vi "Alligator Variables Storage.vi"(6 "Get(F)/Set":bool, 7 "AlliGator Variable":T1=enum."Phasor Plot:Computed", 8 "Error In":errorcluster, 11 "Data in":variant) -> (0 "Error Out":errorcluster, 1 "Default Data out":variant, 3 "Data out":variant)   [LabVIEW 2021, in "AlliGator Globals, Variables & Constants.lvlib"]
doc: "LV2-type global storage of internal AlliGator data and parameters."
uses:
  AlliGator Globals, Variables & Constants.lvlib
  AlliGator Variables List.ctl
  GUI/AlliGator State Indicator.ctl
  Image Profile Window/AlliGator Image Profile Data.ctl
  Image/Image ROI Type.ctl
  Image Profile Window/AlliGator Image Profile Plot Data.ctl
  Graphs/XY Graph/XY Plot Data.ctl
  Action Engine/AlliGator Q Event.ctl
  Source Image/AlliGator Image Loading Options.ctl
  Settings/AlliGator Image Smoothing Options.ctl
  Arrays/Kernel Type.ctl
  Arrays/Smoothing Algorithm.ctl
  Settings/AlliGator Background Subtraction Parameters.ctl
  Source Image/AlliGator Image Binning Options.ctl
  Settings/AlliGator Gates to Keep.ctl
  SwissSPAD/SwissSPAD Live_Image Display Options.ctl
  Files/AlliGator Image Pre-processing Step.ctl
  Files/AlliGator ICCD-specific Information.ctl
  Python Plugins API/AlliGator Python Function Information.ctl
  Python Plugins API/AlliGator Python Function Parameter Definition.ctl
  Python Plugins API/AlliGator Python Function Output Definition.ctl
  Python Plugins API/AlliGator Python Plugin Target Type.ctl
  ROIs/AlliGator Image ROI Event refnum.ctl
  ROIs/AlliGator ROI Manager Actions.ctl
  Source Image/AlliGator Displayed Image.ctl
  Image Profile Window/AlliGator Image Profile Intensity Type.ctl
  Image Profile Window/AlliGator Image Profile Average Intensity Type.ctl
  Image/Box Profile Type.ctl
  Fits/IRF(X)PSED/Decay Fit Parameters & Derived Quantities List v2.ctl
  Phasor/Phasor Harmonic Data.ctl
  Phasor Plot/AlliGator Phasor Harmonic Manager Event Refnum.ctl
  Phasor Plot/AlliGator Phasor Harmonic Manager Actions.ctl
  Phasor Ratio/AlliGator Phasor Plot Reference Points.ctl
  Phasor Plot/AlliGator Phasor Plot Parameters v2.ctl
  Decay Analysis/Decay Preprocessing/AlliGator Decay Preprocessing Options.ctl
  Decay Analysis/Decay Preprocessing/AlliGator Background Subtraction Parameters.ctl
  Decay Analysis/Decay Preprocessing/AlliGator Baseline Subtraction Method.ctl
  Decay Analysis/Decay Preprocessing/AlliGator Decay Preprocessing Parameters.ctl
  Graphs/XY Graph/XY Graph Plot Shift Parameters.ctl
  Graphs/XY Graph/XY Graph Plot Shift Method.ctl
  Settings/AlliGator Low Count Pixels Rejection Options.ctl
  Settings/AlliGator High Count Pixels Rejection Options.ctl
  Settings/AlliGator Gate Arithmetic.ctl
  Phasor Plot/AlliGator Phasor Plot Smoothing Options.ctl
  Phasor Plot/AlliGator Phasor Plot Size.ctl
  Image/Named ROI Description.ctl
  Phasor Calibration/AlliGator Phasor Calibration Options.ctl
  Phasor/Phasor Calibration Type.ctl
  Phasor Calibration/AlliGator Calibration Map Algorithm.ctl
  Fits/IRF(X)PSED/Decay Fit Parameters In List.ctl
  Decay Analysis/Decay Processing/AlliGator Decay Graph Process Plot Target.ctl
  Local Decay Window/AlliGator Local Decay Fit Results.ctl
  GUI/AlliGator Skippable Windows Status.ctl
  Dual-Channel Datasets/AlliGator Dataset Channel.ctl
  Palette/Image Palette Information.ctl
  Image/Image Display Palette Type.ctl
  Image/Image Zoom Factor.ctl
  Phasor/Phasor (g, s).ctl
  Fits/Fit Results (statistics).ctl
  Fits/Non-linear Fitting Method v2.ctl
  Fits/Non-linear Fitting Algorithm.ctl
  Phasor Ratio/AlliGator Phasor Ratio.lvlib
  Image/Image.lvlib
  Palette/Palette.lvlib
  Phasor/Phasor.lvlib
  ROIs/AlliGator ROIs.lvlib
  Fits/Fits.lvlib
  Settings/AlliGator Settings.lvlib
  Decay Analysis/Decay Preprocessing/AlliGator Decay Preprocessing.lvlib
  GUI/AlliGator GUI.lvlib
  Arrays/Arrays.lvlib
  Source Image/AlliGator Source Image.lvlib
  Graphs/XY Graph/XY Graph Add-Ons.lvlib
  Phasor Plot/AlliGator Phasor Plot.lvlib
  Image Profile Window/AlliGator Image Profile Window.lvlib
  Action Engine/AlliGator Action Engine.lvlib
  SwissSPAD/SwissSPAD Live.lvlib
  Python Plugins API/AlliGator Python Plugins.lvlib
  Dual-Channel Datasets/AlliGator Dual-Channel Datasets.lvlib
  Decay Analysis/Decay Processing/AlliGator Decay Processing.lvlib
  Phasor Calibration/AlliGator Phasor Calibration.lvlib
  Files/AlliGator Files.lvlib
  Local Decay Window/AlliGator Local Decay Window.lvlib
panel:
  in  "user event out":refnum<user-event>
  in  "State Indicators":refnum<vi>
  # "see the AlliGator License on the block diagram (Ctrl+E or Window:Show Block Diagram)"
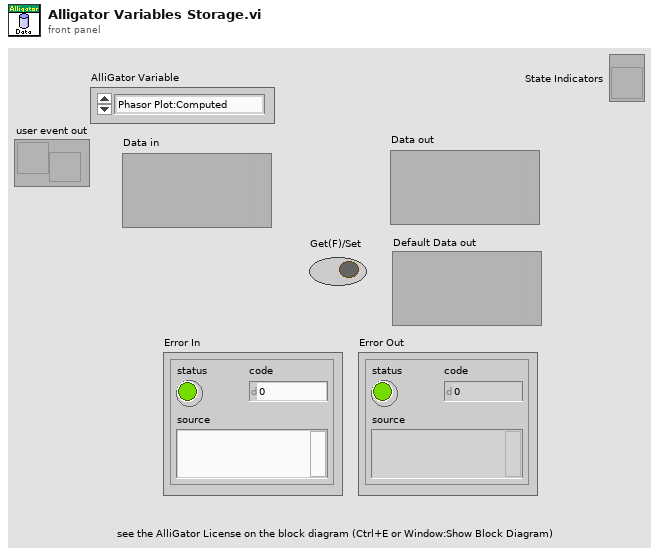
[diagram p1: front panel]
types:
  T1 = typedef "AlliGator Globals, Variables & Constants.lvlib/AlliGator Variables List.ctl" = enum16{"---- GUI ----", "GUI:Initialization Status", "GUI:State Indicators Refnum", "GUI:Original AlliGator Menu Items", "GUI:Current Action Loop State", "GUI:Script in progress", "GUI:Playback", "GUI:Loop Playback", "GUI:Search ROI Used", "GUI:Search ROI", "Decay Graph Max Legend Size", "Intensity Graph Max Legend Size", "Decay Statistics Graph Max Legend Size", "Phasor Graph Max Legend Size", "Phasor Ratio Graph Max Legend Size", "Lifetime Graph Max Legend Size", "---- Files ----", "Files:Export Dataset Frames as Individual Files", "Files:Show Batch Export Help Balloons", "Files:Frames in Dataset", "Files:ptu File Frame Start Indices", "Files:Current Frame in Dataset", "Files:Current Frame Timestamp", "Files:Dataset Loaded", "Files:Dataset Metadata", "Files:Dataset Channel", "Files:Dataset Data Description", "Files:Background Dataset Metadata", "Files:Background Dataset Channel", "Files:Background Dataset Data Description", "Files:Background File Subtraction", "Files:Background File Path", "Files:Background File Pile-up Correction", "Files:Background File Pixel Well Capacity", "Files:Background File Scaling Factor", "Files:Current Dataset Load Settings", "Files:Dataset Path", "Files:ICCD-specific Information", "Files:Macrotime Gate Separation", "------ Python Plugins ------", "Python Plugins:Information", "Python Plugins:Python Session", "Python Plugins:Valid Python Session?", "---- Source Image ----", "Source Image:ROIs", "Source Image:Current ROI", "Source Image:ROI Event Refnum", "X_Source Image Display Range", "X_Source Image Palette Information", "X_Type of Displayed Image", "X_Time Gate Slider", "Source Image:Palette List", "Source Image:Scale", "Source Image:ROI Overlay Color", "Source Image:Overlay to Erase", "Source Image:Is Displayed Image Accumulated", "Source Image:White Light Image Modified", "Source Image:Mask Image Modified", "---- Image Profile Window ----", "Image Profile:Window Event Refnum", "Image Profile:IntensityType", "Image Profile:Intensity Average Type", "Image Profile:Intensity-weighted SDV", "Image Profile:Box Profile Type", "Image Profile:Window Open", "Image Profile:Plotted Fit Parameter", "------ Phasor Graph -------", "Phasor Graph:Show Line", "---- Phasor Plot ---", "Phasor Plot:Parameters Changed", "Phasor Plot:FLI Dataset Modified since last Calculation", "Phasor Harmonics Data", "Selected Phasor Harmonics", "Phasor Harmonic Manager Event Refnum", "Phasor Plot:ROIs", "Phasor Plot:Current ROI", "Phasor Plot:ROI Event Refnum", "Phasor Plot:Image Reference Points", "Phasor Plot:Computed", "Phasor Plot:Palette Information", "Phasor Plot:Palette List", "Phasor Plot:Phasor Ratio Palette Information", "Phasor Plot:Phasor Ratio Palette List", "Phasor Plot:Image Scale", "Phasor Plot:Image Overlay to Erase", "Phasor Plot:Image Elements to Update", "Phasor Plot:Current Calculation Parameters", "Phasor Plot:Current Calibration Options", "Phasor Plot:Reset Cumulated Phasor Plot", "Phasor Plot:Reference 1", "Phasor Plot:Lifetime Reference 1", "Phasor Plot:Reference 1 Frequency", "Phasor Plot:Reference 2", "Phasor Plot:Lifetime Reference 2", "Phasor Plot:Reference 2 Frequency", "---- Decay Analysis ----", "Number of Selected Decays to Fit", "LS Fit Results", "LAR Fit Results", "BS Fit Results", "Last Decay Max - Min", "Best Fit Parameters", "Best Fit Parameter Names", "Actual Size X", "Actual Size Y", "Binning X", "Binning Y", "Actual # Gates", "Dataset Number", "Gates to...", "Gates Skipped", "Gates to keep", "Gate Step", "Gate Separation", "Reversed Gates", "Pile-up Correction", "Pixel Well Capacity", "Background Subtracted", "Background Subtraction Method", "Background Definition Range", "Background File (deprecated)", "Number of Dataset Accumulated", "Array of Accumulated Dataset Paths", "Do Averaged Datasets", "Destination File Path", "Process Plot Target", "Use 1/D as Phasor Frequency", "---- Decay Fit Parameter Map -----", "Decay Fit Parameter Map:Palette Information", "Decay Fit Parameter Map:Palette List", "---- Parameter Map ----", "Parameter Map:Palette Information", "Parameter Map:Palette List", "------- Local Decay Window ---------", "Local Decay Graph Window:Event Refnum", "Local Decay Graph Window:Use normalized IRF for convolution", "----- Miscellaneous ----", "Misc:Skippable Dialog Windows Status"}
  T2 = typedef "AlliGator Action Engine.lvlib/AlliGator Q Event.ctl" = enum16{"---- Files ----", "Files:Set Batch Export Files To Save", "Files:Set Dataset Loading & Pre-processing Options", "Files:Check #Frames in Dataset", "Files:Increment Frame Index", "Files:Open Mask Image", "Files:Open White Light Image", "Files:Open Single Dataset", "Files:New Folder of Folders Selected", "Files:Load File (all Types)_Scriptable", "Files:Move Flattened Series to Folders Series", "Files:Select Folder", "Files:Load FLI Dataset", "Files:Load Swiss SPAD 1 Dataset", "Files:Load Swiss SPAD 2 Dataset", "Files:Load .sdt FLI Dataset", "Files:Load .ptu FLI Dataset", "Files:Load .bin FLI Dataset", "Files:Load Single Gate Image Folder", "Files:Load I/m/phi Dataset (deprecated)", "Files:Load Single Image", "Files:Subtract Background File", "Files:Export FLI Dataset", "Files:Load HDF5 FLI Dataset", "Files:Set Destination File Path", "Files:Save Mask Image", "Files:Batch Conversion", "Files:New Folder Selected", "Files:Close FLI Dataset", "Files:Close FLI Dataset Series", "Files:Close White Light Image", "Files:Close Mask Image", "---- FLI Dataset ----", "FLI Dataset:Channel Arithmetic", "FLI Dataset:Export Average Lifetime Map as ASCII", "FLI Dataset:Export User-Defined Quantity Map as ASCII", "FLI Dataset:Python Function FLI Dataset Event", "FLI Dataset:ROI Analysis", "FLI Dataset:Tilted Logistic Square Gated IRF Characteristics Map", "FLI Dataset:Logistic Square Gated IRF Characteristics Map", "FLI Dataset:Square Gated IRF Characteristics Map", "FLI Dataset:Multi-ROI Single-Pixel Phasor Analysis", "FLI Dataset:Multi-ROI Single-Pixel NLSF Analysis", "FLI Dataset:All ROIs IRF Extraction", "FLI Dataset:All ROIs Decay Fit Non-Interactive (Fast + Individual IRF)", "FLI Dataset:All ROIs Phasor Analysis", "FLI Dataset:All ROIs Decay Fit", "FLI Dataset:Fluorescence Decay Statistics", "FLI Dataset:Update Decay Statistics Graph", "FLI Dataset:Get Decay from ROI", "FLI Dataset:All ROIs Average Lifetimes", "---- FLI Dataset Series ----", "FLI Dataset Series:Sum All Datasets in Series", "FLI Dataset Series:Add Dataset to Accumulated Dataset", "FLI Dataset Series:Display Accumulated Dataset", "FLI Dataset Series:Clear Dataset Series Sum", "FLI Dataset Series:Time-Series Analysis (NLSF)", "FLI Dataset Series:Time-Series Analysis (Phasor)", "---- Image ----", "Image:Update Image Profile Plots", "Image:Image Histogram Cursor Move", "Image:Image Histogram", "Image:Image Contrast", "Image:Set Image Histogram Cursor Move Flag", "Image:Clear Image Overlay", "Image:Use ROI as Search Area", "Image:Set ROI Diameter", "Image:Save Image Data as TIFF", "Image:Save Displayed Image with Overlay", "Image:Save Image Overlay Only", "Image:Save Image as Hot Pixel Mask", "Image:Change Source Image Color Palette", "Image:Copy Image to Clipboard", "Image:Source Image ROI Selection", "Image:Delete All ROIs", "Image:Delete All Unselected ROIs", "Image:Delete ROI", "Image:Merge All ROIs", "Image:Store ROI", "Image:Source Image ROI Storage", "Image:Export ROI Description to Notebook", "Image:Save ROI", "Image:Load ROI", "Image:Paste ROI Definition", "Image:Clear ROI", "Image:Identify ROIs in Mask Image", "Image:Create Complementary ROI", "Image:Create Contour ROI", "Image:Create ROI(s) from Pixels with Peak above Min_Scriptable", "Image:Create ROI(s) from Pixels with Intensity above Min_Scriptable", "Image:Compute ROI Statistics", "Image:Delete ROI(s) based on ROI Characteristics", "Image:Create ROI Grid", "Image:ROI to Individual Pixel ROIs", "Image:Python Function Source Image Event", "Image:Show Phasor Calibration Map ROI Centers", "Image:Convert ROI to Mask Image", "Image:Mouse Move", "Image:Mouse Up", "Image:Set Source Image Mouse Move Flag", "Image:Add Scale Bar Overlay", "Image:Delete Existing ROIs Option", "Image:Overlay ROI Median", "Image:Check Current ROI", "---- Decay ----", "Decay:Clear IRF/Reference Plot", "Decay:Clear Local IRFs", "Decay:Add Decay to Graph", "Decay:Smoothen Plot", "Decay:Smoothen Plot Tail", "Decay:Average Selected Plots", "Decay:Extract IRF", "Decay:Optimal IRF Extraction", "Decay:Threshold IRF", "Decay:Fit to Model IRF", "Decay:Fit IRF to Square Gate", "Decay:Fit IRF to Logistic Square Gate", "Decay:Fit IRF to Tilted Logistic Square Gate", "Decay:Create Bounding Cursors Set", "Decay:Export Bounding Cursors Definition to Notebook", "Decay:Denoise Plot", "Decay:Compute Cumulative Function", "Decay:Use as Reference Decay", "Decay:Show Reference Decay/IRF", "Decay:Extrapolate Decay", "Decay:Create Head & Tail Bounding Cursors", "Decay:Store Cursor-defined Head & Tail Fractions", "Decay:Rebin Plot", "Decay:1-Normalize Decay", "Decay:[0-1]-Normalize Plot", "Decay:Straighten Decay", "Decay:Shift Decay", "Decay:Fold Decay", "Decay:Fit Decay", "Decay:Global Fit of Selected Decays", "Decay:Post Global Fit Script", "Decay:Add Global Fit Parameters to Graph", "Decay:Add Decay Parameter(s) to Plot (Graph)", "Decay:Export Decay to Phasor Graph", "Decay:Plot Decay Shifts", "Decay:Compute Average Lifetime", "Decay:Plot Convolution", "Decay:Graph Tip Strip Update", "---- Decay Statistics ----", "Decay Statistics:Tip Strip Update", "---- Intensity Time Trace ----", "Intensity Time Trace:Use File Timestamp", "Intensity Time Trace:Load Intensity Corrections File", "Intensity Time Trace:Clear Intensity Corrections File", "Intensity Time Trace:Tip Strip Update", "---- Phasor Plot ----", "Phasor Plot:Build Phasor Plot", "Phasor Plot:Change Phasor Plot Color Palette", "Phasor Plot:Adjust Phasor Plot Display Range", "Phasor Plot:Highlight Image ROI in Phasor Plot", "Phasor Plot:Save Phasor Plot Image with Overlay", "Phasor Plot:Export Complex Phasor Map", "Phasor Plot:Export Phasor Ratio Map", "Phasor Plot:Export Average Lifetime Map", "Phasor Plot:Compute Phase Lifetime Histogram", "Phasor Plot:Compute Phasor Ratio Histogram", "Phasor Plot:Compute Phase Lifetime vs Intensity Scatter Plot", "Phasor Plot:Weber 2-Component Decomposition", "Phasor Plot:Update Phasor Color Map Vertices", "Phasor Plot:Clear Phasor Overlay", "Phasor Plot:Use Segment Extremities as References", "Phasor Plot:Use UC/Segment Intersections as References", "Phasor Plot:Use UC/Principal Axis Intersections as References", "Phasor Plot:Use UC/Linear Fit Intersections as References", "Phasor Plot:Update Phasor Plot Reference", "Phasor Plot:Show Local Phasor Info in Phasor Plot", "Phasor Plot:Update Phasor Plot State", "Phasor Plot:Phasor Plot ROI Storage", "Phasor Plot:Phasor Plot ROI Selection", "Phasor Plot:Python Function Phasor Plot Event", "Phasor Plot:Overlay Phasor ROI, Ratio or Map in Source Image", "Phasor Plot:Compute Decay of Selected Phasors", "Phasor Plot:Phasor at Image Pixel", "Phasor Plot:Mouse Move", "Phasor Plot:Mouse Up", "Phasor Plot:Display Range Mouse Move", "Phasor Plot:Set Mouse Move Flag", "---- Phasor Graph ----", "Phasor Graph:Calibrated Phasor Map Series", "Phasor Graph:Whole Image Phasor Scatter Plot (deprecated)", "Phasor Graph:Get Phasor Value", "Phasor Graph:Create New Phasor Plot Dialog", "Phasor Graph:Update Last Phasor Value", "Phasor Graph:Update Phasor (m, phi)", "Phasor Graph:Remove Single Phasor from Plot", "Phasor Graph:Add Single Phasor to Plot", "Phasor Graph:Remove Phasor Plot", "Phasor Graph:Remove Selected Phasor Plots", "Phasor Graph:Clear Phasor Data", "Phasor Graph:Clear Phasor Graph", "Phasor Graph:Cursor Move", "Phasor Graph:Draw Cursor Connecting Line", "Phasor Graph:Clear Cursor Connecting Line", "Phasor Graph:Find UC Intersection", "Phasor Graph:Use UC/Cursor-Defined Line Intersections", "Phasor Graph:Use Selected Plots Fitted Line/UC Intersections", "Phasor Graph:Use Selected Plots Principal Axis/UC Intersections", "Phasor Graph:Show Single Phasor", "Phasor Graph:Save Single Phasor Plot", "Phasor Graph:Save All Phasor Plots", "Phasor Graph:Load Phasor Plot(s)", "Phasor Graph:Phasor Multiplication", "Phasor Graph:Compute Average Phasor", "Phasor Graph:Compute Multiple Average Phasors (Selected Plots)", "Phasor Graph:Export Single Phasor Plot Phase Lifetimes", "Phasor Graph:Phase Lifetime Trajectory", "Phasor Graph:Phase Lifetime vs Intensity Scatter Plot (deprecated)", "Phasor Graph:Parameter 2 vs Parameter 1 Scatter Plot", "Phasor Graph:Use Cursor n Location", "Phasor Graph:Set Reference n to Current Phase Lifetime Value", "Phasor Graph:Set Reference n to Lifetime Value", "Phasor Graph:Set Cursor n Location", "Phasor Graph:Save Phasor Graph Image", "Phasor Graph:Update SEPL Plot", "Phasor Graph:Export Single Phasor Plot Data", "Phasor Graph:Export Selected Phasor Plots Data", "Phasor Graph:Python Function Phasor Graph Event", "Phasor Graph:Tip Strip Update", "---- Calibration ----", "Calibration:Set Calibration Type", "Calibration:Load/Save Phasor Calibration", "Calibration:Load/Save Phasor Calibration Series", "Calibration:Load/Save Phasor Calibration Map", "Calibration:Use as Calibration", "Calibration:Compute Optimal Calibration from Phasor References", "Calibration:Clear Phasor Calibration", "Calibration:Single Phasor Calibration Information", "Calibration:Use as Calibration Series", "Calibration:Use as Calibration Map", "Calibration:Clear Calibration Series", "Calibration:Phasor Calibration Series Information", "Calibration:Clear Calibration Map", "Calibration:Phasor Calibration Map Information", "Calibration:Apply Phasor Calibration", "Calibration:Update Single Plot Calibration", "Calibration:Update Multiple Plots Calibration", "Calibration:Clear Single Plot Calibration", "Calibration:Clear All Plots Calibrations", "Calibration:Clear Plot(s) Calibration(s)?", "Calibration:Phasor Calibration Maps (# Gates Series)", "---- Phasor Ratio ----", "Phasor Ratio:Clear Reference n", "Phasor Ratio:Toggle Selected Plot(s)  Lock to Reference 1", "Phasor Ratio:Use as Reference n", "Phasor Ratio:Send Reference n to Notebook", "Phasor Ratio:Toggle Selected Plot(s)  Lock to Reference 2", "Phasor Ratio:Compute Phasor Ratio at Mouse Location", "Phasor Ratio:Compute Phasor Plot's Average Phasor Ratio", "Phasor Ratio:Compute Time-Series Phasor Ratios", "Phasor Ratio:Fit Line to Phasor Ratio Plot", "Phasor Ratio:Save References", "Phasor Ratio:Load References", "Phasor Ratio:Update Phasor Reference 1", "Phasor Ratio:Update Phasor Reference 2", "Phasor Ratio:Move Cursor n to Reference n", "Phasor Ratio:Use as Phasor Reference 1 Lifetime", "Phasor Ratio:Use as Phasor Reference 2 Lifetime", "Phasor Ratio:Export Phasor Ratio Map as ASCII", "Phasor Ratio:Tip Strip Update", "---- Lifetime & Other Parameters Graph ----", "Lifetime:Tip Strip Update", "---- Decay Fit Parameter Map ----", "Decay Fit Parameter Map:Export ROI NLSF Data as ASCII", "Decay Fit Parameter Map:Set Decay Fit Parameter Map Selection", "Decay Fit Parameter Map:Build Decay Fit Parameter Map", "Decay Fit Parameter Map:Change Decay Fit Parameter Map Color Palette", "Decay Fit Parameter Map:Export Decay Fit Parameter Map Data as ASCII", "Decay Fit Parameter Map:Export All Decay Fit Parameter Maps Data as ASCII", "Decay Fit Parameter Map:Selected Parameter Scatterplot", "Decay Fit Parameter Map:Parameter 2 vs Parameter 1 Scatterplot", "Decay Fit Parameter Map:Save Decay Fit Parameter Map Image", "Decay Fit Parameter Map:Save-Load IRFs & Fit Data", "Decay Fit Parameter Map:Update Local Decay Plots", "Decay Fit Parameter Map:Python Function Decay Fit Parameters Map Event", "Decay Fit Parameter Map:Overlay Decay Fit Parameter Map in Source Image", "Decay Fit Parameter Map:Selected Parameter vs Intensity Scatterplot", "Decay Fit Parameter Map:Mouse Up", "Decay Fit Parameter Map:Display Range Mouse Move", "---- Parameter Map ----", "Parameter Map:Export ROI Parameters Data as ASCII", "Parameter Map:Delete Parameter Map Set", "Parameter Map:Update Parameter List", "Parameter Map:Build Parameter Map", "Parameter Map:Change Parameter Map Color Palette", "Parameter Map:Export Parameter Map Data as ASCII", "Parameter Map:Export All Parameter Maps Data as ASCII", "Parameter Map:Selected Parameter Scatterplot", "Parameter Map:Parameter 2 vs Parameter 1 Scatterplot", "Parameter Map:Selected Parameter vs Intensity Scatterplot", "Parameter Map:Save Parameter Map Image", "Parameter Map:Save-Load IRFs & Parameter Maps (TODO)", "Parameter Map:Set Parameter Map Selection", "Parameter Map:Python Function Parameter Map Event", "Parameter Map:Overlay Parameter Map in Source Image", "Parameter Map:Update Local Decay Plots", "Parameter Map:Mouse Up", "Parameter Map:Display Range Mouse Move", "---- Generic Graph ----", "Generic Graph:Generic XY Graph Event", "Generic Graph:Python Function XY Graph Event", "Generic Graph:New Plot", "Generic Graph:Save Plot", "Generic Graph:XY Plot Histogram", "Generic Graph:Set XY Graph Plot Name", "Generic Graph:Set Last Cursor Style", "Generic Graph:Tip Strip Update", "---- GUI ----", "GUI:Start Script", "GUI:Type of Displayed Image Changed", "GUI:Gate Image Slide Changed", "GUI:Show Busy Icon", "GUI:Show Busy Icon & Abort Button", "GUI:Hide Busy Icon", "GUI:Hide Busy Icon & Abort Button", "GUI:Abort", "GUI:End Script", "GUI:Start Timing", "GUI:End Timing", "GUI:Set State Indicator", "GUI:Send Parameters JSON Strings to Clipboard", "GUI:Set Gate Step", "GUI:Idle", "GUI:Initialization", "GUI:Quit", "GUI:Increment Dataset Index", "GUI:Set Dataset Index to -1", "GUI:Time Series Slider Moved", "GUI:Time Series Slider Changed", "GUI:Toggle Playback or Loop", "GUI:Playback Script", "GUI:Set Phasor Frequency", "GUI:Open Window", "GUI:Start Test Script", "GUI:End Test Script", "DEBUG"}
  T3 = typedef "ROI Descriptor" = cluster{"Global Rectangle":i32[], "Contours":cluster{"ID":enum32{"External", "Internal"}, "Type":u32, "Coordinates":i32[]}[]}
  T4 = typedef "AlliGator Dual-Channel Datasets.lvlib/AlliGator Dataset Channel.ctl" = enum16{"G2", "INT"}
  T5 = typedef "AlliGator Source Image.lvlib/AlliGator Image Loading Options.ctl" = cluster{"Pixel Well Capacity":u32, "Pile-up Correction":bool, "Gate Step":i32, "Image Smoothing Options":T6, "Gates to Skip":T9, "File Background Subtraction":bool, "Background File Path":path, "Image Binning Options":T10, "# Gates":u32, "Gates to Keep":T11, "Define Gates to":bool, "Hot Pixel Removal":T12, "Dataset Scaling Factor":dbl, "Image Pre-processing Steps":T13[]}
  T6 = typedef "AlliGator Settings.lvlib/AlliGator Image Smoothing Options.ctl" = cluster{"Use Image Smoothing":bool, "Kernel Type":T7, "Bin":i32, "Algorithm":T8}
  T7 = typedef "Arrays.lvlib/Kernel Type.ctl" = enum16{"Uniform", "Bilinear", "Gaussian"}
  T8 = typedef "Arrays.lvlib/Smoothing Algorithm.ctl" = enum16{"Rapid", "Thorough"}
  T9 = typedef "AlliGator Settings.lvlib/AlliGator Background Subtraction Parameters.ctl" = cluster{"Start":u32, "End":u32}
  T10 = typedef "AlliGator Source Image.lvlib/AlliGator Image Binning Options.ctl" = cluster{"Use Image Binning":bool, "X Bin":i32, "Y Bin":i32}
  T11 = typedef "AlliGator Settings.lvlib/AlliGator Gates to Keep.ctl" = cluster{"First":u32, "Last":u32}
  T12 = typedef "SwissSPAD Live.lvlib/SwissSPAD Live_Image Display Options.ctl" = cluster{"Remove Screamers":bool, "Delta":sgl, "Equalize Histogram":bool, "Percentile":sgl, "Hot Pixel Mask Image":path, "Use Hot Pixel Mask":bool}
  T13 = typedef "AlliGator Files.lvlib/AlliGator Image Pre-processing Step.ctl" = enum16{"Remove Screamers", "Pile-up Correction", "Binning", "Smoothing", "Rescaling", "Dead Left Column Correction"}
  T14 = typedef "AlliGator Files.lvlib/AlliGator ICCD-specific Information.ctl" = cluster{"V MCP":dbl[unit], "X Hardware Binning":dbl, "Y Hardware Binning":dbl, "Gate Image Integration":dbl[unit], "Laser Power":dbl[unit]}
  T15 = typedef "AlliGator Python Plugins.lvlib/AlliGator Python Function Information.ctl" = cluster{"Script Path":path, "Function Name":string, "Function Parent Menu":string, "API Version":string, "Function Input Parameters":T16[], "Function Outputs":T17[], "Function Doc String":string, "Function Display Name":string, "Function Target Type":T18, "Function Target Window":string, "Parent Menu Location":string, "Item Menu Tag":string, "Is preceded by Separator":bool}
  T16 = typedef "AlliGator Python Plugins.lvlib/AlliGator Python Function Parameter Definition.ctl" = cluster{"Parameter Name":string, "Parameter Type":string, "Parameter Description":string}
  T17 = typedef "AlliGator Python Plugins.lvlib/AlliGator Python Function Output Definition.ctl" = cluster{"Output Type":string, "Output Destination":string}
  T18 = typedef "AlliGator Python Plugins.lvlib/AlliGator Python Plugin Target Type.ctl" = enum16{"Undefined", "Window Menu", "Object Menu"}
  T19 = typedef "Image.lvlib/Named ROI Description.ctl" = cluster{"ROI Descriptor":T3, "ROI Name":string, "Overlay Color":u32}
  T20 = typedef "AlliGator ROIs.lvlib/AlliGator Image ROI Event refnum.ctl" = refnum<user-event>
  T21 = typedef "Palette.lvlib/Image Palette Information.ctl" = cluster{"Palette Name [# Colors,int?,inv?]":string, "Palette Type":T22, "Palette Colors":u32[], "Interpolate?":bool}
  T22 = typedef "Image.lvlib/Image Display Palette Type.ctl" = u32
  T23 = typedef "AlliGator Source Image.lvlib/AlliGator Displayed Image.ctl" = enum16{"Single Gate", "Sum of All Gates", "Max of All Gates", "Min of All Gates", "-", "White Ligth Image", "Mask Image"}
  T24 = typedef "Image.lvlib/Image Zoom Factor.ctl" = enum16{"Zoom to Fit", "Zoom to Fit (Keep Aspect Ratio)", "Other Zoom Factor"}
  T25 = typedef "AlliGator Image Profile Window.lvlib/AlliGator Image Profile Intensity Type.ctl" = enum16{"Raw Data", "Displayed Image", "Background-subtracted"}
  T26 = typedef "AlliGator Image Profile Window.lvlib/AlliGator Image Profile Average Intensity Type.ctl" = enum16{"Integrated Intensity", "Average Intensity", "Intensity-weighted Average Intensity"}
  T27 = typedef "Image.lvlib/Box Profile Type.ctl" = enum16{"Full Width", "Half Width"}
  T28 = typedef "Fits.lvlib/Decay Fit Parameters & Derived Quantities List v2.ctl" = enum16{"Offset", "Baseline", "A_1", "tau_1", "A_2", "tau_2", "<tau>_a", "f1_a", "f2_a", "<tau>_i", "f1_i", "f2_i", "-", "R^2", "Chi^2"}
  T29 = typedef "Phasor.lvlib/Phasor Harmonic Data.ctl" = cluster{"Phasor Harmonic Name":string, "Phasor Plot Settings Checksum":u64, "Phasor Frequency":dbl[unit], "Base Frequency":dbl[unit], "Harmonic Order":u8, "Phasor Plot Parameters":string, "Phasor Array [[CSG]]":csg[][], "Dataset File Path":path}
  T30 = typedef "AlliGator Phasor Plot.lvlib/AlliGator Phasor Harmonic Manager Event Refnum.ctl" = refnum<user-event>
  T31 = typedef "AlliGator Phasor Ratio.lvlib/AlliGator Phasor Plot Reference Points.ctl" = cluster{"O_h":dbl, "O_v":dbl, "1_h":dbl, "1_v":dbl}
  T32 = typedef "AlliGator Phasor Plot.lvlib/AlliGator Phasor Plot Parameters v2.ctl" = cluster{"Phasor Frequency":dbl[unit], "Decay Preprocessing Options & Parameters":T33, "FLI Dataset Modified":bool, "Source Image Settings":cluster{"Low Count Pixels Rejection Options":T39, "High Count Pixels Rejection Options":T40}, "Data Information":cluster{"Gate Width":dbl[unit], "Gate Separation":dbl[unit], "Step (Gate Separation)":i32, "Laser Period":dbl[unit], "SYNC Period":dbl[unit], "Channel Name":u16, "Channel Arithmetic":T41, "Pile-up Correction":bool, "Pixel Well Capacity":u32, "Dataset Scaling Factor":dbl}, "Phasor Plot":cluster{"Phasor Plot Smoothing Options":T42, "Phasor Plot Size":T43, "Selected Image ROI(s)":bool, "All Image ROIs":bool, "Selected Source Image ROI":i32, "Source Image ROIs":T19[]}}
  T33 = typedef "AlliGator Decay Preprocessing.lvlib/AlliGator Decay Preprocessing Options.ctl" = cluster{"Background Subtraction Parameters":T34, "Decay Preprocessing Parameters":T36, "Preprocessing Steps Order":string[]}
  T34 = typedef "AlliGator Decay Preprocessing.lvlib/AlliGator Background Subtraction Parameters.ctl" = cluster{"Background Definition Range":cluster{"Min Gate":dbl[unit], "Max Gate":dbl[unit]}, "Baseline Subtraction Method":T35, "Background Subtraction?":bool, "Background File":path, "Background Constant":dbl, "Background Scaling Factor":dbl, "Background Pile-up Correction":bool, "Background Pixel Well Capacity":u32}
  T35 = typedef "AlliGator Decay Preprocessing.lvlib/AlliGator Baseline Subtraction Method.ctl" = enum16{"Mean", "Min", "Square Gated Single-Exponential", "File", "Constant"}
  T36 = typedef "AlliGator Decay Preprocessing.lvlib/AlliGator Decay Preprocessing Parameters.ctl" = cluster{"Background Subtraction":bool, "Straighten Decay":bool, "Reverse Gates":bool, "1-Normalized Decay":bool, "Smoothen Decay":bool, "Smoothing Parameter":dbl, "Shift Decay":bool, "Decay Shift Parameters":T37, "Extrapolate Decay":bool, "Additional Points":u32, "Head Fraction":dbl, "Pixel-Normalize Decay":bool, "Use Periodicity":bool, "Use Cursors":bool, "Tail Fraction":dbl, "Use Decay Pre-Processing":bool, "Fold Decay":bool, "# Folds":u32, "[0-1]-Normalized Decay":bool}
  T37 = typedef "XY Graph Add-Ons.lvlib/XY Graph Plot Shift Parameters.ctl" = cluster{"Type":T38, "Shift":dbl[unit], "Threshold":dbl, "Rotate":bool}
  T38 = typedef "XY Graph Add-Ons.lvlib/XY Graph Plot Shift Method.ctl" = enum16{"Default", "CFD", "Threshold", "Cross-Correlation"}
  T39 = typedef "AlliGator Settings.lvlib/AlliGator Low Count Pixels Rejection Options.ctl" = cluster{"Background Low Threshold Factor":dbl, "Fixed Low Background Threshold":dbl, "Reject Low Count Pixels":bool, "Low Percentile":dbl}
  T40 = typedef "AlliGator Settings.lvlib/AlliGator High Count Pixels Rejection Options.ctl" = cluster{"Background High Threshold Factor":dbl, "Fixed High Background Threshold":dbl, "Reject High Count Pixels":bool, "High Percentile":dbl}
  T41 = typedef "AlliGator Settings.lvlib/AlliGator Gate Arithmetic.ctl" = enum16{"None", "INT-G2", "G2/INT*<INT>", "(1 - G2/INT)*<INT>"}
  T42 = typedef "AlliGator Phasor Plot.lvlib/AlliGator Phasor Plot Smoothing Options.ctl" = cluster{"Use Phasor Plot Smoothing":bool, "Kernel Type":T7, "Bin":i32, "Algorithm":T8}
  T43 = typedef "AlliGator Phasor Plot.lvlib/AlliGator Phasor Plot Size.ctl" = cluster{"H":i32, "V":i32, "Margin":dbl}
  T44 = typedef "AlliGator Phasor Calibration.lvlib/AlliGator Phasor Calibration Options.ctl" = cluster{"Phasor Frequency":dbl[unit], "Phasor Calibration":cluster{"Calibration Lifetime":dbl[unit], "Calibration Type":T45, "Calibration Map Algorithm":T46, "Use Backup Calibration if needed":bool, "Backup Calibration Type":enum16{"Single Calibration", "Nearest Valid Calibration"}}}
  T45 = typedef "Phasor.lvlib/Phasor Calibration Type.ctl" = enum16{"None", "Single Phasor", "Phasor Series", "Phasor Map"}
  T46 = typedef "AlliGator Phasor Calibration.lvlib/AlliGator Calibration Map Algorithm.ctl" = enum16{"Simple Search", "Min Distance"}
  T47 = typedef "Phasor.lvlib/Phasor (g, s).ctl" = cluster{"g":dbl, "s":dbl}
  T48 = typedef "Fits.lvlib/Fit Results (statistics).ctl" = cluster{"Chi2/DOF":dbl, "R2":dbl, "RMSE":dbl, "Fitting Method":T49, "Fitting Algorithm":T50}
  T49 = typedef "Fits.lvlib/Non-linear Fitting Method v2.ctl" = enum16{"Least Square", "Least Absolute Residual", "Bisquare", "MLE", "-", "Best of All"}
  T50 = typedef "Fits.lvlib/Non-linear Fitting Algorithm.ctl" = enum16{"Levenberg-Marquardt", "Trust-Region Dogleg"}
  T51 = typedef "Fits.lvlib/Decay Fit Parameters In List.ctl" = enum16{"Offset", "Baseline", "A_1", "tau_1", "A_2", "tau_2"}
  T52 = cluster{"Min Gate":dbl[unit], "Max Gate":dbl[unit]}
  T53 = typedef "AlliGator Decay Processing.lvlib/AlliGator Decay Graph Process Plot Target.ctl" = enum16{"Single Plot", "Selected Plots", "All Plots"}
  T54 = typedef "AlliGator GUI.lvlib/AlliGator Skippable Windows Status.ctl" = cluster{"Dialog Window Name":string, "Is skipped":bool}
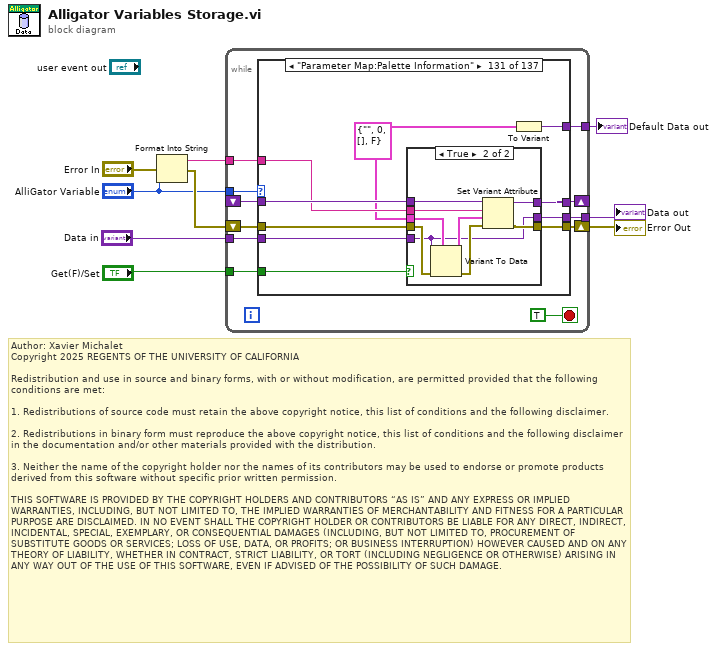
[diagram p0: block diagram]
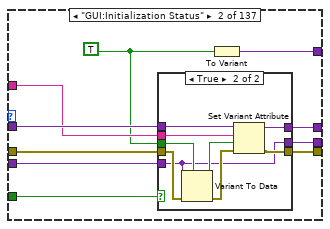
[diagram p3: hidden frame]
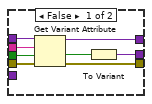
[diagram p4: hidden frame]
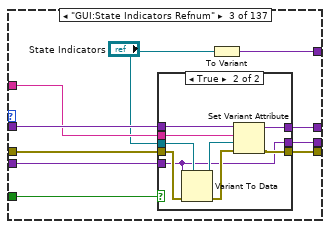
[diagram p5: hidden frame]
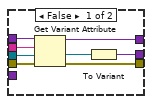
[diagram p6: hidden frame]
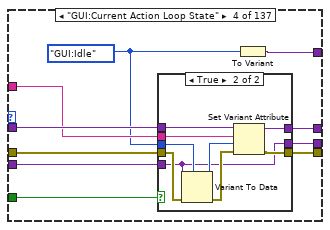
[diagram p7: hidden frame]
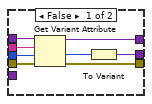
[diagram p8: hidden frame]
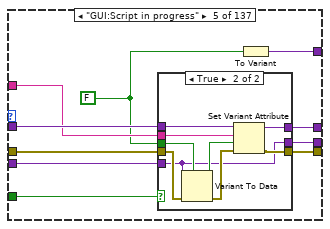
[diagram p9: hidden frame]
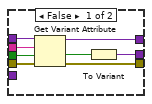
[diagram p10: hidden frame]
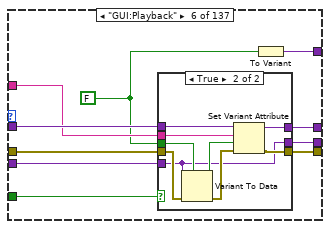
[diagram p11: hidden frame]
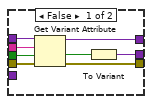
[diagram p12: hidden frame]
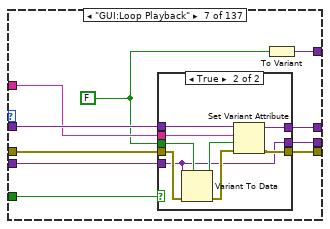
[diagram p13: hidden frame]
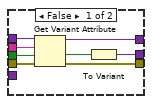
[diagram p14: hidden frame]
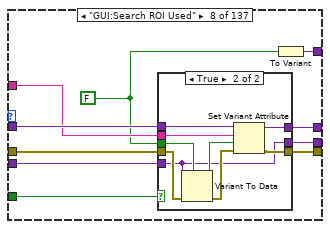
[diagram p15: hidden frame]
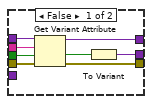
[diagram p16: hidden frame]
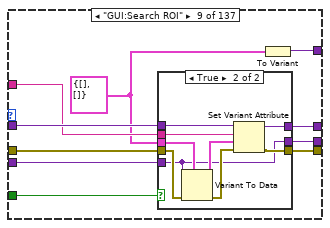
[diagram p17: hidden frame]
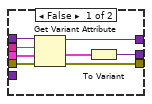
[diagram p18: hidden frame]
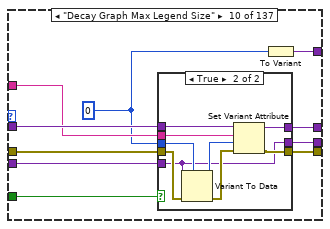
[diagram p19: hidden frame]
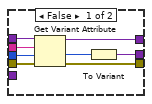
[diagram p20: hidden frame]
diagram:
  # "Author: Xavier Michalet\nCopyright 2025 REGENTS OF THE UNIVERSITY OF CALIFORNIA\n\nRedistribution and use in source and binary forms, with or without modification, are permitted provided that the following conditions are met:\n\n1. Redistributions of source code must retain the above copyright notice, this list of conditions and the following disclaimer.\n\n2. Redistributions in binary form must reproduce the above copyright notice, this list of conditions and the following disclaimer in the documentation and/or other materials provided with the distribution.\n\n3. Neither the name of the copyright holder nor the names of its contributors may be used to endorse or promote products derived from this software without specific prior written permission.\n\nTHIS SOFTWARE IS PROVIDED BY THE COPYRIGHT HOLDERS AND CONTRIBUTORS “AS IS” AND ANY EXPRESS OR IMPLIED WARRANTIES, INCLUDING, BUT NOT LIMITED TO, THE IMPLIED WARRANTIES OF MERCHANTABILITY AND FITNESS FOR A PARTICULAR PURPOSE ARE DISCLAIMED. IN NO EVENT SHALL THE COPYRIGHT HOLDER OR CONTRIBUTORS BE LIABLE FOR ANY DIRECT, INDIRECT, INCIDENTAL, SPECIAL, EXEMPLARY, OR CONSEQUENTIAL DAMAGES (INCLUDING, BUT NOT LIMITED TO, PROCUREMENT OF SUBSTITUTE GOODS OR SERVICES; LOSS OF USE, DATA, OR PROFITS; OR BUSINESS INTERRUPTION) HOWEVER CAUSED AND ON ANY THEORY OF LIABILITY, WHETHER IN CONTRACT, STRICT LIABILITY, OR TORT (INCLUDING NEGLIGENCE OR OTHERWISE) ARISING IN ANY WAY OUT OF THE USE OF THIS SOFTWARE, EVEN IF ADVISED OF THE POSSIBILITY OF SUCH DAMAGE."
  n1 = Format Into String(error in="Error In", "AlliGator Variable") -> (resulting string=w8:string, error out=w5:errorcluster)  [unwired: 2 in]
  n2 = while {
    tunnel: "Get(F)/Set" -> [w12]
    tunnel: w8 -> [w19]
    shift-right: [w17] -> _
    shift-left: _ -> [w18]
    tunnel: "Data in" -> [w11]
    tunnel: [w14] -> w3
    tunnel: "AlliGator Variable" -> [w13]
    tunnel: [w10] -> w1
    shift-right: [w15] -> w4
    shift-left: w5 -> [w16]
    stop <- TRUE stop-if-true
    n3 = case shown="\"Parameter Map:Palette Information\"" w13 {
      tunnel: w18 -> [w23 w33 w60 w87 w114 w141 w168 w195 w222 w249 w276 w303 w330 w357 w384 w402 w414 w441 w468 w495 w522 w549 w576 w603 w630 w657 w684 w711 w738 w765 w792 w819 w846 w873 w900 w927 w954 w981 w999 w1011 w1038 w1065 w1085 w1095 w1122 w1149 w1176 w1203 w1230 w1257 w1284 w1311 w1338 w1365 w1392 w1419 w1446 w1464 w1476 w1503 w1530 w1557 w1584 w1611 w1638 w1656 w1668 w1688 w1698 w1725 w1752 w1779 w1806 w1833 w1860 w1887 w1914 w1941 w1968 w1995 w2022 w2049 w2076 w2103 w2130 w2157 w2184 w2211 w2238 w2265 w2292 w2319 w2346 w2373 w2393 w2403 w2430 w2457 w2484 w2511 w2538 w2565 w2592 w2619 w2646 w2673 w2700 w2727 w2754 w2781 w2808 w2835 w2862 w2889 w2916 w2943 w2970 w2997 w3024 w3051 w3078 w3105 w3132 w3159 w3186 w3213 w3231 w3243 w3270 w3288 w3300 w3327 w3345 w3357 w3384 w3402 w3414]
      tunnel: w19 -> [_ w32 w59 w86 w113 w140 w167 w194 w221 w248 w275 w302 w329 w356 w383 _ w413 w440 w467 w494 w521 w548 w575 w602 w629 w656 w683 w710 w737 w764 w791 w818 w845 w872 w899 w926 w953 w980 _ w1010 w1037 w1064 _ w1094 w1121 w1148 w1175 w1202 w1229 w1256 w1283 w1310 w1337 w1364 w1391 w1418 w1445 _ w1475 w1502 w1529 w1556 w1583 w1610 w1637 _ w1667 _ w1697 w1724 w1751 w1778 w1805 w1832 w1859 w1886 w1913 w1940 w1967 w1994 w2021 w2048 w2075 w2102 w2129 w2156 w2183 w2210 w2237 w2264 w2291 w2318 w2345 w2372 _ w2402 w2429 w2456 w2483 w2510 w2537 w2564 w2591 w2618 w2645 w2672 w2699 w2726 w2753 w2780 w2807 w2834 w2861 w2888 w2915 w2942 w2969 w2996 w3023 w3050 w3077 w3104 w3131 w3158 w3185 w3212 _ w3242 w3269 _ w3299 w3326 _ w3356 w3383 _ w3413]
      tunnel: w16 -> [w22 w31 w58 w85 w112 w139 w166 w193 w220 w247 w274 w301 w328 w355 w382 w404 w412 w439 w466 w493 w520 w547 w574 w601 w628 w655 w682 w709 w736 w763 w790 w817 w844 w871 w898 w925 w952 w979 w1001 w1009 w1036 w1063 w1084 w1093 w1120 w1147 w1174 w1201 w1228 w1255 w1282 w1309 w1336 w1363 w1390 w1417 w1444 w1466 w1474 w1501 w1528 w1555 w1582 w1609 w1636 w1658 w1666 w1687 w1696 w1723 w1750 w1777 w1804 w1831 w1858 w1885 w1912 w1939 w1966 w1993 w2020 w2047 w2074 w2101 w2128 w2155 w2182 w2209 w2236 w2263 w2290 w2317 w2344 w2371 w2392 w2401 w2428 w2455 w2482 w2509 w2536 w2563 w2590 w2617 w2644 w2671 w2698 w2725 w2752 w2779 w2806 w2833 w2860 w2887 w2914 w2941 w2968 w2995 w3022 w3049 w3076 w3103 w3130 w3157 w3184 w3211 w3233 w3241 w3268 w3290 w3298 w3325 w3347 w3355 w3382 w3404 w3412]
      tunnel: [w22 w30 w57 w84 w111 w138 w165 w192 w219 w246 w273 w300 w327 w354 w381 w404 w411 w438 w465 w492 w519 w546 w573 w600 w627 w654 w681 w708 w735 w762 w789 w816 w843 w870 w897 w924 w951 w978 w1001 w1008 w1035 w1062 w1084 w1092 w1119 w1146 w1173 w1200 w1227 w1254 w1281 w1308 w1335 w1362 w1389 w1416 w1443 w1466 w1473 w1500 w1527 w1554 w1581 w1608 w1635 w1658 w1665 w1687 w1695 w1722 w1749 w1776 w1803 w1830 w1857 w1884 w1911 w1938 w1965 w1992 w2019 w2046 w2073 w2100 w2127 w2154 w2181 w2208 w2235 w2262 w2289 w2316 w2343 w2370 w2392 w2400 w2427 w2454 w2481 w2508 w2535 w2562 w2589 w2616 w2643 w2670 w2697 w2724 w2751 w2778 w2805 w2832 w2859 w2886 w2913 w2940 w2967 w2994 w3021 w3048 w3075 w3102 w3129 w3156 w3183 w3210 w3233 w3240 w3267 w3290 w3297 w3324 w3347 w3354 w3381 w3404 w3411] -> w15
      tunnel: [w21 w29 w56 w83 w110 w137 w164 w191 w218 w245 w272 w299 w326 w353 w380 w403 w410 w437 w464 w491 w518 w545 w572 w599 w626 w653 w680 w707 w734 w761 w788 w815 w842 w869 w896 w923 w950 w977 w1000 w1007 w1034 w1061 w1083 w1091 w1118 w1145 w1172 w1199 w1226 w1253 w1280 w1307 w1334 w1361 w1388 w1415 w1442 w1465 w1472 w1499 w1526 w1553 w1580 w1607 w1634 w1657 w1664 w1686 w1694 w1721 w1748 w1775 w1802 w1829 w1856 w1883 w1910 w1937 w1964 w1991 w2018 w2045 w2072 w2099 w2126 w2153 w2180 w2207 w2234 w2261 w2288 w2315 w2342 w2369 w2391 w2399 w2426 w2453 w2480 w2507 w2534 w2561 w2588 w2615 w2642 w2669 w2696 w2723 w2750 w2777 w2804 w2831 w2858 w2885 w2912 w2939 w2966 w2993 w3020 w3047 w3074 w3101 w3128 w3155 w3182 w3209 w3232 w3239 w3266 w3289 w3296 w3323 w3346 w3353 w3380 w3403 w3410] -> w14
      tunnel: [w23 w28 w55 w82 w109 w136 w163 w190 w217 w244 w271 w298 w325 w352 w379 w402 w409 w436 w463 w490 w517 w544 w571 w598 w625 w652 w679 w706 w733 w760 w787 w814 w841 w868 w895 w922 w949 w976 w999 w1006 w1033 w1060 w1085 w1090 w1117 w1144 w1171 w1198 w1225 w1252 w1279 w1306 w1333 w1360 w1387 w1414 w1441 w1464 w1471 w1498 w1525 w1552 w1579 w1606 w1633 w1656 w1663 w1688 w1693 w1720 w1747 w1774 w1801 w1828 w1855 w1882 w1909 w1936 w1963 w1990 w2017 w2044 w2071 w2098 w2125 w2152 w2179 w2206 w2233 w2260 w2287 w2314 w2341 w2368 w2393 w2398 w2425 w2452 w2479 w2506 w2533 w2560 w2587 w2614 w2641 w2668 w2695 w2722 w2749 w2776 w2803 w2830 w2857 w2884 w2911 w2938 w2965 w2992 w3019 w3046 w3073 w3100 w3127 w3154 w3181 w3208 w3231 w3238 w3265 w3288 w3295 w3322 w3345 w3352 w3379 w3402 w3409] -> w17
      tunnel: w12 -> [_ w27 w54 w81 w108 w135 w162 w189 w216 w243 w270 w297 w324 w351 w378 _ w408 w435 w462 w489 w516 w543 w570 w597 w624 w651 w678 w705 w732 w759 w786 w813 w840 w867 w894 w921 w948 w975 _ w1005 w1032 w1059 _ w1089 w1116 w1143 w1170 w1197 w1224 w1251 w1278 w1305 w1332 w1359 w1386 w1413 w1440 _ w1470 w1497 w1524 w1551 w1578 w1605 w1632 _ w1662 _ w1692 w1719 w1746 w1773 w1800 w1827 w1854 w1881 w1908 w1935 w1962 w1989 w2016 w2043 w2070 w2097 w2124 w2151 w2178 w2205 w2232 w2259 w2286 w2313 w2340 w2367 _ w2397 w2424 w2451 w2478 w2505 w2532 w2559 w2586 w2613 w2640 w2667 w2694 w2721 w2748 w2775 w2802 w2829 w2856 w2883 w2910 w2937 w2964 w2991 w3018 w3045 w3072 w3099 w3126 w3153 w3180 w3207 _ w3237 w3264 _ w3294 w3321 _ w3351 w3378 _ w3408]
      tunnel: w11 -> [w21 w26 w53 w80 w107 w134 w161 w188 w215 w242 w269 w296 w323 w350 w377 w403 w407 w434 w461 w488 w515 w542 w569 w596 w623 w650 w677 w704 w731 w758 w785 w812 w839 w866 w893 w920 w947 w974 w1000 w1004 w1031 w1058 w1083 w1088 w1115 w1142 w1169 w1196 w1223 w1250 w1277 w1304 w1331 w1358 w1385 w1412 w1439 w1465 w1469 w1496 w1523 w1550 w1577 w1604 w1631 w1657 w1661 w1686 w1691 w1718 w1745 w1772 w1799 w1826 w1853 w1880 w1907 w1934 w1961 w1988 w2015 w2042 w2069 w2096 w2123 w2150 w2177 w2204 w2231 w2258 w2285 w2312 w2339 w2366 w2391 w2396 w2423 w2450 w2477 w2504 w2531 w2558 w2585 w2612 w2639 w2666 w2693 w2720 w2747 w2774 w2801 w2828 w2855 w2882 w2909 w2936 w2963 w2990 w3017 w3044 w3071 w3098 w3125 w3152 w3179 w3206 w3232 w3236 w3263 w3289 w3293 w3320 w3346 w3350 w3377 w3403 w3407]
      tunnel: [_ w25 w52 w79 w106 w133 w160 w187 w214 w241 w268 w295 w322 w349 w376 _ w406 w433 w460 w487 w514 w541 w567 w595 w622 w649 w676 w703 w730 w757 w784 w811 w838 w865 w892 w919 w946 w973 _ w1003 w1030 w1057 _ w1087 w1114 w1141 w1168 w1195 w1222 w1249 w1276 w1303 w1330 w1357 w1384 w1411 w1438 _ w1468 w1495 w1522 w1549 w1576 w1603 w1630 _ w1660 _ w1690 w1717 w1744 w1771 w1798 w1825 w1852 w1879 w1905 w1933 w1960 w1987 w2014 w2041 w2068 w2095 w2122 w2149 w2176 w2203 w2230 w2257 w2284 w2311 w2338 w2365 _ w2395 w2422 w2449 w2476 w2503 w2530 w2557 w2584 w2611 w2638 w2665 w2692 w2719 w2746 w2773 w2800 w2827 w2854 w2881 w2908 w2935 w2962 w2989 w3016 w3043 w3070 w3097 w3124 w3151 w3178 w3205 _ w3235 w3262 _ w3292 w3319 _ w3349 w3376 _ w3406] -> w10
      frame "---- GUI ----", Default {
      }
      frame "GUI:Initialization Status" {
        w24 = TRUE
        n4 = case shown="True" w27 {
          tunnel: w33 -> [w41 w50]
          tunnel: w32 -> [w40 w45]
          tunnel: w31 -> [w39 w49]
          tunnel: [w38 w43] -> w30
          tunnel: [w34 w42] -> w29
          tunnel: [w36 w44] -> w28
          tunnel: w24 -> [w35 w48]
          tunnel: w26 -> [_ w42]
          frame False {
            n5 = Get Variant Attribute(Variant=w41, name=w40, default value (empty Variant)=w35, error in=w39) -> (duplicate Variant=w36:variant, value=w37:bool, error out=w38:errorcluster)  [unwired: 1 out]
            n6 = To Variant(anything=w37) -> (Variant=w34:variant)
          }
          frame True {
            n7 = Variant To Data(error in=w49, type=w48, Variant=w42) -> (data=w47:bool, error out=w46:errorcluster)
            n8 = Set Variant Attribute(Variant=w50, name=w45, value=w47, error in=w46) -> (Variant out=w44:variant, error out=w43:errorcluster)  [unwired: 1 out]
          }
        }
        n9 = To Variant(anything=w24) -> (Variant=w25:variant)
      }
      frame "GUI:State Indicators Refnum" {
        n10 = case shown="True" w54 {
          tunnel: w60 -> [w68 w77]
          tunnel: w59 -> [w67 w72]
          tunnel: w58 -> [w66 w76]
          tunnel: [w65 w70] -> w57
          tunnel: [w61 w69] -> w56
          tunnel: [w63 w71] -> w55
          tunnel: "State Indicators" -> [w62 w75]
          tunnel: w53 -> [_ w69]
          frame False {
            n11 = Get Variant Attribute(Variant=w68, name=w67, default value (empty Variant)=w62, error in=w66) -> (duplicate Variant=w63:variant, value=w64:refnum<vi>, error out=w65:errorcluster)  [unwired: 1 out]
            n12 = To Variant(anything=w64) -> (Variant=w61:variant)
          }
          frame True {
            n13 = Variant To Data(error in=w76, type=w75, Variant=w69) -> (data=w74:refnum<vi>, error out=w73:errorcluster)
            n14 = Set Variant Attribute(Variant=w77, name=w72, value=w74, error in=w73) -> (Variant out=w71:variant, error out=w70:errorcluster)  [unwired: 1 out]
          }
        }
        n15 = To Variant(anything="State Indicators") -> (Variant=w52:variant)
      }
      frame "GUI:Current Action Loop State" {
        w78 = AlliGator_Q_Event."GUI:Idle" ("AlliGator Q Event")
        n16 = case shown="True" w81 {
          tunnel: w87 -> [w95 w104]
          tunnel: w86 -> [w94 w99]
          tunnel: w85 -> [w93 w103]
          tunnel: [w92 w97] -> w84
          tunnel: [w88 w96] -> w83
          tunnel: [w90 w98] -> w82
          tunnel: w78 -> [w89 w102]
          tunnel: w80 -> [_ w96]
          frame False {
            n17 = Get Variant Attribute(Variant=w95, name=w94, default value (empty Variant)=w89, error in=w93) -> (duplicate Variant=w90:variant, value=w91:T2, error out=w92:errorcluster)  [unwired: 1 out]
            n18 = To Variant(anything=w91) -> (Variant=w88:variant)
          }
          frame True {
            n19 = Variant To Data(error in=w103, type=w102, Variant=w96) -> (data=w101:T2, error out=w100:errorcluster)
            n20 = Set Variant Attribute(Variant=w104, name=w99, value=w101, error in=w100) -> (Variant out=w98:variant, error out=w97:errorcluster)  [unwired: 1 out]
          }
        }
        n21 = To Variant(anything=w78) -> (Variant=w79:variant)
      }
      frame "GUI:Script in progress" {
        w105 = FALSE
        n22 = case shown="True" w108 {
          tunnel: w114 -> [w122 w131]
          tunnel: w113 -> [w121 w126]
          tunnel: w112 -> [w120 w130]
          tunnel: [w119 w124] -> w111
          tunnel: [w115 w123] -> w110
          tunnel: [w117 w125] -> w109
          tunnel: w105 -> [w116 w129]
          tunnel: w107 -> [_ w123]
          frame False {
            n23 = Get Variant Attribute(Variant=w122, name=w121, default value (empty Variant)=w116, error in=w120) -> (duplicate Variant=w117:variant, value=w118:bool, error out=w119:errorcluster)  [unwired: 1 out]
            n24 = To Variant(anything=w118) -> (Variant=w115:variant)
          }
          frame True {
            n25 = Variant To Data(error in=w130, type=w129, Variant=w123) -> (data=w128:bool, error out=w127:errorcluster)
            n26 = Set Variant Attribute(Variant=w131, name=w126, value=w128, error in=w127) -> (Variant out=w125:variant, error out=w124:errorcluster)  [unwired: 1 out]
          }
        }
        n27 = To Variant(anything=w105) -> (Variant=w106:variant)
      }
      frame "GUI:Playback" {
        w132 = FALSE
        n28 = case shown="True" w135 {
          tunnel: w141 -> [w149 w158]
          tunnel: w140 -> [w148 w153]
          tunnel: w139 -> [w147 w157]
          tunnel: [w146 w151] -> w138
          tunnel: [w142 w150] -> w137
          tunnel: [w144 w152] -> w136
          tunnel: w132 -> [w143 w156]
          tunnel: w134 -> [_ w150]
          frame False {
            n29 = Get Variant Attribute(Variant=w149, name=w148, default value (empty Variant)=w143, error in=w147) -> (duplicate Variant=w144:variant, value=w145:bool, error out=w146:errorcluster)  [unwired: 1 out]
            n30 = To Variant(anything=w145) -> (Variant=w142:variant)
          }
          frame True {
            n31 = Variant To Data(error in=w157, type=w156, Variant=w150) -> (data=w155:bool, error out=w154:errorcluster)
            n32 = Set Variant Attribute(Variant=w158, name=w153, value=w155, error in=w154) -> (Variant out=w152:variant, error out=w151:errorcluster)  [unwired: 1 out]
          }
        }
        n33 = To Variant(anything=w132) -> (Variant=w133:variant)
      }
      frame "GUI:Loop Playback" {
        w159 = FALSE
        n34 = case shown="True" w162 {
          tunnel: w168 -> [w176 w185]
          tunnel: w167 -> [w175 w180]
          tunnel: w166 -> [w174 w184]
          tunnel: [w173 w178] -> w165
          tunnel: [w169 w177] -> w164
          tunnel: [w171 w179] -> w163
          tunnel: w159 -> [w170 w183]
          tunnel: w161 -> [_ w177]
          frame False {
            n35 = Get Variant Attribute(Variant=w176, name=w175, default value (empty Variant)=w170, error in=w174) -> (duplicate Variant=w171:variant, value=w172:bool, error out=w173:errorcluster)  [unwired: 1 out]
            n36 = To Variant(anything=w172) -> (Variant=w169:variant)
          }
          frame True {
            n37 = Variant To Data(error in=w184, type=w183, Variant=w177) -> (data=w182:bool, error out=w181:errorcluster)
            n38 = Set Variant Attribute(Variant=w185, name=w180, value=w182, error in=w181) -> (Variant out=w179:variant, error out=w178:errorcluster)  [unwired: 1 out]
          }
        }
        n39 = To Variant(anything=w159) -> (Variant=w160:variant)
      }
      frame "GUI:Search ROI Used" {
        w186 = FALSE
        n40 = case shown="True" w189 {
          tunnel: w195 -> [w203 w212]
          tunnel: w194 -> [w202 w207]
          tunnel: w193 -> [w201 w211]
          tunnel: [w200 w205] -> w192
          tunnel: [w196 w204] -> w191
          tunnel: [w198 w206] -> w190
          tunnel: w186 -> [w197 w210]
          tunnel: w188 -> [_ w204]
          frame False {
            n41 = Get Variant Attribute(Variant=w203, name=w202, default value (empty Variant)=w197, error in=w201) -> (duplicate Variant=w198:variant, value=w199:bool, error out=w200:errorcluster)  [unwired: 1 out]
            n42 = To Variant(anything=w199) -> (Variant=w196:variant)
          }
          frame True {
            n43 = Variant To Data(error in=w211, type=w210, Variant=w204) -> (data=w209:bool, error out=w208:errorcluster)
            n44 = Set Variant Attribute(Variant=w212, name=w207, value=w209, error in=w208) -> (Variant out=w206:variant, error out=w205:errorcluster)  [unwired: 1 out]
          }
        }
        n45 = To Variant(anything=w186) -> (Variant=w187:variant)
      }
      frame "GUI:Search ROI" {
        w213 = T3 {"Global Rectangle"=[], "Contours"=[]} ("ROI Descriptor")
        n46 = case shown="True" w216 {
          tunnel: w222 -> [w230 w239]
          tunnel: w221 -> [w229 w234]
          tunnel: w220 -> [w228 w238]
          tunnel: [w227 w232] -> w219
          tunnel: [w223 w231] -> w218
          tunnel: [w225 w233] -> w217
          tunnel: w213 -> [w224 w237]
          tunnel: w215 -> [_ w231]
          frame False {
            n47 = Get Variant Attribute(Variant=w230, name=w229, default value (empty Variant)=w224, error in=w228) -> (duplicate Variant=w225:variant, value=w226:T3, error out=w227:errorcluster)  [unwired: 1 out]
            n48 = To Variant(anything=w226) -> (Variant=w223:variant)
          }
          frame True {
            n49 = Variant To Data(error in=w238, type=w237, Variant=w231) -> (data=w236:T3, error out=w235:errorcluster)
            n50 = Set Variant Attribute(Variant=w239, name=w234, value=w236, error in=w235) -> (Variant out=w233:variant, error out=w232:errorcluster)  [unwired: 1 out]
          }
        }
        n51 = To Variant(anything=w213) -> (Variant=w214:variant)
      }
      frame "Decay Graph Max Legend Size" {
        w240 = 0
        n52 = case shown="True" w243 {
          tunnel: w249 -> [w257 w266]
          tunnel: w248 -> [w256 w261]
          tunnel: w247 -> [w255 w265]
          tunnel: [w254 w259] -> w246
          tunnel: [w250 w258] -> w245
          tunnel: [w252 w260] -> w244
          tunnel: w240 -> [w251 w264]
          tunnel: w242 -> [_ w258]
          frame False {
            n53 = Get Variant Attribute(Variant=w257, name=w256, default value (empty Variant)=w251, error in=w255) -> (duplicate Variant=w252:variant, value=w253:i32, error out=w254:errorcluster)  [unwired: 1 out]
            n54 = To Variant(anything=w253) -> (Variant=w250:variant)
          }
          frame True {
            n55 = Variant To Data(error in=w265, type=w264, Variant=w258) -> (data=w263:i32, error out=w262:errorcluster)
            n56 = Set Variant Attribute(Variant=w266, name=w261, value=w263, error in=w262) -> (Variant out=w260:variant, error out=w259:errorcluster)  [unwired: 1 out]
          }
        }
        n57 = To Variant(anything=w240) -> (Variant=w241:variant)
      }
      frame "Intensity Graph Max Legend Size" {
        w267 = 0
        n58 = case shown="True" w270 {
          tunnel: w276 -> [w284 w293]
          tunnel: w275 -> [w283 w288]
          tunnel: w274 -> [w282 w292]
          tunnel: [w281 w286] -> w273
          tunnel: [w277 w285] -> w272
          tunnel: [w279 w287] -> w271
          tunnel: w267 -> [w278 w291]
          tunnel: w269 -> [_ w285]
          frame False {
            n59 = Get Variant Attribute(Variant=w284, name=w283, default value (empty Variant)=w278, error in=w282) -> (duplicate Variant=w279:variant, value=w280:i32, error out=w281:errorcluster)  [unwired: 1 out]
            n60 = To Variant(anything=w280) -> (Variant=w277:variant)
          }
          frame True {
            n61 = Variant To Data(error in=w292, type=w291, Variant=w285) -> (data=w290:i32, error out=w289:errorcluster)
            n62 = Set Variant Attribute(Variant=w293, name=w288, value=w290, error in=w289) -> (Variant out=w287:variant, error out=w286:errorcluster)  [unwired: 1 out]
          }
        }
        n63 = To Variant(anything=w267) -> (Variant=w268:variant)
      }
      frame "Decay Statistics Graph Max Legend Size" {
        w294 = 0
        n64 = case shown="True" w297 {
          tunnel: w303 -> [w311 w320]
          tunnel: w302 -> [w310 w315]
          tunnel: w301 -> [w309 w319]
          tunnel: [w308 w313] -> w300
          tunnel: [w304 w312] -> w299
          tunnel: [w306 w314] -> w298
          tunnel: w294 -> [w305 w318]
          tunnel: w296 -> [_ w312]
          frame False {
            n65 = Get Variant Attribute(Variant=w311, name=w310, default value (empty Variant)=w305, error in=w309) -> (duplicate Variant=w306:variant, value=w307:i32, error out=w308:errorcluster)  [unwired: 1 out]
            n66 = To Variant(anything=w307) -> (Variant=w304:variant)
          }
          frame True {
            n67 = Variant To Data(error in=w319, type=w318, Variant=w312) -> (data=w317:i32, error out=w316:errorcluster)
            n68 = Set Variant Attribute(Variant=w320, name=w315, value=w317, error in=w316) -> (Variant out=w314:variant, error out=w313:errorcluster)  [unwired: 1 out]
          }
        }
        n69 = To Variant(anything=w294) -> (Variant=w295:variant)
      }
      frame "Phasor Graph Max Legend Size" {
        w321 = 0
        n70 = case shown="True" w324 {
          tunnel: w330 -> [w338 w347]
          tunnel: w329 -> [w337 w342]
          tunnel: w328 -> [w336 w346]
          tunnel: [w335 w340] -> w327
          tunnel: [w331 w339] -> w326
          tunnel: [w333 w341] -> w325
          tunnel: w321 -> [w332 w345]
          tunnel: w323 -> [_ w339]
          frame False {
            n71 = Get Variant Attribute(Variant=w338, name=w337, default value (empty Variant)=w332, error in=w336) -> (duplicate Variant=w333:variant, value=w334:i32, error out=w335:errorcluster)  [unwired: 1 out]
            n72 = To Variant(anything=w334) -> (Variant=w331:variant)
          }
          frame True {
            n73 = Variant To Data(error in=w346, type=w345, Variant=w339) -> (data=w344:i32, error out=w343:errorcluster)
            n74 = Set Variant Attribute(Variant=w347, name=w342, value=w344, error in=w343) -> (Variant out=w341:variant, error out=w340:errorcluster)  [unwired: 1 out]
          }
        }
        n75 = To Variant(anything=w321) -> (Variant=w322:variant)
      }
      frame "Phasor Ratio Graph Max Legend Size" {
        w348 = 0
        n76 = case shown="True" w351 {
          tunnel: w357 -> [w365 w374]
          tunnel: w356 -> [w364 w369]
          tunnel: w355 -> [w363 w373]
          tunnel: [w362 w367] -> w354
          tunnel: [w358 w366] -> w353
          tunnel: [w360 w368] -> w352
          tunnel: w348 -> [w359 w372]
          tunnel: w350 -> [_ w366]
          frame False {
            n77 = Get Variant Attribute(Variant=w365, name=w364, default value (empty Variant)=w359, error in=w363) -> (duplicate Variant=w360:variant, value=w361:i32, error out=w362:errorcluster)  [unwired: 1 out]
            n78 = To Variant(anything=w361) -> (Variant=w358:variant)
          }
          frame True {
            n79 = Variant To Data(error in=w373, type=w372, Variant=w366) -> (data=w371:i32, error out=w370:errorcluster)
            n80 = Set Variant Attribute(Variant=w374, name=w369, value=w371, error in=w370) -> (Variant out=w368:variant, error out=w367:errorcluster)  [unwired: 1 out]
          }
        }
        n81 = To Variant(anything=w348) -> (Variant=w349:variant)
      }
      frame "Lifetime Graph Max Legend Size" {
        w375 = 0
        n82 = case shown="True" w378 {
          tunnel: w384 -> [w392 w401]
          tunnel: w383 -> [w391 w396]
          tunnel: w382 -> [w390 w400]
          tunnel: [w389 w394] -> w381
          tunnel: [w385 w393] -> w380
          tunnel: [w387 w395] -> w379
          tunnel: w375 -> [w386 w399]
          tunnel: w377 -> [_ w393]
          frame False {
            n83 = Get Variant Attribute(Variant=w392, name=w391, default value (empty Variant)=w386, error in=w390) -> (duplicate Variant=w387:variant, value=w388:i32, error out=w389:errorcluster)  [unwired: 1 out]
            n84 = To Variant(anything=w388) -> (Variant=w385:variant)
          }
          frame True {
            n85 = Variant To Data(error in=w400, type=w399, Variant=w393) -> (data=w398:i32, error out=w397:errorcluster)
            n86 = Set Variant Attribute(Variant=w401, name=w396, value=w398, error in=w397) -> (Variant out=w395:variant, error out=w394:errorcluster)  [unwired: 1 out]
          }
        }
        n87 = To Variant(anything=w375) -> (Variant=w376:variant)
      }
      frame "---- Files ----" {
      }
      frame "Files:Export Dataset Frames as Individual Files" {
        w405 = FALSE
        n88 = case shown="True" w408 {
          tunnel: w414 -> [w422 w431]
          tunnel: w413 -> [w421 w426]
          tunnel: w412 -> [w420 w430]
          tunnel: [w419 w424] -> w411
          tunnel: [w415 w423] -> w410
          tunnel: [w417 w425] -> w409
          tunnel: w405 -> [w416 w429]
          tunnel: w407 -> [_ w423]
          frame False {
            n89 = Get Variant Attribute(Variant=w422, name=w421, default value (empty Variant)=w416, error in=w420) -> (duplicate Variant=w417:variant, value=w418:bool, error out=w419:errorcluster)  [unwired: 1 out]
            n90 = To Variant(anything=w418) -> (Variant=w415:variant)
          }
          frame True {
            n91 = Variant To Data(error in=w430, type=w429, Variant=w423) -> (data=w428:bool, error out=w427:errorcluster)
            n92 = Set Variant Attribute(Variant=w431, name=w426, value=w428, error in=w427) -> (Variant out=w425:variant, error out=w424:errorcluster)  [unwired: 1 out]
          }
        }
        n93 = To Variant(anything=w405) -> (Variant=w406:variant)
      }
      frame "Files:Show Batch Export Help Balloons" {
        w432 = FALSE
        n94 = case shown="True" w435 {
          tunnel: w441 -> [w449 w458]
          tunnel: w440 -> [w448 w453]
          tunnel: w439 -> [w447 w457]
          tunnel: [w446 w451] -> w438
          tunnel: [w442 w450] -> w437
          tunnel: [w444 w452] -> w436
          tunnel: w432 -> [w443 w456]
          tunnel: w434 -> [_ w450]
          frame False {
            n95 = Get Variant Attribute(Variant=w449, name=w448, default value (empty Variant)=w443, error in=w447) -> (duplicate Variant=w444:variant, value=w445:bool, error out=w446:errorcluster)  [unwired: 1 out]
            n96 = To Variant(anything=w445) -> (Variant=w442:variant)
          }
          frame True {
            n97 = Variant To Data(error in=w457, type=w456, Variant=w450) -> (data=w455:bool, error out=w454:errorcluster)
            n98 = Set Variant Attribute(Variant=w458, name=w453, value=w455, error in=w454) -> (Variant out=w452:variant, error out=w451:errorcluster)  [unwired: 1 out]
          }
        }
        n99 = To Variant(anything=w432) -> (Variant=w433:variant)
      }
      frame "Files:Frames in Dataset" {
        w459 = 1
        n100 = case shown="True" w462 {
          tunnel: w468 -> [w476 w485]
          tunnel: w467 -> [w475 w480]
          tunnel: w466 -> [w474 w484]
          tunnel: [w473 w478] -> w465
          tunnel: [w469 w477] -> w464
          tunnel: [w471 w479] -> w463
          tunnel: w459 -> [w470 w483]
          tunnel: w461 -> [_ w477]
          frame False {
            n101 = Get Variant Attribute(Variant=w476, name=w475, default value (empty Variant)=w470, error in=w474) -> (duplicate Variant=w471:variant, value=w472:i32, error out=w473:errorcluster)  [unwired: 1 out]
            n102 = To Variant(anything=w472) -> (Variant=w469:variant)
          }
          frame True {
            n103 = Variant To Data(error in=w484, type=w483, Variant=w477) -> (data=w482:i32, error out=w481:errorcluster)
            n104 = Set Variant Attribute(Variant=w485, name=w480, value=w482, error in=w481) -> (Variant out=w479:variant, error out=w478:errorcluster)  [unwired: 1 out]
          }
        }
        n105 = To Variant(anything=w459) -> (Variant=w460:variant)
      }
      frame "Files:ptu File Frame Start Indices" {
        w486 = i32[] []
        n106 = case shown="True" w489 {
          tunnel: w495 -> [w503 w512]
          tunnel: w494 -> [w502 w507]
          tunnel: w493 -> [w501 w511]
          tunnel: [w500 w505] -> w492
          tunnel: [w496 w504] -> w491
          tunnel: [w498 w506] -> w490
          tunnel: w486 -> [w497 w510]
          tunnel: w488 -> [_ w504]
          frame False {
            n107 = Get Variant Attribute(Variant=w503, name=w502, default value (empty Variant)=w497, error in=w501) -> (duplicate Variant=w498:variant, value=w499:i32[], error out=w500:errorcluster)  [unwired: 1 out]
            n108 = To Variant(anything=w499) -> (Variant=w496:variant)
          }
          frame True {
            n109 = Variant To Data(error in=w511, type=w510, Variant=w504) -> (data=w509:i32[], error out=w508:errorcluster)
            n110 = Set Variant Attribute(Variant=w512, name=w507, value=w509, error in=w508) -> (Variant out=w506:variant, error out=w505:errorcluster)  [unwired: 1 out]
          }
        }
        n111 = To Variant(anything=w486) -> (Variant=w487:variant)
      }
      frame "Files:Current Frame in Dataset" {
        w513 = 1
        n112 = case shown="True" w516 {
          tunnel: w522 -> [w530 w539]
          tunnel: w521 -> [w529 w534]
          tunnel: w520 -> [w528 w538]
          tunnel: [w527 w532] -> w519
          tunnel: [w523 w531] -> w518
          tunnel: [w525 w533] -> w517
          tunnel: w513 -> [w524 w537]
          tunnel: w515 -> [_ w531]
          frame False {
            n113 = Get Variant Attribute(Variant=w530, name=w529, default value (empty Variant)=w524, error in=w528) -> (duplicate Variant=w525:variant, value=w526:i32, error out=w527:errorcluster)  [unwired: 1 out]
            n114 = To Variant(anything=w526) -> (Variant=w523:variant)
          }
          frame True {
            n115 = Variant To Data(error in=w538, type=w537, Variant=w531) -> (data=w536:i32, error out=w535:errorcluster)
            n116 = Set Variant Attribute(Variant=w539, name=w534, value=w536, error in=w535) -> (Variant out=w533:variant, error out=w532:errorcluster)  [unwired: 1 out]
          }
        }
        n117 = To Variant(anything=w513) -> (Variant=w514:variant)
      }
      frame "Files:Current Frame Timestamp" {
        w540 = nan
        n118 = case shown="True" w543 {
          tunnel: w549 -> [w557 w566]
          tunnel: w548 -> [w556 w561]
          tunnel: w547 -> [w555 w565]
          tunnel: [w554 w559] -> w546
          tunnel: [w550 w558] -> w545
          tunnel: [w552 w560] -> w544
          tunnel: w540 -> [w551 w564]
          tunnel: w542 -> [_ w558]
          frame False {
            n119 = Get Variant Attribute(Variant=w557, name=w556, default value (empty Variant)=w551, error in=w555) -> (duplicate Variant=w552:variant, value=w553:dbl, error out=w554:errorcluster)  [unwired: 1 out]
            n120 = To Variant(anything=w553) -> (Variant=w550:variant)
          }
          frame True {
            n121 = Variant To Data(error in=w565, type=w564, Variant=w558) -> (data=w563:dbl, error out=w562:errorcluster)
            n122 = Set Variant Attribute(Variant=w566, name=w561, value=w563, error in=w562) -> (Variant out=w560:variant, error out=w559:errorcluster)  [unwired: 1 out]
          }
        }
        n123 = To Variant(anything=w540) -> (Variant=w541:variant)
      }
      frame "Files:Dataset Loaded" {
        w568 = FALSE
        n124 = case shown="True" w570 {
          tunnel: w576 -> [w584 w593]
          tunnel: w575 -> [w583 w588]
          tunnel: w574 -> [w582 w592]
          tunnel: [w581 w586] -> w573
          tunnel: [w577 w585] -> w572
          tunnel: [w579 w587] -> w571
          tunnel: w568 -> [w578 w591]
          tunnel: w569 -> [_ w585]
          frame False {
            n125 = Get Variant Attribute(Variant=w584, name=w583, default value (empty Variant)=w578, error in=w582) -> (duplicate Variant=w579:variant, value=w580:bool, error out=w581:errorcluster)  [unwired: 1 out]
            n126 = To Variant(anything=w580) -> (Variant=w577:variant)
          }
          frame True {
            n127 = Variant To Data(error in=w592, type=w591, Variant=w585) -> (data=w590:bool, error out=w589:errorcluster)
            n128 = Set Variant Attribute(Variant=w593, name=w588, value=w590, error in=w589) -> (Variant out=w587:variant, error out=w586:errorcluster)  [unwired: 1 out]
          }
        }
        n129 = To Variant(anything=w568) -> (Variant=w567:variant)
      }
      frame "Files:Dataset Metadata" {
        w594 = ""
        n130 = case shown="True" w597 {
          tunnel: w603 -> [w611 w620]
          tunnel: w602 -> [w610 w615]
          tunnel: w601 -> [w609 w619]
          tunnel: [w608 w613] -> w600
          tunnel: [w604 w612] -> w599
          tunnel: [w606 w614] -> w598
          tunnel: w594 -> [w605 w618]
          tunnel: w596 -> [_ w612]
          frame False {
            n131 = Get Variant Attribute(Variant=w611, name=w610, default value (empty Variant)=w605, error in=w609) -> (duplicate Variant=w606:variant, value=w607:string, error out=w608:errorcluster)  [unwired: 1 out]
            n132 = To Variant(anything=w607) -> (Variant=w604:variant)
          }
          frame True {
            n133 = Variant To Data(error in=w619, type=w618, Variant=w612) -> (data=w617:string, error out=w616:errorcluster)
            n134 = Set Variant Attribute(Variant=w620, name=w615, value=w617, error in=w616) -> (Variant out=w614:variant, error out=w613:errorcluster)  [unwired: 1 out]
          }
        }
        n135 = To Variant(anything=w594) -> (Variant=w595:variant)
      }
      frame "Files:Dataset Channel" {
        w621 = AlliGator_Dataset_Channel."G2" ("Dataset Channel")
        n136 = case shown="True" w624 {
          tunnel: w630 -> [w638 w647]
          tunnel: w629 -> [w637 w642]
          tunnel: w628 -> [w636 w646]
          tunnel: [w635 w640] -> w627
          tunnel: [w631 w639] -> w626
          tunnel: [w633 w641] -> w625
          tunnel: w621 -> [w632 w645]
          tunnel: w623 -> [_ w639]
          frame False {
            n137 = Get Variant Attribute(Variant=w638, name=w637, default value (empty Variant)=w632, error in=w636) -> (duplicate Variant=w633:variant, value=w634:T4, error out=w635:errorcluster)  [unwired: 1 out]
            n138 = To Variant(anything=w634) -> (Variant=w631:variant)
          }
          frame True {
            n139 = Variant To Data(error in=w646, type=w645, Variant=w639) -> (data=w644:T4, error out=w643:errorcluster)
            n140 = Set Variant Attribute(Variant=w647, name=w642, value=w644, error in=w643) -> (Variant out=w641:variant, error out=w640:errorcluster)  [unwired: 1 out]
          }
        }
        n141 = To Variant(anything=w621) -> (Variant=w622:variant)
      }
      frame "Files:Dataset Data Description" {
        w648 = ""
        n142 = case shown="True" w651 {
          tunnel: w657 -> [w665 w674]
          tunnel: w656 -> [w664 w669]
          tunnel: w655 -> [w663 w673]
          tunnel: [w662 w667] -> w654
          tunnel: [w658 w666] -> w653
          tunnel: [w660 w668] -> w652
          tunnel: w648 -> [w659 w672]
          tunnel: w650 -> [_ w666]
          frame False {
            n143 = Get Variant Attribute(Variant=w665, name=w664, default value (empty Variant)=w659, error in=w663) -> (duplicate Variant=w660:variant, value=w661:string, error out=w662:errorcluster)  [unwired: 1 out]
            n144 = To Variant(anything=w661) -> (Variant=w658:variant)
          }
          frame True {
            n145 = Variant To Data(error in=w673, type=w672, Variant=w666) -> (data=w671:string, error out=w670:errorcluster)
            n146 = Set Variant Attribute(Variant=w674, name=w669, value=w671, error in=w670) -> (Variant out=w668:variant, error out=w667:errorcluster)  [unwired: 1 out]
          }
        }
        n147 = To Variant(anything=w648) -> (Variant=w649:variant)
      }
      frame "Files:Background Dataset Metadata" {
        w675 = ""
        n148 = case shown="True" w678 {
          tunnel: w684 -> [w692 w701]
          tunnel: w683 -> [w691 w696]
          tunnel: w682 -> [w690 w700]
          tunnel: [w689 w694] -> w681
          tunnel: [w685 w693] -> w680
          tunnel: [w687 w695] -> w679
          tunnel: w675 -> [w686 w699]
          tunnel: w677 -> [_ w693]
          frame False {
            n149 = Get Variant Attribute(Variant=w692, name=w691, default value (empty Variant)=w686, error in=w690) -> (duplicate Variant=w687:variant, value=w688:string, error out=w689:errorcluster)  [unwired: 1 out]
            n150 = To Variant(anything=w688) -> (Variant=w685:variant)
          }
          frame True {
            n151 = Variant To Data(error in=w700, type=w699, Variant=w693) -> (data=w698:string, error out=w697:errorcluster)
            n152 = Set Variant Attribute(Variant=w701, name=w696, value=w698, error in=w697) -> (Variant out=w695:variant, error out=w694:errorcluster)  [unwired: 1 out]
          }
        }
        n153 = To Variant(anything=w675) -> (Variant=w676:variant)
      }
      frame "Files:Background Dataset Channel" {
        w702 = AlliGator_Dataset_Channel."G2" ("Dataset Channel")
        n154 = case shown="True" w705 {
          tunnel: w711 -> [w719 w728]
          tunnel: w710 -> [w718 w723]
          tunnel: w709 -> [w717 w727]
          tunnel: [w716 w721] -> w708
          tunnel: [w712 w720] -> w707
          tunnel: [w714 w722] -> w706
          tunnel: w702 -> [w713 w726]
          tunnel: w704 -> [_ w720]
          frame False {
            n155 = Get Variant Attribute(Variant=w719, name=w718, default value (empty Variant)=w713, error in=w717) -> (duplicate Variant=w714:variant, value=w715:T4, error out=w716:errorcluster)  [unwired: 1 out]
            n156 = To Variant(anything=w715) -> (Variant=w712:variant)
          }
          frame True {
            n157 = Variant To Data(error in=w727, type=w726, Variant=w720) -> (data=w725:T4, error out=w724:errorcluster)
            n158 = Set Variant Attribute(Variant=w728, name=w723, value=w725, error in=w724) -> (Variant out=w722:variant, error out=w721:errorcluster)  [unwired: 1 out]
          }
        }
        n159 = To Variant(anything=w702) -> (Variant=w703:variant)
      }
      frame "Files:Background Dataset Data Description" {
        w729 = ""
        n160 = case shown="True" w732 {
          tunnel: w738 -> [w746 w755]
          tunnel: w737 -> [w745 w750]
          tunnel: w736 -> [w744 w754]
          tunnel: [w743 w748] -> w735
          tunnel: [w739 w747] -> w734
          tunnel: [w741 w749] -> w733
          tunnel: w729 -> [w740 w753]
          tunnel: w731 -> [_ w747]
          frame False {
            n161 = Get Variant Attribute(Variant=w746, name=w745, default value (empty Variant)=w740, error in=w744) -> (duplicate Variant=w741:variant, value=w742:string, error out=w743:errorcluster)  [unwired: 1 out]
            n162 = To Variant(anything=w742) -> (Variant=w739:variant)
          }
          frame True {
            n163 = Variant To Data(error in=w754, type=w753, Variant=w747) -> (data=w752:string, error out=w751:errorcluster)
            n164 = Set Variant Attribute(Variant=w755, name=w750, value=w752, error in=w751) -> (Variant out=w749:variant, error out=w748:errorcluster)  [unwired: 1 out]
          }
        }
        n165 = To Variant(anything=w729) -> (Variant=w730:variant)
      }
      frame "Files:Background File Subtraction" {
        w756 = FALSE
        n166 = case shown="True" w759 {
          tunnel: w765 -> [w773 w782]
          tunnel: w764 -> [w772 w777]
          tunnel: w763 -> [w771 w781]
          tunnel: [w770 w775] -> w762
          tunnel: [w766 w774] -> w761
          tunnel: [w768 w776] -> w760
          tunnel: w756 -> [w767 w780]
          tunnel: w758 -> [_ w774]
          frame False {
            n167 = Get Variant Attribute(Variant=w773, name=w772, default value (empty Variant)=w767, error in=w771) -> (duplicate Variant=w768:variant, value=w769:bool, error out=w770:errorcluster)  [unwired: 1 out]
            n168 = To Variant(anything=w769) -> (Variant=w766:variant)
          }
          frame True {
            n169 = Variant To Data(error in=w781, type=w780, Variant=w774) -> (data=w779:bool, error out=w778:errorcluster)
            n170 = Set Variant Attribute(Variant=w782, name=w777, value=w779, error in=w778) -> (Variant out=w776:variant, error out=w775:errorcluster)  [unwired: 1 out]
          }
        }
        n171 = To Variant(anything=w756) -> (Variant=w757:variant)
      }
      frame "Files:Background File Path" {
        w783 = path ""
        n172 = case shown="True" w786 {
          tunnel: w792 -> [w800 w809]
          tunnel: w791 -> [w799 w804]
          tunnel: w790 -> [w798 w808]
          tunnel: [w797 w802] -> w789
          tunnel: [w793 w801] -> w788
          tunnel: [w795 w803] -> w787
          tunnel: w783 -> [w794 w807]
          tunnel: w785 -> [_ w801]
          frame False {
            n173 = Get Variant Attribute(Variant=w800, name=w799, default value (empty Variant)=w794, error in=w798) -> (duplicate Variant=w795:variant, value=w796:path, error out=w797:errorcluster)  [unwired: 1 out]
            n174 = To Variant(anything=w796) -> (Variant=w793:variant)
          }
          frame True {
            n175 = Variant To Data(error in=w808, type=w807, Variant=w801) -> (data=w806:path, error out=w805:errorcluster)
            n176 = Set Variant Attribute(Variant=w809, name=w804, value=w806, error in=w805) -> (Variant out=w803:variant, error out=w802:errorcluster)  [unwired: 1 out]
          }
        }
        n177 = To Variant(anything=w783) -> (Variant=w784:variant)
      }
      frame "Files:Background File Pile-up Correction" {
        w810 = FALSE
        n178 = case shown="True" w813 {
          tunnel: w819 -> [w827 w836]
          tunnel: w818 -> [w826 w831]
          tunnel: w817 -> [w825 w835]
          tunnel: [w824 w829] -> w816
          tunnel: [w820 w828] -> w815
          tunnel: [w822 w830] -> w814
          tunnel: w810 -> [w821 w834]
          tunnel: w812 -> [_ w828]
          frame False {
            n179 = Get Variant Attribute(Variant=w827, name=w826, default value (empty Variant)=w821, error in=w825) -> (duplicate Variant=w822:variant, value=w823:bool, error out=w824:errorcluster)  [unwired: 1 out]
            n180 = To Variant(anything=w823) -> (Variant=w820:variant)
          }
          frame True {
            n181 = Variant To Data(error in=w835, type=w834, Variant=w828) -> (data=w833:bool, error out=w832:errorcluster)
            n182 = Set Variant Attribute(Variant=w836, name=w831, value=w833, error in=w832) -> (Variant out=w830:variant, error out=w829:errorcluster)  [unwired: 1 out]
          }
        }
        n183 = To Variant(anything=w810) -> (Variant=w811:variant)
      }
      frame "Files:Background File Pixel Well Capacity" {
        w837 = u32 0
        n184 = case shown="True" w840 {
          tunnel: w846 -> [w854 w863]
          tunnel: w845 -> [w853 w858]
          tunnel: w844 -> [w852 w862]
          tunnel: [w851 w856] -> w843
          tunnel: [w847 w855] -> w842
          tunnel: [w849 w857] -> w841
          tunnel: w837 -> [w848 w861]
          tunnel: w839 -> [_ w855]
          frame False {
            n185 = Get Variant Attribute(Variant=w854, name=w853, default value (empty Variant)=w848, error in=w852) -> (duplicate Variant=w849:variant, value=w850:u32, error out=w851:errorcluster)  [unwired: 1 out]
            n186 = To Variant(anything=w850) -> (Variant=w847:variant)
          }
          frame True {
            n187 = Variant To Data(error in=w862, type=w861, Variant=w855) -> (data=w860:u32, error out=w859:errorcluster)
            n188 = Set Variant Attribute(Variant=w863, name=w858, value=w860, error in=w859) -> (Variant out=w857:variant, error out=w856:errorcluster)  [unwired: 1 out]
          }
        }
        n189 = To Variant(anything=w837) -> (Variant=w838:variant)
      }
      frame "Files:Background File Scaling Factor" {
        w864 = 0.0
        n190 = case shown="True" w867 {
          tunnel: w873 -> [w881 w890]
          tunnel: w872 -> [w880 w885]
          tunnel: w871 -> [w879 w889]
          tunnel: [w878 w883] -> w870
          tunnel: [w874 w882] -> w869
          tunnel: [w876 w884] -> w868
          tunnel: w864 -> [w875 w888]
          tunnel: w866 -> [_ w882]
          frame False {
            n191 = Get Variant Attribute(Variant=w881, name=w880, default value (empty Variant)=w875, error in=w879) -> (duplicate Variant=w876:variant, value=w877:dbl, error out=w878:errorcluster)  [unwired: 1 out]
            n192 = To Variant(anything=w877) -> (Variant=w874:variant)
          }
          frame True {
            n193 = Variant To Data(error in=w889, type=w888, Variant=w882) -> (data=w887:dbl, error out=w886:errorcluster)
            n194 = Set Variant Attribute(Variant=w890, name=w885, value=w887, error in=w886) -> (Variant out=w884:variant, error out=w883:errorcluster)  [unwired: 1 out]
          }
        }
        n195 = To Variant(anything=w864) -> (Variant=w865:variant)
      }
      frame "Files:Current Dataset Load Settings" {
        w891 = T5 {"Pixel Well Capacity"=0, "Pile-up Correction"=FALSE, "Gate Step"=0, "Image Smoothing Options"={"Use Image Smoothing"=FALSE, "Kernel Type"=enum."Bilinear", "Bin"=1, "Algorithm"=enum."Rapid"}, "Gates to Skip"={"Start"=0, "End"=0}, "File Background Subtraction"=FALSE, "Background File Path"=path "", "Image Binning Options"={"Use Image Binning"=FALSE, "X Bin"=1, "Y Bin"=1}, "# Gates"=0, "Gates to Keep"={"First"=0, "Last"=0}, "Define Gates to"=FALSE, "Hot Pixel Removal"={"Remove Screamers"=FALSE, "Delta"=0.0, "Equalize Histogram"=FALSE, "Percentile"=0.0, "Hot Pixel Mask Image"=path "", "Use Hot Pixel Mask"=FALSE}, "Dataset Scaling Factor"=0.0, "Image Pre-processing Steps"=[]} ("Image Loading Options")
        n196 = case shown="True" w894 {
          tunnel: w900 -> [w908 w917]
          tunnel: w899 -> [w907 w912]
          tunnel: w898 -> [w906 w916]
          tunnel: [w905 w910] -> w897
          tunnel: [w901 w909] -> w896
          tunnel: [w903 w911] -> w895
          tunnel: w891 -> [w902 w915]
          tunnel: w893 -> [_ w909]
          frame False {
            n197 = Get Variant Attribute(Variant=w908, name=w907, default value (empty Variant)=w902, error in=w906) -> (duplicate Variant=w903:variant, value=w904:T5, error out=w905:errorcluster)  [unwired: 1 out]
            n198 = To Variant(anything=w904) -> (Variant=w901:variant)
          }
          frame True {
            n199 = Variant To Data(error in=w916, type=w915, Variant=w909) -> (data=w914:T5, error out=w913:errorcluster)
            n200 = Set Variant Attribute(Variant=w917, name=w912, value=w914, error in=w913) -> (Variant out=w911:variant, error out=w910:errorcluster)  [unwired: 1 out]
          }
        }
        n201 = To Variant(anything=w891) -> (Variant=w892:variant)
      }
      frame "Files:Dataset Path" {
        w918 = path ""
        n202 = case shown="True" w921 {
          tunnel: w927 -> [w935 w944]
          tunnel: w926 -> [w934 w939]
          tunnel: w925 -> [w933 w943]
          tunnel: [w932 w937] -> w924
          tunnel: [w928 w936] -> w923
          tunnel: [w930 w938] -> w922
          tunnel: w918 -> [w929 w942]
          tunnel: w920 -> [_ w936]
          frame False {
            n203 = Get Variant Attribute(Variant=w935, name=w934, default value (empty Variant)=w929, error in=w933) -> (duplicate Variant=w930:variant, value=w931:path, error out=w932:errorcluster)  [unwired: 1 out]
            n204 = To Variant(anything=w931) -> (Variant=w928:variant)
          }
          frame True {
            n205 = Variant To Data(error in=w943, type=w942, Variant=w936) -> (data=w941:path, error out=w940:errorcluster)
            n206 = Set Variant Attribute(Variant=w944, name=w939, value=w941, error in=w940) -> (Variant out=w938:variant, error out=w937:errorcluster)  [unwired: 1 out]
          }
        }
        n207 = To Variant(anything=w918) -> (Variant=w919:variant)
      }
      frame "Files:ICCD-specific Information" {
        w945 = T14 {"V MCP"=0.0, "X Hardware Binning"=0.0, "Y Hardware Binning"=0.0, "Gate Image Integration"=0.0, "Laser Power"=0.0} ("ICCD-specific Information")
        n208 = case shown="True" w948 {
          tunnel: w954 -> [w962 w971]
          tunnel: w953 -> [w961 w966]
          tunnel: w952 -> [w960 w970]
          tunnel: [w959 w964] -> w951
          tunnel: [w955 w963] -> w950
          tunnel: [w957 w965] -> w949
          tunnel: w945 -> [w956 w969]
          tunnel: w947 -> [_ w963]
          frame False {
            n209 = Get Variant Attribute(Variant=w962, name=w961, default value (empty Variant)=w956, error in=w960) -> (duplicate Variant=w957:variant, value=w958:T14, error out=w959:errorcluster)  [unwired: 1 out]
            n210 = To Variant(anything=w958) -> (Variant=w955:variant)
          }
          frame True {
            n211 = Variant To Data(error in=w970, type=w969, Variant=w963) -> (data=w968:T14, error out=w967:errorcluster)
            n212 = Set Variant Attribute(Variant=w971, name=w966, value=w968, error in=w967) -> (Variant out=w965:variant, error out=w964:errorcluster)  [unwired: 1 out]
          }
        }
        n213 = To Variant(anything=w945) -> (Variant=w946:variant)
      }
      frame "Files:Macrotime Gate Separation" {
        w972 = dbl[unit] nan  # s
        n214 = case shown="True" w975 {
          tunnel: w981 -> [w989 w998]
          tunnel: w980 -> [w988 w993]
          tunnel: w979 -> [w987 w997]
          tunnel: [w986 w991] -> w978
          tunnel: [w982 w990] -> w977
          tunnel: [w984 w992] -> w976
          tunnel: w972 -> [w983 w996]
          tunnel: w974 -> [_ w990]
          frame False {
            n215 = Get Variant Attribute(Variant=w989, name=w988, default value (empty Variant)=w983, error in=w987) -> (duplicate Variant=w984:variant, value=w985:dbl[unit], error out=w986:errorcluster)  [unwired: 1 out]
            n216 = To Variant(anything=w985) -> (Variant=w982:variant)
          }
          frame True {
            n217 = Variant To Data(error in=w997, type=w996, Variant=w990) -> (data=w995:dbl[unit], error out=w994:errorcluster)
            n218 = Set Variant Attribute(Variant=w998, name=w993, value=w995, error in=w994) -> (Variant out=w992:variant, error out=w991:errorcluster)  [unwired: 1 out]
          }
        }
        n219 = To Variant(anything=w972) -> (Variant=w973:variant)
      }
      frame "------ Python Plugins ------" {
      }
      frame "Python Plugins:Information" {
        w1002 = T15[] [] ("Array")
        n220 = case shown="False" w1005 {
          tunnel: w1011 -> [w1019 w1028]
          tunnel: w1010 -> [w1018 w1023]
          tunnel: w1009 -> [w1017 w1027]
          tunnel: [w1016 w1021] -> w1008
          tunnel: [w1012 w1020] -> w1007
          tunnel: [w1014 w1022] -> w1006
          tunnel: w1002 -> [w1013 w1026]
          tunnel: w1004 -> [_ w1020]
          frame False {
            n221 = Get Variant Attribute(Variant=w1019, name=w1018, default value (empty Variant)=w1013, error in=w1017) -> (duplicate Variant=w1014:variant, value=w1015:T15[], error out=w1016:errorcluster)  [unwired: 1 out]
            n222 = To Variant(anything=w1015) -> (Variant=w1012:variant)
          }
          frame True {
            n223 = Variant To Data(error in=w1027, type=w1026, Variant=w1020) -> (data=w1025:T15[], error out=w1024:errorcluster)
            n224 = Set Variant Attribute(Variant=w1028, name=w1023, value=w1025, error in=w1024) -> (Variant out=w1022:variant, error out=w1021:errorcluster)  [unwired: 1 out]
          }
        }
        n225 = To Variant(anything=w1002) -> (Variant=w1003:variant)
      }
      frame "Python Plugins:Python Session" {
        w1029 = refnum<k35> refnum ("Python Session")
        n226 = case shown="True" w1032 {
          tunnel: w1038 -> [w1046 w1055]
          tunnel: w1037 -> [w1045 w1050]
          tunnel: w1036 -> [w1044 w1054]
          tunnel: [w1043 w1048] -> w1035
          tunnel: [w1039 w1047] -> w1034
          tunnel: [w1041 w1049] -> w1033
          tunnel: w1029 -> [w1040 w1053]
          tunnel: w1031 -> [_ w1047]
          frame False {
            n227 = Get Variant Attribute(Variant=w1046, name=w1045, default value (empty Variant)=w1040, error in=w1044) -> (duplicate Variant=w1041:variant, value=w1042:refnum<k35>, error out=w1043:errorcluster)  [unwired: 1 out]
            n228 = To Variant(anything=w1042) -> (Variant=w1039:variant)
          }
          frame True {
            n229 = Variant To Data(error in=w1054, type=w1053, Variant=w1047) -> (data=w1052:refnum<k35>, error out=w1051:errorcluster)
            n230 = Set Variant Attribute(Variant=w1055, name=w1050, value=w1052, error in=w1051) -> (Variant out=w1049:variant, error out=w1048:errorcluster)  [unwired: 1 out]
          }
        }
        n231 = To Variant(anything=w1029) -> (Variant=w1030:variant)
      }
      frame "Python Plugins:Valid Python Session?" {
        w1056 = FALSE
        n232 = case shown="True" w1059 {
          tunnel: w1065 -> [w1073 w1082]
          tunnel: w1064 -> [w1072 w1077]
          tunnel: w1063 -> [w1071 w1081]
          tunnel: [w1070 w1075] -> w1062
          tunnel: [w1066 w1074] -> w1061
          tunnel: [w1068 w1076] -> w1060
          tunnel: w1056 -> [w1067 w1080]
          tunnel: w1058 -> [_ w1074]
          frame False {
            n233 = Get Variant Attribute(Variant=w1073, name=w1072, default value (empty Variant)=w1067, error in=w1071) -> (duplicate Variant=w1068:variant, value=w1069:bool, error out=w1070:errorcluster)  [unwired: 1 out]
            n234 = To Variant(anything=w1069) -> (Variant=w1066:variant)
          }
          frame True {
            n235 = Variant To Data(error in=w1081, type=w1080, Variant=w1074) -> (data=w1079:bool, error out=w1078:errorcluster)
            n236 = Set Variant Attribute(Variant=w1082, name=w1077, value=w1079, error in=w1078) -> (Variant out=w1076:variant, error out=w1075:errorcluster)  [unwired: 1 out]
          }
        }
        n237 = To Variant(anything=w1056) -> (Variant=w1057:variant)
      }
      frame "---- Source Image ----" {
      }
      frame "Source Image:ROIs" {
        w1086 = T19[] [] ("ROIs")
        n238 = case shown="True" w1089 {
          tunnel: w1095 -> [w1103 w1112]
          tunnel: w1094 -> [w1102 w1107]
          tunnel: w1093 -> [w1101 w1111]
          tunnel: [w1100 w1105] -> w1092
          tunnel: [w1096 w1104] -> w1091
          tunnel: [w1098 w1106] -> w1090
          tunnel: w1086 -> [w1097 w1110]
          tunnel: w1088 -> [_ w1104]
          frame False {
            n239 = Get Variant Attribute(Variant=w1103, name=w1102, default value (empty Variant)=w1097, error in=w1101) -> (duplicate Variant=w1098:variant, value=w1099:T19[], error out=w1100:errorcluster)  [unwired: 1 out]
            n240 = To Variant(anything=w1099) -> (Variant=w1096:variant)
          }
          frame True {
            n241 = Variant To Data(error in=w1111, type=w1110, Variant=w1104) -> (data=w1109:T19[], error out=w1108:errorcluster)
            n242 = Set Variant Attribute(Variant=w1112, name=w1107, value=w1109, error in=w1108) -> (Variant out=w1106:variant, error out=w1105:errorcluster)  [unwired: 1 out]
          }
        }
        n243 = To Variant(anything=w1086) -> (Variant=w1087:variant)
      }
      frame "Source Image:Current ROI" {
        w1113 = -1  # Current ROI
        n244 = case shown="True" w1116 {
          tunnel: w1122 -> [w1130 w1139]
          tunnel: w1121 -> [w1129 w1134]
          tunnel: w1120 -> [w1128 w1138]
          tunnel: [w1127 w1132] -> w1119
          tunnel: [w1123 w1131] -> w1118
          tunnel: [w1125 w1133] -> w1117
          tunnel: w1113 -> [w1124 w1137]
          tunnel: w1115 -> [_ w1131]
          frame False {
            n245 = Get Variant Attribute(Variant=w1130, name=w1129, default value (empty Variant)=w1124, error in=w1128) -> (duplicate Variant=w1125:variant, value=w1126:i32, error out=w1127:errorcluster)  [unwired: 1 out]
            n246 = To Variant(anything=w1126) -> (Variant=w1123:variant)
          }
          frame True {
            n247 = Variant To Data(error in=w1138, type=w1137, Variant=w1131) -> (data=w1136:i32, error out=w1135:errorcluster)
            n248 = Set Variant Attribute(Variant=w1139, name=w1134, value=w1136, error in=w1135) -> (Variant out=w1133:variant, error out=w1132:errorcluster)  [unwired: 1 out]
          }
        }
        n249 = To Variant(anything=w1113) -> (Variant=w1114:variant)
      }
      frame "Source Image:ROI Event Refnum" {
        w1140 = T20 refnum items=["Undefined", "Delete Current ROI", "Delete All Unselected ROIs", "Delete Multiple ROIs", "Delete All ROIs", "Swap ROIs", "Insert ROI", "Update Current ROI Descriptor", "Rename Current ROI", "Store New ROI", "Store Multiple ROIs", "Select Next ROI", "Select Previous ROI", "Find Selected ROI", "Show All ROIs", "Update ROI Manager Window", "Merge All ROIs", "Unmerge ROI", "Set Selected ROI by ID"]  # Source Image ROI Event Refnum
        n250 = case shown="True" w1143 {
          tunnel: w1149 -> [w1157 w1166]
          tunnel: w1148 -> [w1156 w1161]
          tunnel: w1147 -> [w1155 w1165]
          tunnel: [w1154 w1159] -> w1146
          tunnel: [w1150 w1158] -> w1145
          tunnel: [w1152 w1160] -> w1144
          tunnel: w1140 -> [w1151 w1164]
          tunnel: w1142 -> [_ w1158]
          frame False {
            n251 = Get Variant Attribute(Variant=w1157, name=w1156, default value (empty Variant)=w1151, error in=w1155) -> (duplicate Variant=w1152:variant, value=w1153:T20, error out=w1154:errorcluster)  [unwired: 1 out]
            n252 = To Variant(anything=w1153) -> (Variant=w1150:variant)
          }
          frame True {
            n253 = Variant To Data(error in=w1165, type=w1164, Variant=w1158) -> (data=w1163:T20, error out=w1162:errorcluster)
            n254 = Set Variant Attribute(Variant=w1166, name=w1161, value=w1163, error in=w1162) -> (Variant out=w1160:variant, error out=w1159:errorcluster)  [unwired: 1 out]
          }
        }
        n255 = To Variant(anything=w1140) -> (Variant=w1141:variant)
      }
      frame "X_Source Image Display Range" {
        w1167 = cluster{"Min Value":dbl, "Max Value":dbl} {"Min Value"=-inf, "Max Value"=inf}  # Source Image Display Range
        n256 = case shown="True" w1170 {
          tunnel: w1176 -> [w1184 w1193]
          tunnel: w1175 -> [w1183 w1188]
          tunnel: w1174 -> [w1182 w1192]
          tunnel: [w1181 w1186] -> w1173
          tunnel: [w1177 w1185] -> w1172
          tunnel: [w1179 w1187] -> w1171
          tunnel: w1167 -> [w1178 w1191]
          tunnel: w1169 -> [_ w1185]
          frame False {
            n257 = Get Variant Attribute(Variant=w1184, name=w1183, default value (empty Variant)=w1178, error in=w1182) -> (duplicate Variant=w1179:variant, value=w1180:cluster{"Min Value":dbl, "Max Value":dbl}, error out=w1181:errorcluster)  [unwired: 1 out]
            n258 = To Variant(anything=w1180) -> (Variant=w1177:variant)
          }
          frame True {
            n259 = Variant To Data(error in=w1192, type=w1191, Variant=w1185) -> (data=w1190:cluster{"Min Value":dbl, "Max Value":dbl}, error out=w1189:errorcluster)
            n260 = Set Variant Attribute(Variant=w1193, name=w1188, value=w1190, error in=w1189) -> (Variant out=w1187:variant, error out=w1186:errorcluster)  [unwired: 1 out]
          }
        }
        n261 = To Variant(anything=w1167) -> (Variant=w1168:variant)
      }
      frame "X_Source Image Palette Information" {
        w1194 = T21 {"Palette Name [# Colors,int?,inv?]"="", "Palette Type"=0, "Palette Colors"=[], "Interpolate?"=FALSE} ("Image Display Palette Information")
        n262 = case shown="True" w1197 {
          tunnel: w1203 -> [w1211 w1220]
          tunnel: w1202 -> [w1210 w1215]
          tunnel: w1201 -> [w1209 w1219]
          tunnel: [w1208 w1213] -> w1200
          tunnel: [w1204 w1212] -> w1199
          tunnel: [w1206 w1214] -> w1198
          tunnel: w1194 -> [w1205 w1218]
          tunnel: w1196 -> [_ w1212]
          frame False {
            n263 = Get Variant Attribute(Variant=w1211, name=w1210, default value (empty Variant)=w1205, error in=w1209) -> (duplicate Variant=w1206:variant, value=w1207:T21, error out=w1208:errorcluster)  [unwired: 1 out]
            n264 = To Variant(anything=w1207) -> (Variant=w1204:variant)
          }
          frame True {
            n265 = Variant To Data(error in=w1219, type=w1218, Variant=w1212) -> (data=w1217:T21, error out=w1216:errorcluster)
            n266 = Set Variant Attribute(Variant=w1220, name=w1215, value=w1217, error in=w1216) -> (Variant out=w1214:variant, error out=w1213:errorcluster)  [unwired: 1 out]
          }
        }
        n267 = To Variant(anything=w1194) -> (Variant=w1195:variant)
      }
      frame "X_Type of Displayed Image" {
        w1221 = AlliGator_Displayed_Image."Sum of All Gates" ("Displayed Image")
        n268 = case shown="True" w1224 {
          tunnel: w1230 -> [w1238 w1247]
          tunnel: w1229 -> [w1237 w1242]
          tunnel: w1228 -> [w1236 w1246]
          tunnel: [w1235 w1240] -> w1227
          tunnel: [w1231 w1239] -> w1226
          tunnel: [w1233 w1241] -> w1225
          tunnel: w1221 -> [w1232 w1245]
          tunnel: w1223 -> [_ w1239]
          frame False {
            n269 = Get Variant Attribute(Variant=w1238, name=w1237, default value (empty Variant)=w1232, error in=w1236) -> (duplicate Variant=w1233:variant, value=w1234:T23, error out=w1235:errorcluster)  [unwired: 1 out]
            n270 = To Variant(anything=w1234) -> (Variant=w1231:variant)
          }
          frame True {
            n271 = Variant To Data(error in=w1246, type=w1245, Variant=w1239) -> (data=w1244:T23, error out=w1243:errorcluster)
            n272 = Set Variant Attribute(Variant=w1247, name=w1242, value=w1244, error in=w1243) -> (Variant out=w1241:variant, error out=w1240:errorcluster)  [unwired: 1 out]
          }
        }
        n273 = To Variant(anything=w1221) -> (Variant=w1222:variant)
      }
      frame "X_Time Gate Slider" {
        w1248 = u16 0
        n274 = case shown="True" w1251 {
          tunnel: w1257 -> [w1265 w1274]
          tunnel: w1256 -> [w1264 w1269]
          tunnel: w1255 -> [w1263 w1273]
          tunnel: [w1262 w1267] -> w1254
          tunnel: [w1258 w1266] -> w1253
          tunnel: [w1260 w1268] -> w1252
          tunnel: w1248 -> [w1259 w1272]
          tunnel: w1250 -> [_ w1266]
          frame False {
            n275 = Get Variant Attribute(Variant=w1265, name=w1264, default value (empty Variant)=w1259, error in=w1263) -> (duplicate Variant=w1260:variant, value=w1261:u16, error out=w1262:errorcluster)  [unwired: 1 out]
            n276 = To Variant(anything=w1261) -> (Variant=w1258:variant)
          }
          frame True {
            n277 = Variant To Data(error in=w1273, type=w1272, Variant=w1266) -> (data=w1271:u16, error out=w1270:errorcluster)
            n278 = Set Variant Attribute(Variant=w1274, name=w1269, value=w1271, error in=w1270) -> (Variant out=w1268:variant, error out=w1267:errorcluster)  [unwired: 1 out]
          }
        }
        n279 = To Variant(anything=w1248) -> (Variant=w1249:variant)
      }
      frame "Source Image:Palette List" {
        w1275 = string[] []  # Source Image Palette List
        n280 = case shown="True" w1278 {
          tunnel: w1284 -> [w1292 w1301]
          tunnel: w1283 -> [w1291 w1296]
          tunnel: w1282 -> [w1290 w1300]
          tunnel: [w1289 w1294] -> w1281
          tunnel: [w1285 w1293] -> w1280
          tunnel: [w1287 w1295] -> w1279
          tunnel: w1275 -> [w1286 w1299]
          tunnel: w1277 -> [_ w1293]
          frame False {
            n281 = Get Variant Attribute(Variant=w1292, name=w1291, default value (empty Variant)=w1286, error in=w1290) -> (duplicate Variant=w1287:variant, value=w1288:string[], error out=w1289:errorcluster)  [unwired: 1 out]
            n282 = To Variant(anything=w1288) -> (Variant=w1285:variant)
          }
          frame True {
            n283 = Variant To Data(error in=w1300, type=w1299, Variant=w1293) -> (data=w1298:string[], error out=w1297:errorcluster)
            n284 = Set Variant Attribute(Variant=w1301, name=w1296, value=w1298, error in=w1297) -> (Variant out=w1295:variant, error out=w1294:errorcluster)  [unwired: 1 out]
          }
        }
        n285 = To Variant(anything=w1275) -> (Variant=w1276:variant)
      }
      frame "Source Image:Scale" {
        w1302 = Image_Zoom_Factor."Zoom to Fit"
        n286 = case shown="True" w1305 {
          tunnel: w1311 -> [w1319 w1328]
          tunnel: w1310 -> [w1318 w1323]
          tunnel: w1309 -> [w1317 w1327]
          tunnel: [w1316 w1321] -> w1308
          tunnel: [w1312 w1320] -> w1307
          tunnel: [w1314 w1322] -> w1306
          tunnel: w1302 -> [w1313 w1326]
          tunnel: w1304 -> [_ w1320]
          frame False {
            n287 = Get Variant Attribute(Variant=w1319, name=w1318, default value (empty Variant)=w1313, error in=w1317) -> (duplicate Variant=w1314:variant, value=w1315:T24, error out=w1316:errorcluster)  [unwired: 1 out]
            n288 = To Variant(anything=w1315) -> (Variant=w1312:variant)
          }
          frame True {
            n289 = Variant To Data(error in=w1327, type=w1326, Variant=w1320) -> (data=w1325:T24, error out=w1324:errorcluster)
            n290 = Set Variant Attribute(Variant=w1328, name=w1323, value=w1325, error in=w1324) -> (Variant out=w1322:variant, error out=w1321:errorcluster)  [unwired: 1 out]
          }
        }
        n291 = To Variant(anything=w1302) -> (Variant=w1303:variant)
      }
      frame "Source Image:ROI Overlay Color" {
        w1329 = u32 6618880
        n292 = case shown="True" w1332 {
          tunnel: w1338 -> [w1346 w1355]
          tunnel: w1337 -> [w1345 w1350]
          tunnel: w1336 -> [w1344 w1354]
          tunnel: [w1343 w1348] -> w1335
          tunnel: [w1339 w1347] -> w1334
          tunnel: [w1341 w1349] -> w1333
          tunnel: w1329 -> [w1340 w1353]
          tunnel: w1331 -> [_ w1347]
          frame False {
            n293 = Get Variant Attribute(Variant=w1346, name=w1345, default value (empty Variant)=w1340, error in=w1344) -> (duplicate Variant=w1341:variant, value=w1342:u32, error out=w1343:errorcluster)  [unwired: 1 out]
            n294 = To Variant(anything=w1342) -> (Variant=w1339:variant)
          }
          frame True {
            n295 = Variant To Data(error in=w1354, type=w1353, Variant=w1347) -> (data=w1352:u32, error out=w1351:errorcluster)
            n296 = Set Variant Attribute(Variant=w1355, name=w1350, value=w1352, error in=w1351) -> (Variant out=w1349:variant, error out=w1348:errorcluster)  [unwired: 1 out]
          }
        }
        n297 = To Variant(anything=w1329) -> (Variant=w1330:variant)
      }
      frame "Source Image:Overlay to Erase" {
        w1356 = string[] []  # Source Image Overlay Groups
        n298 = case shown="True" w1359 {
          tunnel: w1365 -> [w1373 w1382]
          tunnel: w1364 -> [w1372 w1377]
          tunnel: w1363 -> [w1371 w1381]
          tunnel: [w1370 w1375] -> w1362
          tunnel: [w1366 w1374] -> w1361
          tunnel: [w1368 w1376] -> w1360
          tunnel: w1356 -> [w1367 w1380]
          tunnel: w1358 -> [_ w1374]
          frame False {
            n299 = Get Variant Attribute(Variant=w1373, name=w1372, default value (empty Variant)=w1367, error in=w1371) -> (duplicate Variant=w1368:variant, value=w1369:string[], error out=w1370:errorcluster)  [unwired: 1 out]
            n300 = To Variant(anything=w1369) -> (Variant=w1366:variant)
          }
          frame True {
            n301 = Variant To Data(error in=w1381, type=w1380, Variant=w1374) -> (data=w1379:string[], error out=w1378:errorcluster)
            n302 = Set Variant Attribute(Variant=w1382, name=w1377, value=w1379, error in=w1378) -> (Variant out=w1376:variant, error out=w1375:errorcluster)  [unwired: 1 out]
          }
        }
        n303 = To Variant(anything=w1356) -> (Variant=w1357:variant)
      }
      frame "Source Image:Is Displayed Image Accumulated" {
        w1383 = FALSE  # Is Displayed Image Accumulated
        n304 = case shown="True" w1386 {
          tunnel: w1392 -> [w1400 w1409]
          tunnel: w1391 -> [w1399 w1404]
          tunnel: w1390 -> [w1398 w1408]
          tunnel: [w1397 w1402] -> w1389
          tunnel: [w1393 w1401] -> w1388
          tunnel: [w1395 w1403] -> w1387
          tunnel: w1383 -> [w1394 w1407]
          tunnel: w1385 -> [_ w1401]
          frame False {
            n305 = Get Variant Attribute(Variant=w1400, name=w1399, default value (empty Variant)=w1394, error in=w1398) -> (duplicate Variant=w1395:variant, value=w1396:bool, error out=w1397:errorcluster)  [unwired: 1 out]
            n306 = To Variant(anything=w1396) -> (Variant=w1393:variant)
          }
          frame True {
            n307 = Variant To Data(error in=w1408, type=w1407, Variant=w1401) -> (data=w1406:bool, error out=w1405:errorcluster)
            n308 = Set Variant Attribute(Variant=w1409, name=w1404, value=w1406, error in=w1405) -> (Variant out=w1403:variant, error out=w1402:errorcluster)  [unwired: 1 out]
          }
        }
        n309 = To Variant(anything=w1383) -> (Variant=w1384:variant)
      }
      frame "Source Image:White Light Image Modified" {
        w1410 = FALSE  # White Light Image Modified
        n310 = case shown="True" w1413 {
          tunnel: w1419 -> [w1427 w1436]
          tunnel: w1418 -> [w1426 w1431]
          tunnel: w1417 -> [w1425 w1435]
          tunnel: [w1424 w1429] -> w1416
          tunnel: [w1420 w1428] -> w1415
          tunnel: [w1422 w1430] -> w1414
          tunnel: w1410 -> [w1421 w1434]
          tunnel: w1412 -> [_ w1428]
          frame False {
            n311 = Get Variant Attribute(Variant=w1427, name=w1426, default value (empty Variant)=w1421, error in=w1425) -> (duplicate Variant=w1422:variant, value=w1423:bool, error out=w1424:errorcluster)  [unwired: 1 out]
            n312 = To Variant(anything=w1423) -> (Variant=w1420:variant)
          }
          frame True {
            n313 = Variant To Data(error in=w1435, type=w1434, Variant=w1428) -> (data=w1433:bool, error out=w1432:errorcluster)
            n314 = Set Variant Attribute(Variant=w1436, name=w1431, value=w1433, error in=w1432) -> (Variant out=w1430:variant, error out=w1429:errorcluster)  [unwired: 1 out]
          }
        }
        n315 = To Variant(anything=w1410) -> (Variant=w1411:variant)
      }
      frame "Source Image:Mask Image Modified" {
        w1437 = FALSE  # Image Mask Modified
        n316 = case shown="True" w1440 {
          tunnel: w1446 -> [w1454 w1463]
          tunnel: w1445 -> [w1453 w1458]
          tunnel: w1444 -> [w1452 w1462]
          tunnel: [w1451 w1456] -> w1443
          tunnel: [w1447 w1455] -> w1442
          tunnel: [w1449 w1457] -> w1441
          tunnel: w1437 -> [w1448 w1461]
          tunnel: w1439 -> [_ w1455]
          frame False {
            n317 = Get Variant Attribute(Variant=w1454, name=w1453, default value (empty Variant)=w1448, error in=w1452) -> (duplicate Variant=w1449:variant, value=w1450:bool, error out=w1451:errorcluster)  [unwired: 1 out]
            n318 = To Variant(anything=w1450) -> (Variant=w1447:variant)
          }
          frame True {
            n319 = Variant To Data(error in=w1462, type=w1461, Variant=w1455) -> (data=w1460:bool, error out=w1459:errorcluster)
            n320 = Set Variant Attribute(Variant=w1463, name=w1458, value=w1460, error in=w1459) -> (Variant out=w1457:variant, error out=w1456:errorcluster)  [unwired: 1 out]
          }
        }
        n321 = To Variant(anything=w1437) -> (Variant=w1438:variant)
      }
      frame "---- Image Profile Window ----" {
      }
      frame "Image Profile:Window Event Refnum" {
        w1467 = refnum<user-event> refnum  # Source Image Profile Window Event Refnum
        n322 = case shown="True" w1470 {
          tunnel: w1476 -> [w1484 w1493]
          tunnel: w1475 -> [w1483 w1488]
          tunnel: w1474 -> [w1482 w1492]
          tunnel: [w1481 w1486] -> w1473
          tunnel: [w1477 w1485] -> w1472
          tunnel: [w1479 w1487] -> w1471
          tunnel: w1467 -> [w1478 w1491]
          tunnel: w1469 -> [_ w1485]
          frame False {
            n323 = Get Variant Attribute(Variant=w1484, name=w1483, default value (empty Variant)=w1478, error in=w1482) -> (duplicate Variant=w1479:variant, value=w1480:refnum<user-event>, error out=w1481:errorcluster)  [unwired: 1 out]
            n324 = To Variant(anything=w1480) -> (Variant=w1477:variant)
          }
          frame True {
            n325 = Variant To Data(error in=w1492, type=w1491, Variant=w1485) -> (data=w1490:refnum<user-event>, error out=w1489:errorcluster)
            n326 = Set Variant Attribute(Variant=w1493, name=w1488, value=w1490, error in=w1489) -> (Variant out=w1487:variant, error out=w1486:errorcluster)  [unwired: 1 out]
          }
        }
        n327 = To Variant(anything=w1467) -> (Variant=w1468:variant)
      }
      frame "Image Profile:IntensityType" {
        w1494 = AlliGator_Image_Profile_Intensity_Type."Raw Data" ("Image Profile Intensity Type")
        n328 = case shown="True" w1497 {
          tunnel: w1503 -> [w1511 w1520]
          tunnel: w1502 -> [w1510 w1515]
          tunnel: w1501 -> [w1509 w1519]
          tunnel: [w1508 w1513] -> w1500
          tunnel: [w1504 w1512] -> w1499
          tunnel: [w1506 w1514] -> w1498
          tunnel: w1494 -> [w1505 w1518]
          tunnel: w1496 -> [_ w1512]
          frame False {
            n329 = Get Variant Attribute(Variant=w1511, name=w1510, default value (empty Variant)=w1505, error in=w1509) -> (duplicate Variant=w1506:variant, value=w1507:T25, error out=w1508:errorcluster)  [unwired: 1 out]
            n330 = To Variant(anything=w1507) -> (Variant=w1504:variant)
          }
          frame True {
            n331 = Variant To Data(error in=w1519, type=w1518, Variant=w1512) -> (data=w1517:T25, error out=w1516:errorcluster)
            n332 = Set Variant Attribute(Variant=w1520, name=w1515, value=w1517, error in=w1516) -> (Variant out=w1514:variant, error out=w1513:errorcluster)  [unwired: 1 out]
          }
        }
        n333 = To Variant(anything=w1494) -> (Variant=w1495:variant)
      }
      frame "Image Profile:Intensity Average Type" {
        w1521 = AlliGator_Image_Profile_Average_Intensity_Type."Integrated Intensity"
        n334 = case shown="False" w1524 {
          tunnel: w1530 -> [w1538 w1547]
          tunnel: w1529 -> [w1537 w1542]
          tunnel: w1528 -> [w1536 w1546]
          tunnel: [w1535 w1540] -> w1527
          tunnel: [w1531 w1539] -> w1526
          tunnel: [w1533 w1541] -> w1525
          tunnel: w1521 -> [w1532 w1545]
          tunnel: w1523 -> [_ w1539]
          frame False {
            n335 = Get Variant Attribute(Variant=w1538, name=w1537, default value (empty Variant)=w1532, error in=w1536) -> (duplicate Variant=w1533:variant, value=w1534:T26, error out=w1535:errorcluster)  [unwired: 1 out]
            n336 = To Variant(anything=w1534) -> (Variant=w1531:variant)
          }
          frame True {
            n337 = Variant To Data(error in=w1546, type=w1545, Variant=w1539) -> (data=w1544:T26, error out=w1543:errorcluster)
            n338 = Set Variant Attribute(Variant=w1547, name=w1542, value=w1544, error in=w1543) -> (Variant out=w1541:variant, error out=w1540:errorcluster)  [unwired: 1 out]
          }
        }
        n339 = To Variant(anything=w1521) -> (Variant=w1522:variant)
      }
      frame "Image Profile:Intensity-weighted SDV" {
        w1548 = TRUE
        n340 = case shown="True" w1551 {
          tunnel: w1557 -> [w1565 w1574]
          tunnel: w1556 -> [w1564 w1569]
          tunnel: w1555 -> [w1563 w1573]
          tunnel: [w1562 w1567] -> w1554
          tunnel: [w1558 w1566] -> w1553
          tunnel: [w1560 w1568] -> w1552
          tunnel: w1548 -> [w1559 w1572]
          tunnel: w1550 -> [_ w1566]
          frame False {
            n341 = Get Variant Attribute(Variant=w1565, name=w1564, default value (empty Variant)=w1559, error in=w1563) -> (duplicate Variant=w1560:variant, value=w1561:bool, error out=w1562:errorcluster)  [unwired: 1 out]
            n342 = To Variant(anything=w1561) -> (Variant=w1558:variant)
          }
          frame True {
            n343 = Variant To Data(error in=w1573, type=w1572, Variant=w1566) -> (data=w1571:bool, error out=w1570:errorcluster)
            n344 = Set Variant Attribute(Variant=w1574, name=w1569, value=w1571, error in=w1570) -> (Variant out=w1568:variant, error out=w1567:errorcluster)  [unwired: 1 out]
          }
        }
        n345 = To Variant(anything=w1548) -> (Variant=w1549:variant)
      }
      frame "Image Profile:Box Profile Type" {
        w1575 = Box_Profile_Type."Full Width"
        n346 = case shown="True" w1578 {
          tunnel: w1584 -> [w1592 w1601]
          tunnel: w1583 -> [w1591 w1596]
          tunnel: w1582 -> [w1590 w1600]
          tunnel: [w1589 w1594] -> w1581
          tunnel: [w1585 w1593] -> w1580
          tunnel: [w1587 w1595] -> w1579
          tunnel: w1575 -> [w1586 w1599]
          tunnel: w1577 -> [_ w1593]
          frame False {
            n347 = Get Variant Attribute(Variant=w1592, name=w1591, default value (empty Variant)=w1586, error in=w1590) -> (duplicate Variant=w1587:variant, value=w1588:T27, error out=w1589:errorcluster)  [unwired: 1 out]
            n348 = To Variant(anything=w1588) -> (Variant=w1585:variant)
          }
          frame True {
            n349 = Variant To Data(error in=w1600, type=w1599, Variant=w1593) -> (data=w1598:T27, error out=w1597:errorcluster)
            n350 = Set Variant Attribute(Variant=w1601, name=w1596, value=w1598, error in=w1597) -> (Variant out=w1595:variant, error out=w1594:errorcluster)  [unwired: 1 out]
          }
        }
        n351 = To Variant(anything=w1575) -> (Variant=w1576:variant)
      }
      frame "Image Profile:Window Open" {
        w1602 = FALSE ("Get(F)/Set")
        n352 = case shown="True" w1605 {
          tunnel: w1611 -> [w1619 w1628]
          tunnel: w1610 -> [w1618 w1623]
          tunnel: w1609 -> [w1617 w1627]
          tunnel: [w1616 w1621] -> w1608
          tunnel: [w1612 w1620] -> w1607
          tunnel: [w1614 w1622] -> w1606
          tunnel: w1602 -> [w1613 w1626]
          tunnel: w1604 -> [_ w1620]
          frame False {
            n353 = Get Variant Attribute(Variant=w1619, name=w1618, default value (empty Variant)=w1613, error in=w1617) -> (duplicate Variant=w1614:variant, value=w1615:bool, error out=w1616:errorcluster)  [unwired: 1 out]
            n354 = To Variant(anything=w1615) -> (Variant=w1612:variant)
          }
          frame True {
            n355 = Variant To Data(error in=w1627, type=w1626, Variant=w1620) -> (data=w1625:bool, error out=w1624:errorcluster)
            n356 = Set Variant Attribute(Variant=w1628, name=w1623, value=w1625, error in=w1624) -> (Variant out=w1622:variant, error out=w1621:errorcluster)  [unwired: 1 out]
          }
        }
        n357 = To Variant(anything=w1602) -> (Variant=w1603:variant)
      }
      frame "Image Profile:Plotted Fit Parameter" {
        w1629 = Decay_Fit_Parameters_&_Derived_Quantities_List_v2."Offset" ("Fit Parameter")
        n358 = case shown="True" w1632 {
          tunnel: w1638 -> [w1646 w1655]
          tunnel: w1637 -> [w1645 w1650]
          tunnel: w1636 -> [w1644 w1654]
          tunnel: [w1643 w1648] -> w1635
          tunnel: [w1639 w1647] -> w1634
          tunnel: [w1641 w1649] -> w1633
          tunnel: w1629 -> [w1640 w1653]
          tunnel: w1631 -> [_ w1647]
          frame False {
            n359 = Get Variant Attribute(Variant=w1646, name=w1645, default value (empty Variant)=w1640, error in=w1644) -> (duplicate Variant=w1641:variant, value=w1642:T28, error out=w1643:errorcluster)  [unwired: 1 out]
            n360 = To Variant(anything=w1642) -> (Variant=w1639:variant)
          }
          frame True {
            n361 = Variant To Data(error in=w1654, type=w1653, Variant=w1647) -> (data=w1652:T28, error out=w1651:errorcluster)
            n362 = Set Variant Attribute(Variant=w1655, name=w1650, value=w1652, error in=w1651) -> (Variant out=w1649:variant, error out=w1648:errorcluster)  [unwired: 1 out]
          }
        }
        n363 = To Variant(anything=w1629) -> (Variant=w1630:variant)
      }
      frame "------ Phasor Graph -------" {
      }
      frame "Phasor Graph:Show Line" {
        w1659 = FALSE
        n364 = case shown="True" w1662 {
          tunnel: w1668 -> [w1676 w1685]
          tunnel: w1667 -> [w1675 w1680]
          tunnel: w1666 -> [w1674 w1684]
          tunnel: [w1673 w1678] -> w1665
          tunnel: [w1669 w1677] -> w1664
          tunnel: [w1671 w1679] -> w1663
          tunnel: w1659 -> [w1670 w1683]
          tunnel: w1661 -> [_ w1677]
          frame False {
            n365 = Get Variant Attribute(Variant=w1676, name=w1675, default value (empty Variant)=w1670, error in=w1674) -> (duplicate Variant=w1671:variant, value=w1672:bool, error out=w1673:errorcluster)  [unwired: 1 out]
            n366 = To Variant(anything=w1672) -> (Variant=w1669:variant)
          }
          frame True {
            n367 = Variant To Data(error in=w1684, type=w1683, Variant=w1677) -> (data=w1682:bool, error out=w1681:errorcluster)
            n368 = Set Variant Attribute(Variant=w1685, name=w1680, value=w1682, error in=w1681) -> (Variant out=w1679:variant, error out=w1678:errorcluster)  [unwired: 1 out]
          }
        }
        n369 = To Variant(anything=w1659) -> (Variant=w1660:variant)
      }
      frame "---- Phasor Plot ---" {
      }
      frame "Phasor Plot:Parameters Changed" {
        w1689 = FALSE
        # "set to true when a new dataset is loaded or param chgd\nset to false the first time the phasor plot is calculated"
        n370 = case shown="True" w1692 {
          tunnel: w1698 -> [w1706 w1715]
          tunnel: w1697 -> [w1705 w1710]
          tunnel: w1696 -> [w1704 w1714]
          tunnel: [w1703 w1708] -> w1695
          tunnel: [w1699 w1707] -> w1694
          tunnel: [w1701 w1709] -> w1693
          tunnel: w1689 -> [w1700 w1713]
          tunnel: w1691 -> [_ w1707]
          frame False {
            n371 = Get Variant Attribute(Variant=w1706, name=w1705, default value (empty Variant)=w1700, error in=w1704) -> (duplicate Variant=w1701:variant, value=w1702:bool, error out=w1703:errorcluster)  [unwired: 1 out]
            n372 = To Variant(anything=w1702) -> (Variant=w1699:variant)
          }
          frame True {
            n373 = Variant To Data(error in=w1714, type=w1713, Variant=w1707) -> (data=w1712:bool, error out=w1711:errorcluster)
            n374 = Set Variant Attribute(Variant=w1715, name=w1710, value=w1712, error in=w1711) -> (Variant out=w1709:variant, error out=w1708:errorcluster)  [unwired: 1 out]
          }
        }
        n375 = To Variant(anything=w1689) -> (Variant=w1690:variant)
      }
      frame "Phasor Plot:FLI Dataset Modified since last Calculation" {
        w1716 = FALSE  # FLI Dataset Modified
        n376 = case shown="True" w1719 {
          tunnel: w1725 -> [w1733 w1742]
          tunnel: w1724 -> [w1732 w1737]
          tunnel: w1723 -> [w1731 w1741]
          tunnel: [w1730 w1735] -> w1722
          tunnel: [w1726 w1734] -> w1721
          tunnel: [w1728 w1736] -> w1720
          tunnel: w1716 -> [w1727 w1740]
          tunnel: w1718 -> [_ w1734]
          frame False {
            n377 = Get Variant Attribute(Variant=w1733, name=w1732, default value (empty Variant)=w1727, error in=w1731) -> (duplicate Variant=w1728:variant, value=w1729:bool, error out=w1730:errorcluster)  [unwired: 1 out]
            n378 = To Variant(anything=w1729) -> (Variant=w1726:variant)
          }
          frame True {
            n379 = Variant To Data(error in=w1741, type=w1740, Variant=w1734) -> (data=w1739:bool, error out=w1738:errorcluster)
            n380 = Set Variant Attribute(Variant=w1742, name=w1737, value=w1739, error in=w1738) -> (Variant out=w1736:variant, error out=w1735:errorcluster)  [unwired: 1 out]
          }
        }
        n381 = To Variant(anything=w1716) -> (Variant=w1717:variant)
      }
      frame "Phasor Harmonics Data" {
        w1743 = T29[] [] ("Stored ROIs in")
        n382 = case shown="True" w1746 {
          tunnel: w1752 -> [w1760 w1769]
          tunnel: w1751 -> [w1759 w1764]
          tunnel: w1750 -> [w1758 w1768]
          tunnel: [w1757 w1762] -> w1749
          tunnel: [w1753 w1761] -> w1748
          tunnel: [w1755 w1763] -> w1747
          tunnel: w1743 -> [w1754 w1767]
          tunnel: w1745 -> [_ w1761]
          frame False {
            n383 = Get Variant Attribute(Variant=w1760, name=w1759, default value (empty Variant)=w1754, error in=w1758) -> (duplicate Variant=w1755:variant, value=w1756:T29[], error out=w1757:errorcluster)  [unwired: 1 out]
            n384 = To Variant(anything=w1756) -> (Variant=w1753:variant)
          }
          frame True {
            n385 = Variant To Data(error in=w1768, type=w1767, Variant=w1761) -> (data=w1766:T29[], error out=w1765:errorcluster)
            n386 = Set Variant Attribute(Variant=w1769, name=w1764, value=w1766, error in=w1765) -> (Variant out=w1763:variant, error out=w1762:errorcluster)  [unwired: 1 out]
          }
        }
        n387 = To Variant(anything=w1743) -> (Variant=w1744:variant)
      }
      frame "Selected Phasor Harmonics" {
        w1770 = i32[] []
        n388 = case shown="True" w1773 {
          tunnel: w1779 -> [w1787 w1796]
          tunnel: w1778 -> [w1786 w1791]
          tunnel: w1777 -> [w1785 w1795]
          tunnel: [w1784 w1789] -> w1776
          tunnel: [w1780 w1788] -> w1775
          tunnel: [w1782 w1790] -> w1774
          tunnel: w1770 -> [w1781 w1794]
          tunnel: w1772 -> [_ w1788]
          frame False {
            n389 = Get Variant Attribute(Variant=w1787, name=w1786, default value (empty Variant)=w1781, error in=w1785) -> (duplicate Variant=w1782:variant, value=w1783:i32[], error out=w1784:errorcluster)  [unwired: 1 out]
            n390 = To Variant(anything=w1783) -> (Variant=w1780:variant)
          }
          frame True {
            n391 = Variant To Data(error in=w1795, type=w1794, Variant=w1788) -> (data=w1793:i32[], error out=w1792:errorcluster)
            n392 = Set Variant Attribute(Variant=w1796, name=w1791, value=w1793, error in=w1792) -> (Variant out=w1790:variant, error out=w1789:errorcluster)  [unwired: 1 out]
          }
        }
        n393 = To Variant(anything=w1770) -> (Variant=w1771:variant)
      }
      frame "Phasor Harmonic Manager Event Refnum" {
        w1797 = T30 refnum items=["Undefined", "Delete Current Harmonic", "Delete Multiple Harmonics", "Delete All Harmonics", "Swap Harmonics", "Insert Harmonics", "Rename Current Harmonic", "Store New Harmonic", "Store Multiple Harmonics", "Select Next Harmonic", "Select Previous Harmonic", "Update Phasor Harmonic Manager Window"] ("Phasor Harmonic Manager Event Refnum")
        n394 = case shown="True" w1800 {
          tunnel: w1806 -> [w1814 w1823]
          tunnel: w1805 -> [w1813 w1818]
          tunnel: w1804 -> [w1812 w1822]
          tunnel: [w1811 w1816] -> w1803
          tunnel: [w1807 w1815] -> w1802
          tunnel: [w1809 w1817] -> w1801
          tunnel: w1797 -> [w1808 w1821]
          tunnel: w1799 -> [_ w1815]
          frame False {
            n395 = Get Variant Attribute(Variant=w1814, name=w1813, default value (empty Variant)=w1808, error in=w1812) -> (duplicate Variant=w1809:variant, value=w1810:T30, error out=w1811:errorcluster)  [unwired: 1 out]
            n396 = To Variant(anything=w1810) -> (Variant=w1807:variant)
          }
          frame True {
            n397 = Variant To Data(error in=w1822, type=w1821, Variant=w1815) -> (data=w1820:T30, error out=w1819:errorcluster)
            n398 = Set Variant Attribute(Variant=w1823, name=w1818, value=w1820, error in=w1819) -> (Variant out=w1817:variant, error out=w1816:errorcluster)  [unwired: 1 out]
          }
        }
        n399 = To Variant(anything=w1797) -> (Variant=w1798:variant)
      }
      frame "Phasor Plot:ROIs" {
        w1824 = T19[] [] ("ROIs")
        n400 = case shown="True" w1827 {
          tunnel: w1833 -> [w1841 w1850]
          tunnel: w1832 -> [w1840 w1845]
          tunnel: w1831 -> [w1839 w1849]
          tunnel: [w1838 w1843] -> w1830
          tunnel: [w1834 w1842] -> w1829
          tunnel: [w1836 w1844] -> w1828
          tunnel: w1824 -> [w1835 w1848]
          tunnel: w1826 -> [_ w1842]
          frame False {
            n401 = Get Variant Attribute(Variant=w1841, name=w1840, default value (empty Variant)=w1835, error in=w1839) -> (duplicate Variant=w1836:variant, value=w1837:T19[], error out=w1838:errorcluster)  [unwired: 1 out]
            n402 = To Variant(anything=w1837) -> (Variant=w1834:variant)
          }
          frame True {
            n403 = Variant To Data(error in=w1849, type=w1848, Variant=w1842) -> (data=w1847:T19[], error out=w1846:errorcluster)
            n404 = Set Variant Attribute(Variant=w1850, name=w1845, value=w1847, error in=w1846) -> (Variant out=w1844:variant, error out=w1843:errorcluster)  [unwired: 1 out]
          }
        }
        n405 = To Variant(anything=w1824) -> (Variant=w1825:variant)
      }
      frame "Phasor Plot:Current ROI" {
        w1851 = -1  # Current ROI
        n406 = case shown="True" w1854 {
          tunnel: w1860 -> [w1868 w1877]
          tunnel: w1859 -> [w1867 w1872]
          tunnel: w1858 -> [w1866 w1876]
          tunnel: [w1865 w1870] -> w1857
          tunnel: [w1861 w1869] -> w1856
          tunnel: [w1863 w1871] -> w1855
          tunnel: w1851 -> [w1862 w1875]
          tunnel: w1853 -> [_ w1869]
          frame False {
            n407 = Get Variant Attribute(Variant=w1868, name=w1867, default value (empty Variant)=w1862, error in=w1866) -> (duplicate Variant=w1863:variant, value=w1864:i32, error out=w1865:errorcluster)  [unwired: 1 out]
            n408 = To Variant(anything=w1864) -> (Variant=w1861:variant)
          }
          frame True {
            n409 = Variant To Data(error in=w1876, type=w1875, Variant=w1869) -> (data=w1874:i32, error out=w1873:errorcluster)
            n410 = Set Variant Attribute(Variant=w1877, name=w1872, value=w1874, error in=w1873) -> (Variant out=w1871:variant, error out=w1870:errorcluster)  [unwired: 1 out]
          }
        }
        n411 = To Variant(anything=w1851) -> (Variant=w1852:variant)
      }
      frame "Phasor Plot:ROI Event Refnum" {
        w1878 = T20 refnum items=["Undefined", "Delete Current ROI", "Delete All Unselected ROIs", "Delete Multiple ROIs", "Delete All ROIs", "Swap ROIs", "Insert ROI", "Update Current ROI Descriptor", "Rename Current ROI", "Store New ROI", "Store Multiple ROIs", "Select Next ROI", "Select Previous ROI", "Find Selected ROI", "Show All ROIs", "Update ROI Manager Window", "Merge All ROIs", "Unmerge ROI", "Set Selected ROI by ID"]  # Phasor Plot ROI Event Refnum
        n412 = case shown="True" w1881 {
          tunnel: w1887 -> [w1895 w1904]
          tunnel: w1886 -> [w1894 w1899]
          tunnel: w1885 -> [w1893 w1903]
          tunnel: [w1892 w1897] -> w1884
          tunnel: [w1888 w1896] -> w1883
          tunnel: [w1890 w1898] -> w1882
          tunnel: w1878 -> [w1889 w1902]
          tunnel: w1880 -> [_ w1896]
          frame False {
            n413 = Get Variant Attribute(Variant=w1895, name=w1894, default value (empty Variant)=w1889, error in=w1893) -> (duplicate Variant=w1890:variant, value=w1891:T20, error out=w1892:errorcluster)  [unwired: 1 out]
            n414 = To Variant(anything=w1891) -> (Variant=w1888:variant)
          }
          frame True {
            n415 = Variant To Data(error in=w1903, type=w1902, Variant=w1896) -> (data=w1901:T20, error out=w1900:errorcluster)
            n416 = Set Variant Attribute(Variant=w1904, name=w1899, value=w1901, error in=w1900) -> (Variant out=w1898:variant, error out=w1897:errorcluster)  [unwired: 1 out]
          }
        }
        n417 = To Variant(anything=w1878) -> (Variant=w1879:variant)
      }
      frame "Phasor Plot:Image Reference Points" {
        w1906 = T31 {"O_h"=0.0, "O_v"=0.0, "1_h"=0.0, "1_v"=0.0} ("Phasor Plot Reference Points")
        n418 = case shown="True" w1908 {
          tunnel: w1914 -> [w1922 w1931]
          tunnel: w1913 -> [w1921 w1926]
          tunnel: w1912 -> [w1920 w1930]
          tunnel: [w1919 w1924] -> w1911
          tunnel: [w1915 w1923] -> w1910
          tunnel: [w1917 w1925] -> w1909
          tunnel: w1906 -> [w1916 w1929]
          tunnel: w1907 -> [_ w1923]
          frame False {
            n419 = Get Variant Attribute(Variant=w1922, name=w1921, default value (empty Variant)=w1916, error in=w1920) -> (duplicate Variant=w1917:variant, value=w1918:T31, error out=w1919:errorcluster)  [unwired: 1 out]
            n420 = To Variant(anything=w1918) -> (Variant=w1915:variant)
          }
          frame True {
            n421 = Variant To Data(error in=w1930, type=w1929, Variant=w1923) -> (data=w1928:T31, error out=w1927:errorcluster)
            n422 = Set Variant Attribute(Variant=w1931, name=w1926, value=w1928, error in=w1927) -> (Variant out=w1925:variant, error out=w1924:errorcluster)  [unwired: 1 out]
          }
        }
        n423 = To Variant(anything=w1906) -> (Variant=w1905:variant)
      }
      frame "Phasor Plot:Computed" {
        w1932 = FALSE
        n424 = case shown="True" w1935 {
          tunnel: w1941 -> [w1949 w1958]
          tunnel: w1940 -> [w1948 w1953]
          tunnel: w1939 -> [w1947 w1957]
          tunnel: [w1946 w1951] -> w1938
          tunnel: [w1942 w1950] -> w1937
          tunnel: [w1944 w1952] -> w1936
          tunnel: w1932 -> [w1943 w1956]
          tunnel: w1934 -> [_ w1950]
          frame False {
            n425 = Get Variant Attribute(Variant=w1949, name=w1948, default value (empty Variant)=w1943, error in=w1947) -> (duplicate Variant=w1944:variant, value=w1945:bool, error out=w1946:errorcluster)  [unwired: 1 out]
            n426 = To Variant(anything=w1945) -> (Variant=w1942:variant)
          }
          frame True {
            n427 = Variant To Data(error in=w1957, type=w1956, Variant=w1950) -> (data=w1955:bool, error out=w1954:errorcluster)
            n428 = Set Variant Attribute(Variant=w1958, name=w1953, value=w1955, error in=w1954) -> (Variant out=w1952:variant, error out=w1951:errorcluster)  [unwired: 1 out]
          }
        }
        n429 = To Variant(anything=w1932) -> (Variant=w1933:variant)
      }
      frame "Phasor Plot:Palette Information" {
        w1959 = T21 {"Palette Name [# Colors,int?,inv?]"="", "Palette Type"=0, "Palette Colors"=[], "Interpolate?"=FALSE} ("Image Display Palette Information")
        n430 = case shown="True" w1962 {
          tunnel: w1968 -> [w1976 w1985]
          tunnel: w1967 -> [w1975 w1980]
          tunnel: w1966 -> [w1974 w1984]
          tunnel: [w1973 w1978] -> w1965
          tunnel: [w1969 w1977] -> w1964
          tunnel: [w1971 w1979] -> w1963
          tunnel: w1959 -> [w1970 w1983]
          tunnel: w1961 -> [_ w1977]
          frame False {
            n431 = Get Variant Attribute(Variant=w1976, name=w1975, default value (empty Variant)=w1970, error in=w1974) -> (duplicate Variant=w1971:variant, value=w1972:T21, error out=w1973:errorcluster)  [unwired: 1 out]
            n432 = To Variant(anything=w1972) -> (Variant=w1969:variant)
          }
          frame True {
            n433 = Variant To Data(error in=w1984, type=w1983, Variant=w1977) -> (data=w1982:T21, error out=w1981:errorcluster)
            n434 = Set Variant Attribute(Variant=w1985, name=w1980, value=w1982, error in=w1981) -> (Variant out=w1979:variant, error out=w1978:errorcluster)  [unwired: 1 out]
          }
        }
        n435 = To Variant(anything=w1959) -> (Variant=w1960:variant)
      }
      frame "Phasor Plot:Palette List" {
        w1986 = string[] []  # Phasor Plot Palette List
        n436 = case shown="True" w1989 {
          tunnel: w1995 -> [w2003 w2012]
          tunnel: w1994 -> [w2002 w2007]
          tunnel: w1993 -> [w2001 w2011]
          tunnel: [w2000 w2005] -> w1992
          tunnel: [w1996 w2004] -> w1991
          tunnel: [w1998 w2006] -> w1990
          tunnel: w1986 -> [w1997 w2010]
          tunnel: w1988 -> [_ w2004]
          frame False {
            n437 = Get Variant Attribute(Variant=w2003, name=w2002, default value (empty Variant)=w1997, error in=w2001) -> (duplicate Variant=w1998:variant, value=w1999:string[], error out=w2000:errorcluster)  [unwired: 1 out]
            n438 = To Variant(anything=w1999) -> (Variant=w1996:variant)
          }
          frame True {
            n439 = Variant To Data(error in=w2011, type=w2010, Variant=w2004) -> (data=w2009:string[], error out=w2008:errorcluster)
            n440 = Set Variant Attribute(Variant=w2012, name=w2007, value=w2009, error in=w2008) -> (Variant out=w2006:variant, error out=w2005:errorcluster)  [unwired: 1 out]
          }
        }
        n441 = To Variant(anything=w1986) -> (Variant=w1987:variant)
      }
      frame "Phasor Plot:Phasor Ratio Palette Information" {
        w2013 = T21 {"Palette Name [# Colors,int?,inv?]"="", "Palette Type"=0, "Palette Colors"=[], "Interpolate?"=FALSE} ("Image Display Palette Information")
        n442 = case shown="True" w2016 {
          tunnel: w2022 -> [w2030 w2039]
          tunnel: w2021 -> [w2029 w2034]
          tunnel: w2020 -> [w2028 w2038]
          tunnel: [w2027 w2032] -> w2019
          tunnel: [w2023 w2031] -> w2018
          tunnel: [w2025 w2033] -> w2017
          tunnel: w2013 -> [w2024 w2037]
          tunnel: w2015 -> [_ w2031]
          frame False {
            n443 = Get Variant Attribute(Variant=w2030, name=w2029, default value (empty Variant)=w2024, error in=w2028) -> (duplicate Variant=w2025:variant, value=w2026:T21, error out=w2027:errorcluster)  [unwired: 1 out]
            n444 = To Variant(anything=w2026) -> (Variant=w2023:variant)
          }
          frame True {
            n445 = Variant To Data(error in=w2038, type=w2037, Variant=w2031) -> (data=w2036:T21, error out=w2035:errorcluster)
            n446 = Set Variant Attribute(Variant=w2039, name=w2034, value=w2036, error in=w2035) -> (Variant out=w2033:variant, error out=w2032:errorcluster)  [unwired: 1 out]
          }
        }
        n447 = To Variant(anything=w2013) -> (Variant=w2014:variant)
      }
      frame "Phasor Plot:Phasor Ratio Palette List" {
        w2040 = string[] []  # Phasor Ratio Palette List
        n448 = case shown="True" w2043 {
          tunnel: w2049 -> [w2057 w2066]
          tunnel: w2048 -> [w2056 w2061]
          tunnel: w2047 -> [w2055 w2065]
          tunnel: [w2054 w2059] -> w2046
          tunnel: [w2050 w2058] -> w2045
          tunnel: [w2052 w2060] -> w2044
          tunnel: w2040 -> [w2051 w2064]
          tunnel: w2042 -> [_ w2058]
          frame False {
            n449 = Get Variant Attribute(Variant=w2057, name=w2056, default value (empty Variant)=w2051, error in=w2055) -> (duplicate Variant=w2052:variant, value=w2053:string[], error out=w2054:errorcluster)  [unwired: 1 out]
            n450 = To Variant(anything=w2053) -> (Variant=w2050:variant)
          }
          frame True {
            n451 = Variant To Data(error in=w2065, type=w2064, Variant=w2058) -> (data=w2063:string[], error out=w2062:errorcluster)
            n452 = Set Variant Attribute(Variant=w2066, name=w2061, value=w2063, error in=w2062) -> (Variant out=w2060:variant, error out=w2059:errorcluster)  [unwired: 1 out]
          }
        }
        n453 = To Variant(anything=w2040) -> (Variant=w2041:variant)
      }
      frame "Phasor Plot:Image Scale" {
        w2067 = Image_Zoom_Factor."Zoom to Fit"
        n454 = case shown="True" w2070 {
          tunnel: w2076 -> [w2084 w2093]
          tunnel: w2075 -> [w2083 w2088]
          tunnel: w2074 -> [w2082 w2092]
          tunnel: [w2081 w2086] -> w2073
          tunnel: [w2077 w2085] -> w2072
          tunnel: [w2079 w2087] -> w2071
          tunnel: w2067 -> [w2078 w2091]
          tunnel: w2069 -> [_ w2085]
          frame False {
            n455 = Get Variant Attribute(Variant=w2084, name=w2083, default value (empty Variant)=w2078, error in=w2082) -> (duplicate Variant=w2079:variant, value=w2080:T24, error out=w2081:errorcluster)  [unwired: 1 out]
            n456 = To Variant(anything=w2080) -> (Variant=w2077:variant)
          }
          frame True {
            n457 = Variant To Data(error in=w2092, type=w2091, Variant=w2085) -> (data=w2090:T24, error out=w2089:errorcluster)
            n458 = Set Variant Attribute(Variant=w2093, name=w2088, value=w2090, error in=w2089) -> (Variant out=w2087:variant, error out=w2086:errorcluster)  [unwired: 1 out]
          }
        }
        n459 = To Variant(anything=w2067) -> (Variant=w2068:variant)
      }
      frame "Phasor Plot:Image Overlay to Erase" {
        w2094 = string[] []  # Phasor Plot Image Overlay Groups
        n460 = case shown="True" w2097 {
          tunnel: w2103 -> [w2111 w2120]
          tunnel: w2102 -> [w2110 w2115]
          tunnel: w2101 -> [w2109 w2119]
          tunnel: [w2108 w2113] -> w2100
          tunnel: [w2104 w2112] -> w2099
          tunnel: [w2106 w2114] -> w2098
          tunnel: w2094 -> [w2105 w2118]
          tunnel: w2096 -> [_ w2112]
          frame False {
            n461 = Get Variant Attribute(Variant=w2111, name=w2110, default value (empty Variant)=w2105, error in=w2109) -> (duplicate Variant=w2106:variant, value=w2107:string[], error out=w2108:errorcluster)  [unwired: 1 out]
            n462 = To Variant(anything=w2107) -> (Variant=w2104:variant)
          }
          frame True {
            n463 = Variant To Data(error in=w2119, type=w2118, Variant=w2112) -> (data=w2117:string[], error out=w2116:errorcluster)
            n464 = Set Variant Attribute(Variant=w2120, name=w2115, value=w2117, error in=w2116) -> (Variant out=w2114:variant, error out=w2113:errorcluster)  [unwired: 1 out]
          }
        }
        n465 = To Variant(anything=w2094) -> (Variant=w2095:variant)
      }
      frame "Phasor Plot:Image Elements to Update" {
        w2121 = string[] []  # Phasor Plot Image Elements to Update
        n466 = case shown="True" w2124 {
          tunnel: w2130 -> [w2138 w2147]
          tunnel: w2129 -> [w2137 w2142]
          tunnel: w2128 -> [w2136 w2146]
          tunnel: [w2135 w2140] -> w2127
          tunnel: [w2131 w2139] -> w2126
          tunnel: [w2133 w2141] -> w2125
          tunnel: w2121 -> [w2132 w2145]
          tunnel: w2123 -> [_ w2139]
          frame False {
            n467 = Get Variant Attribute(Variant=w2138, name=w2137, default value (empty Variant)=w2132, error in=w2136) -> (duplicate Variant=w2133:variant, value=w2134:string[], error out=w2135:errorcluster)  [unwired: 1 out]
            n468 = To Variant(anything=w2134) -> (Variant=w2131:variant)
          }
          frame True {
            n469 = Variant To Data(error in=w2146, type=w2145, Variant=w2139) -> (data=w2144:string[], error out=w2143:errorcluster)
            n470 = Set Variant Attribute(Variant=w2147, name=w2142, value=w2144, error in=w2143) -> (Variant out=w2141:variant, error out=w2140:errorcluster)  [unwired: 1 out]
          }
        }
        n471 = To Variant(anything=w2121) -> (Variant=w2122:variant)
      }
      frame "Phasor Plot:Current Calculation Parameters" {
        w2148 = T32 {"Phasor Frequency"=0.0, "Decay Preprocessing Options & Parameters"={"Background Subtraction Parameters"={"Background Definition Range"={"Min Gate"=0.0, "Max Gate"=0.0}, "Baseline Subtraction Method"=enum."Mean", "Background Subtraction?"=FALSE, "Background File"=path "", "Background Constant"=0.0, "Background Scaling Factor"=1.0, "Background Pile-up Correction"=FALSE, "Background Pixel Well Capacity"=1}, "Decay Preprocessing Parameters"={"Background Subtraction"=FALSE, "Straighten Decay"=FALSE, "Reverse Gates"=FALSE, "1-Normalized Decay"=FALSE, "Smoothen Decay"=FALSE, "Smoothing Parameter"=0.0, "Shift Decay"=FALSE, "Decay Shift Parameters"={"Type"=enum."Default", "Shift"=0.0, "Threshold"=0.0, "Rotate"=FALSE}, "Extrapolate Decay"=FALSE, "Additional Points"=0, "Head Fraction"=0.0, "Pixel-Normalize Decay"=FALSE, "Use Periodicity"=FALSE, "Use Cursors"=FALSE, "Tail Fraction"=0.0, "Use Decay Pre-Processing"=TRUE, "Fold Decay"=FALSE, "# Folds"=1, "[0-1]-Normalized Decay"=FALSE}, "Preprocessing Steps Order"=[]}, "FLI Dataset Modified"=FALSE, "Source Image Settings"={"Low Count Pixels Rejection Options"={"Background Low Threshold Factor"=0.0, "Fixed Low Background Threshold"=0.0, "Reject Low Count Pixels"=FALSE, "Low Percentile"=0.0}, "High Count Pixels Rejection Options"={"Background High Threshold Factor"=0.0, "Fixed High Background Threshold"=20000.0, "Reject High Count Pixels"=FALSE, "High Percentile"=100.0}}, "Data Information"={"Gate Width"=0.0, "Gate Separation"=0.0, "Step (Gate Separation)"=0, "Laser Period"=0.0, "SYNC Period"=0.0, "Channel Name"=0, "Channel Arithmetic"=enum."None", "Pile-up Correction"=FALSE, "Pixel Well Capacity"=1, "Dataset Scaling Factor"=1.0}, "Phasor Plot"={"Phasor Plot Smoothing Options"={"Use Phasor Plot Smoothing"=FALSE, "Kernel Type"=enum."Uniform", "Bin"=1, "Algorithm"=enum."Rapid"}, "Phasor Plot Size"={"H"=0, "V"=0, "Margin"=0.0}, "Selected Image ROI(s)"=FALSE, "All Image ROIs"=FALSE, "Selected Source Image ROI"=0, "Source Image ROIs"=[]}} ("TG Phasor Plot Parameters")
        n472 = case shown="True" w2151 {
          tunnel: w2157 -> [w2165 w2174]
          tunnel: w2156 -> [w2164 w2169]
          tunnel: w2155 -> [w2163 w2173]
          tunnel: [w2162 w2167] -> w2154
          tunnel: [w2158 w2166] -> w2153
          tunnel: [w2160 w2168] -> w2152
          tunnel: w2148 -> [w2159 w2172]
          tunnel: w2150 -> [_ w2166]
          frame False {
            n473 = Get Variant Attribute(Variant=w2165, name=w2164, default value (empty Variant)=w2159, error in=w2163) -> (duplicate Variant=w2160:variant, value=w2161:T32, error out=w2162:errorcluster)  [unwired: 1 out]
            n474 = To Variant(anything=w2161) -> (Variant=w2158:variant)
          }
          frame True {
            n475 = Variant To Data(error in=w2173, type=w2172, Variant=w2166) -> (data=w2171:T32, error out=w2170:errorcluster)
            n476 = Set Variant Attribute(Variant=w2174, name=w2169, value=w2171, error in=w2170) -> (Variant out=w2168:variant, error out=w2167:errorcluster)  [unwired: 1 out]
          }
        }
        n477 = To Variant(anything=w2148) -> (Variant=w2149:variant)
      }
      frame "Phasor Plot:Current Calibration Options" {
        w2175 = T44 {"Phasor Frequency"=0.0, "Phasor Calibration"={"Calibration Lifetime"=1e-09, "Calibration Type"=enum."Single Phasor", "Calibration Map Algorithm"=enum."Simple Search", "Use Backup Calibration if needed"=TRUE, "Backup Calibration Type"=enum."Single Calibration"}} ("AlliGator Phasor Calibration Options")
        n478 = case shown="True" w2178 {
          tunnel: w2184 -> [w2192 w2201]
          tunnel: w2183 -> [w2191 w2196]
          tunnel: w2182 -> [w2190 w2200]
          tunnel: [w2189 w2194] -> w2181
          tunnel: [w2185 w2193] -> w2180
          tunnel: [w2187 w2195] -> w2179
          tunnel: w2175 -> [w2186 w2199]
          tunnel: w2177 -> [_ w2193]
          frame False {
            n479 = Get Variant Attribute(Variant=w2192, name=w2191, default value (empty Variant)=w2186, error in=w2190) -> (duplicate Variant=w2187:variant, value=w2188:T44, error out=w2189:errorcluster)  [unwired: 1 out]
            n480 = To Variant(anything=w2188) -> (Variant=w2185:variant)
          }
          frame True {
            n481 = Variant To Data(error in=w2200, type=w2199, Variant=w2193) -> (data=w2198:T44, error out=w2197:errorcluster)
            n482 = Set Variant Attribute(Variant=w2201, name=w2196, value=w2198, error in=w2197) -> (Variant out=w2195:variant, error out=w2194:errorcluster)  [unwired: 1 out]
          }
        }
        n483 = To Variant(anything=w2175) -> (Variant=w2176:variant)
      }
      frame "Phasor Plot:Reset Cumulated Phasor Plot" {
        w2202 = FALSE
        n484 = case shown="True" w2205 {
          tunnel: w2211 -> [w2219 w2228]
          tunnel: w2210 -> [w2218 w2223]
          tunnel: w2209 -> [w2217 w2227]
          tunnel: [w2216 w2221] -> w2208
          tunnel: [w2212 w2220] -> w2207
          tunnel: [w2214 w2222] -> w2206
          tunnel: w2202 -> [w2213 w2226]
          tunnel: w2204 -> [_ w2220]
          frame False {
            n485 = Get Variant Attribute(Variant=w2219, name=w2218, default value (empty Variant)=w2213, error in=w2217) -> (duplicate Variant=w2214:variant, value=w2215:bool, error out=w2216:errorcluster)  [unwired: 1 out]
            n486 = To Variant(anything=w2215) -> (Variant=w2212:variant)
          }
          frame True {
            n487 = Variant To Data(error in=w2227, type=w2226, Variant=w2220) -> (data=w2225:bool, error out=w2224:errorcluster)
            n488 = Set Variant Attribute(Variant=w2228, name=w2223, value=w2225, error in=w2224) -> (Variant out=w2222:variant, error out=w2221:errorcluster)  [unwired: 1 out]
          }
        }
        n489 = To Variant(anything=w2202) -> (Variant=w2203:variant)
      }
      frame "Phasor Plot:Reference 1" {
        w2229 = T47 {"g"=0.0, "s"=0.0} ("Phasor")
        n490 = case shown="True" w2232 {
          tunnel: w2238 -> [w2246 w2255]
          tunnel: w2237 -> [w2245 w2250]
          tunnel: w2236 -> [w2244 w2254]
          tunnel: [w2243 w2248] -> w2235
          tunnel: [w2239 w2247] -> w2234
          tunnel: [w2241 w2249] -> w2233
          tunnel: w2229 -> [w2240 w2253]
          tunnel: w2231 -> [_ w2247]
          frame False {
            n491 = Get Variant Attribute(Variant=w2246, name=w2245, default value (empty Variant)=w2240, error in=w2244) -> (duplicate Variant=w2241:variant, value=w2242:T47, error out=w2243:errorcluster)  [unwired: 1 out]
            n492 = To Variant(anything=w2242) -> (Variant=w2239:variant)
          }
          frame True {
            n493 = Variant To Data(error in=w2254, type=w2253, Variant=w2247) -> (data=w2252:T47, error out=w2251:errorcluster)
            n494 = Set Variant Attribute(Variant=w2255, name=w2250, value=w2252, error in=w2251) -> (Variant out=w2249:variant, error out=w2248:errorcluster)  [unwired: 1 out]
          }
        }
        n495 = To Variant(anything=w2229) -> (Variant=w2230:variant)
      }
      frame "Phasor Plot:Lifetime Reference 1" {
        w2256 = dbl[unit] nan  # s
        n496 = case shown="True" w2259 {
          tunnel: w2265 -> [w2273 w2282]
          tunnel: w2264 -> [w2272 w2277]
          tunnel: w2263 -> [w2271 w2281]
          tunnel: [w2270 w2275] -> w2262
          tunnel: [w2266 w2274] -> w2261
          tunnel: [w2268 w2276] -> w2260
          tunnel: w2256 -> [w2267 w2280]
          tunnel: w2258 -> [_ w2274]
          frame False {
            n497 = Get Variant Attribute(Variant=w2273, name=w2272, default value (empty Variant)=w2267, error in=w2271) -> (duplicate Variant=w2268:variant, value=w2269:dbl[unit], error out=w2270:errorcluster)  [unwired: 1 out]
            n498 = To Variant(anything=w2269) -> (Variant=w2266:variant)
          }
          frame True {
            n499 = Variant To Data(error in=w2281, type=w2280, Variant=w2274) -> (data=w2279:dbl[unit], error out=w2278:errorcluster)
            n500 = Set Variant Attribute(Variant=w2282, name=w2277, value=w2279, error in=w2278) -> (Variant out=w2276:variant, error out=w2275:errorcluster)  [unwired: 1 out]
          }
        }
        n501 = To Variant(anything=w2256) -> (Variant=w2257:variant)
      }
      frame "Phasor Plot:Reference 1 Frequency" {
        w2283 = dbl[unit] nan  # Hz
        n502 = case shown="True" w2286 {
          tunnel: w2292 -> [w2300 w2309]
          tunnel: w2291 -> [w2299 w2304]
          tunnel: w2290 -> [w2298 w2308]
          tunnel: [w2297 w2302] -> w2289
          tunnel: [w2293 w2301] -> w2288
          tunnel: [w2295 w2303] -> w2287
          tunnel: w2283 -> [w2294 w2307]
          tunnel: w2285 -> [_ w2301]
          frame False {
            n503 = Get Variant Attribute(Variant=w2300, name=w2299, default value (empty Variant)=w2294, error in=w2298) -> (duplicate Variant=w2295:variant, value=w2296:dbl[unit], error out=w2297:errorcluster)  [unwired: 1 out]
            n504 = To Variant(anything=w2296) -> (Variant=w2293:variant)
          }
          frame True {
            n505 = Variant To Data(error in=w2308, type=w2307, Variant=w2301) -> (data=w2306:dbl[unit], error out=w2305:errorcluster)
            n506 = Set Variant Attribute(Variant=w2309, name=w2304, value=w2306, error in=w2305) -> (Variant out=w2303:variant, error out=w2302:errorcluster)  [unwired: 1 out]
          }
        }
        n507 = To Variant(anything=w2283) -> (Variant=w2284:variant)
      }
      frame "Phasor Plot:Reference 2" {
        w2310 = T47 {"g"=0.0, "s"=0.0} ("Phasor")
        n508 = case shown="True" w2313 {
          tunnel: w2319 -> [w2327 w2336]
          tunnel: w2318 -> [w2326 w2331]
          tunnel: w2317 -> [w2325 w2335]
          tunnel: [w2324 w2329] -> w2316
          tunnel: [w2320 w2328] -> w2315
          tunnel: [w2322 w2330] -> w2314
          tunnel: w2310 -> [w2321 w2334]
          tunnel: w2312 -> [_ w2328]
          frame False {
            n509 = Get Variant Attribute(Variant=w2327, name=w2326, default value (empty Variant)=w2321, error in=w2325) -> (duplicate Variant=w2322:variant, value=w2323:T47, error out=w2324:errorcluster)  [unwired: 1 out]
            n510 = To Variant(anything=w2323) -> (Variant=w2320:variant)
          }
          frame True {
            n511 = Variant To Data(error in=w2335, type=w2334, Variant=w2328) -> (data=w2333:T47, error out=w2332:errorcluster)
            n512 = Set Variant Attribute(Variant=w2336, name=w2331, value=w2333, error in=w2332) -> (Variant out=w2330:variant, error out=w2329:errorcluster)  [unwired: 1 out]
          }
        }
        n513 = To Variant(anything=w2310) -> (Variant=w2311:variant)
      }
      frame "Phasor Plot:Lifetime Reference 2" {
        w2337 = dbl[unit] nan  # s
        n514 = case shown="True" w2340 {
          tunnel: w2346 -> [w2354 w2363]
          tunnel: w2345 -> [w2353 w2358]
          tunnel: w2344 -> [w2352 w2362]
          tunnel: [w2351 w2356] -> w2343
          tunnel: [w2347 w2355] -> w2342
          tunnel: [w2349 w2357] -> w2341
          tunnel: w2337 -> [w2348 w2361]
          tunnel: w2339 -> [_ w2355]
          frame False {
            n515 = Get Variant Attribute(Variant=w2354, name=w2353, default value (empty Variant)=w2348, error in=w2352) -> (duplicate Variant=w2349:variant, value=w2350:dbl[unit], error out=w2351:errorcluster)  [unwired: 1 out]
            n516 = To Variant(anything=w2350) -> (Variant=w2347:variant)
          }
          frame True {
            n517 = Variant To Data(error in=w2362, type=w2361, Variant=w2355) -> (data=w2360:dbl[unit], error out=w2359:errorcluster)
            n518 = Set Variant Attribute(Variant=w2363, name=w2358, value=w2360, error in=w2359) -> (Variant out=w2357:variant, error out=w2356:errorcluster)  [unwired: 1 out]
          }
        }
        n519 = To Variant(anything=w2337) -> (Variant=w2338:variant)
      }
      frame "Phasor Plot:Reference 2 Frequency" {
        w2364 = dbl[unit] nan  # Hz
        n520 = case shown="True" w2367 {
          tunnel: w2373 -> [w2381 w2390]
          tunnel: w2372 -> [w2380 w2385]
          tunnel: w2371 -> [w2379 w2389]
          tunnel: [w2378 w2383] -> w2370
          tunnel: [w2374 w2382] -> w2369
          tunnel: [w2376 w2384] -> w2368
          tunnel: w2364 -> [w2375 w2388]
          tunnel: w2366 -> [_ w2382]
          frame False {
            n521 = Get Variant Attribute(Variant=w2381, name=w2380, default value (empty Variant)=w2375, error in=w2379) -> (duplicate Variant=w2376:variant, value=w2377:dbl[unit], error out=w2378:errorcluster)  [unwired: 1 out]
            n522 = To Variant(anything=w2377) -> (Variant=w2374:variant)
          }
          frame True {
            n523 = Variant To Data(error in=w2389, type=w2388, Variant=w2382) -> (data=w2387:dbl[unit], error out=w2386:errorcluster)
            n524 = Set Variant Attribute(Variant=w2390, name=w2385, value=w2387, error in=w2386) -> (Variant out=w2384:variant, error out=w2383:errorcluster)  [unwired: 1 out]
          }
        }
        n525 = To Variant(anything=w2364) -> (Variant=w2365:variant)
      }
      frame "---- Decay Analysis ----" {
      }
      frame "Number of Selected Decays to Fit" {
        w2394 = 0
        n526 = case shown="True" w2397 {
          tunnel: w2403 -> [w2411 w2420]
          tunnel: w2402 -> [w2410 w2415]
          tunnel: w2401 -> [w2409 w2419]
          tunnel: [w2408 w2413] -> w2400
          tunnel: [w2404 w2412] -> w2399
          tunnel: [w2406 w2414] -> w2398
          tunnel: w2394 -> [w2405 w2418]
          tunnel: w2396 -> [_ w2412]
          frame False {
            n527 = Get Variant Attribute(Variant=w2411, name=w2410, default value (empty Variant)=w2405, error in=w2409) -> (duplicate Variant=w2406:variant, value=w2407:i32, error out=w2408:errorcluster)  [unwired: 1 out]
            n528 = To Variant(anything=w2407) -> (Variant=w2404:variant)
          }
          frame True {
            n529 = Variant To Data(error in=w2419, type=w2418, Variant=w2412) -> (data=w2417:i32, error out=w2416:errorcluster)
            n530 = Set Variant Attribute(Variant=w2420, name=w2415, value=w2417, error in=w2416) -> (Variant out=w2414:variant, error out=w2413:errorcluster)  [unwired: 1 out]
          }
        }
        n531 = To Variant(anything=w2394) -> (Variant=w2395:variant)
      }
      frame "LS Fit Results" {
        w2421 = T48 {"Chi2/DOF"=0.0, "R2"=0.0, "RMSE"=0.0, "Fitting Method"=enum."Least Square", "Fitting Algorithm"=enum."Levenberg-Marquardt"} ("Fit Statistics")
        n532 = case shown="True" w2424 {
          tunnel: w2430 -> [w2438 w2447]
          tunnel: w2429 -> [w2437 w2442]
          tunnel: w2428 -> [w2436 w2446]
          tunnel: [w2435 w2440] -> w2427
          tunnel: [w2431 w2439] -> w2426
          tunnel: [w2433 w2441] -> w2425
          tunnel: w2421 -> [w2432 w2445]
          tunnel: w2423 -> [_ w2439]
          frame False {
            n533 = Get Variant Attribute(Variant=w2438, name=w2437, default value (empty Variant)=w2432, error in=w2436) -> (duplicate Variant=w2433:variant, value=w2434:T48, error out=w2435:errorcluster)  [unwired: 1 out]
            n534 = To Variant(anything=w2434) -> (Variant=w2431:variant)
          }
          frame True {
            n535 = Variant To Data(error in=w2446, type=w2445, Variant=w2439) -> (data=w2444:T48, error out=w2443:errorcluster)
            n536 = Set Variant Attribute(Variant=w2447, name=w2442, value=w2444, error in=w2443) -> (Variant out=w2441:variant, error out=w2440:errorcluster)  [unwired: 1 out]
          }
        }
        n537 = To Variant(anything=w2421) -> (Variant=w2422:variant)
      }
      frame "LAR Fit Results" {
        w2448 = T48 {"Chi2/DOF"=0.0, "R2"=0.0, "RMSE"=0.0, "Fitting Method"=enum."Least Square", "Fitting Algorithm"=enum."Levenberg-Marquardt"} ("Fit Statistics")
        n538 = case shown="True" w2451 {
          tunnel: w2457 -> [w2465 w2474]
          tunnel: w2456 -> [w2464 w2469]
          tunnel: w2455 -> [w2463 w2473]
          tunnel: [w2462 w2467] -> w2454
          tunnel: [w2458 w2466] -> w2453
          tunnel: [w2460 w2468] -> w2452
          tunnel: w2448 -> [w2459 w2472]
          tunnel: w2450 -> [_ w2466]
          frame False {
            n539 = Get Variant Attribute(Variant=w2465, name=w2464, default value (empty Variant)=w2459, error in=w2463) -> (duplicate Variant=w2460:variant, value=w2461:T48, error out=w2462:errorcluster)  [unwired: 1 out]
            n540 = To Variant(anything=w2461) -> (Variant=w2458:variant)
          }
          frame True {
            n541 = Variant To Data(error in=w2473, type=w2472, Variant=w2466) -> (data=w2471:T48, error out=w2470:errorcluster)
            n542 = Set Variant Attribute(Variant=w2474, name=w2469, value=w2471, error in=w2470) -> (Variant out=w2468:variant, error out=w2467:errorcluster)  [unwired: 1 out]
          }
        }
        n543 = To Variant(anything=w2448) -> (Variant=w2449:variant)
      }
      frame "BS Fit Results" {
        w2475 = T48 {"Chi2/DOF"=0.0, "R2"=0.0, "RMSE"=0.0, "Fitting Method"=enum."Least Square", "Fitting Algorithm"=enum."Levenberg-Marquardt"} ("Fit Statistics")
        n544 = case shown="True" w2478 {
          tunnel: w2484 -> [w2492 w2501]
          tunnel: w2483 -> [w2491 w2496]
          tunnel: w2482 -> [w2490 w2500]
          tunnel: [w2489 w2494] -> w2481
          tunnel: [w2485 w2493] -> w2480
          tunnel: [w2487 w2495] -> w2479
          tunnel: w2475 -> [w2486 w2499]
          tunnel: w2477 -> [_ w2493]
          frame False {
            n545 = Get Variant Attribute(Variant=w2492, name=w2491, default value (empty Variant)=w2486, error in=w2490) -> (duplicate Variant=w2487:variant, value=w2488:T48, error out=w2489:errorcluster)  [unwired: 1 out]
            n546 = To Variant(anything=w2488) -> (Variant=w2485:variant)
          }
          frame True {
            n547 = Variant To Data(error in=w2500, type=w2499, Variant=w2493) -> (data=w2498:T48, error out=w2497:errorcluster)
            n548 = Set Variant Attribute(Variant=w2501, name=w2496, value=w2498, error in=w2497) -> (Variant out=w2495:variant, error out=w2494:errorcluster)  [unwired: 1 out]
          }
        }
        n549 = To Variant(anything=w2475) -> (Variant=w2476:variant)
      }
      frame "Last Decay Max - Min" {
        w2502 = 0.0 ("Fit Statistics")
        n550 = case shown="True" w2505 {
          tunnel: w2511 -> [w2519 w2528]
          tunnel: w2510 -> [w2518 w2523]
          tunnel: w2509 -> [w2517 w2527]
          tunnel: [w2516 w2521] -> w2508
          tunnel: [w2512 w2520] -> w2507
          tunnel: [w2514 w2522] -> w2506
          tunnel: w2502 -> [w2513 w2526]
          tunnel: w2504 -> [_ w2520]
          frame False {
            n551 = Get Variant Attribute(Variant=w2519, name=w2518, default value (empty Variant)=w2513, error in=w2517) -> (duplicate Variant=w2514:variant, value=w2515:dbl, error out=w2516:errorcluster)  [unwired: 1 out]
            n552 = To Variant(anything=w2515) -> (Variant=w2512:variant)
          }
          frame True {
            n553 = Variant To Data(error in=w2527, type=w2526, Variant=w2520) -> (data=w2525:dbl, error out=w2524:errorcluster)
            n554 = Set Variant Attribute(Variant=w2528, name=w2523, value=w2525, error in=w2524) -> (Variant out=w2522:variant, error out=w2521:errorcluster)  [unwired: 1 out]
          }
        }
        n555 = To Variant(anything=w2502) -> (Variant=w2503:variant)
      }
      frame "Best Fit Parameters" {
        w2529 = dbl[] []
        n556 = case shown="True" w2532 {
          tunnel: w2538 -> [w2546 w2555]
          tunnel: w2537 -> [w2545 w2550]
          tunnel: w2536 -> [w2544 w2554]
          tunnel: [w2543 w2548] -> w2535
          tunnel: [w2539 w2547] -> w2534
          tunnel: [w2541 w2549] -> w2533
          tunnel: w2529 -> [w2540 w2553]
          tunnel: w2531 -> [_ w2547]
          frame False {
            n557 = Get Variant Attribute(Variant=w2546, name=w2545, default value (empty Variant)=w2540, error in=w2544) -> (duplicate Variant=w2541:variant, value=w2542:dbl[], error out=w2543:errorcluster)  [unwired: 1 out]
            n558 = To Variant(anything=w2542) -> (Variant=w2539:variant)
          }
          frame True {
            n559 = Variant To Data(error in=w2554, type=w2553, Variant=w2547) -> (data=w2552:dbl[], error out=w2551:errorcluster)
            n560 = Set Variant Attribute(Variant=w2555, name=w2550, value=w2552, error in=w2551) -> (Variant out=w2549:variant, error out=w2548:errorcluster)  [unwired: 1 out]
          }
        }
        n561 = To Variant(anything=w2529) -> (Variant=w2530:variant)
      }
      frame "Best Fit Parameter Names" {
        w2556 = T51[] [] items=["Offset", "Baseline", "A_1", "tau_1", "A_2", "tau_2"] ("Array")
        n562 = case shown="True" w2559 {
          tunnel: w2565 -> [w2573 w2582]
          tunnel: w2564 -> [w2572 w2577]
          tunnel: w2563 -> [w2571 w2581]
          tunnel: [w2570 w2575] -> w2562
          tunnel: [w2566 w2574] -> w2561
          tunnel: [w2568 w2576] -> w2560
          tunnel: w2556 -> [w2567 w2580]
          tunnel: w2558 -> [_ w2574]
          frame False {
            n563 = Get Variant Attribute(Variant=w2573, name=w2572, default value (empty Variant)=w2567, error in=w2571) -> (duplicate Variant=w2568:variant, value=w2569:T51[], error out=w2570:errorcluster)  [unwired: 1 out]
            n564 = To Variant(anything=w2569) -> (Variant=w2566:variant)
          }
          frame True {
            n565 = Variant To Data(error in=w2581, type=w2580, Variant=w2574) -> (data=w2579:T51[], error out=w2578:errorcluster)
            n566 = Set Variant Attribute(Variant=w2582, name=w2577, value=w2579, error in=w2578) -> (Variant out=w2576:variant, error out=w2575:errorcluster)  [unwired: 1 out]
          }
        }
        n567 = To Variant(anything=w2556) -> (Variant=w2557:variant)
      }
      frame "Actual Size X" {
        w2583 = 0
        n568 = case shown="True" w2586 {
          tunnel: w2592 -> [w2600 w2609]
          tunnel: w2591 -> [w2599 w2604]
          tunnel: w2590 -> [w2598 w2608]
          tunnel: [w2597 w2602] -> w2589
          tunnel: [w2593 w2601] -> w2588
          tunnel: [w2595 w2603] -> w2587
          tunnel: w2583 -> [w2594 w2607]
          tunnel: w2585 -> [_ w2601]
          frame False {
            n569 = Get Variant Attribute(Variant=w2600, name=w2599, default value (empty Variant)=w2594, error in=w2598) -> (duplicate Variant=w2595:variant, value=w2596:i32, error out=w2597:errorcluster)  [unwired: 1 out]
            n570 = To Variant(anything=w2596) -> (Variant=w2593:variant)
          }
          frame True {
            n571 = Variant To Data(error in=w2608, type=w2607, Variant=w2601) -> (data=w2606:i32, error out=w2605:errorcluster)
            n572 = Set Variant Attribute(Variant=w2609, name=w2604, value=w2606, error in=w2605) -> (Variant out=w2603:variant, error out=w2602:errorcluster)  [unwired: 1 out]
          }
        }
        n573 = To Variant(anything=w2583) -> (Variant=w2584:variant)
      }
      frame "Actual Size Y" {
        w2610 = 0
        n574 = case shown="True" w2613 {
          tunnel: w2619 -> [w2627 w2636]
          tunnel: w2618 -> [w2626 w2631]
          tunnel: w2617 -> [w2625 w2635]
          tunnel: [w2624 w2629] -> w2616
          tunnel: [w2620 w2628] -> w2615
          tunnel: [w2622 w2630] -> w2614
          tunnel: w2610 -> [w2621 w2634]
          tunnel: w2612 -> [_ w2628]
          frame False {
            n575 = Get Variant Attribute(Variant=w2627, name=w2626, default value (empty Variant)=w2621, error in=w2625) -> (duplicate Variant=w2622:variant, value=w2623:i32, error out=w2624:errorcluster)  [unwired: 1 out]
            n576 = To Variant(anything=w2623) -> (Variant=w2620:variant)
          }
          frame True {
            n577 = Variant To Data(error in=w2635, type=w2634, Variant=w2628) -> (data=w2633:i32, error out=w2632:errorcluster)
            n578 = Set Variant Attribute(Variant=w2636, name=w2631, value=w2633, error in=w2632) -> (Variant out=w2630:variant, error out=w2629:errorcluster)  [unwired: 1 out]
          }
        }
        n579 = To Variant(anything=w2610) -> (Variant=w2611:variant)
      }
      frame "Binning X" {
        w2637 = 0
        n580 = case shown="True" w2640 {
          tunnel: w2646 -> [w2654 w2663]
          tunnel: w2645 -> [w2653 w2658]
          tunnel: w2644 -> [w2652 w2662]
          tunnel: [w2651 w2656] -> w2643
          tunnel: [w2647 w2655] -> w2642
          tunnel: [w2649 w2657] -> w2641
          tunnel: w2637 -> [w2648 w2661]
          tunnel: w2639 -> [_ w2655]
          frame False {
            n581 = Get Variant Attribute(Variant=w2654, name=w2653, default value (empty Variant)=w2648, error in=w2652) -> (duplicate Variant=w2649:variant, value=w2650:i32, error out=w2651:errorcluster)  [unwired: 1 out]
            n582 = To Variant(anything=w2650) -> (Variant=w2647:variant)
          }
          frame True {
            n583 = Variant To Data(error in=w2662, type=w2661, Variant=w2655) -> (data=w2660:i32, error out=w2659:errorcluster)
            n584 = Set Variant Attribute(Variant=w2663, name=w2658, value=w2660, error in=w2659) -> (Variant out=w2657:variant, error out=w2656:errorcluster)  [unwired: 1 out]
          }
        }
        n585 = To Variant(anything=w2637) -> (Variant=w2638:variant)
      }
      frame "Binning Y" {
        w2664 = 0
        n586 = case shown="True" w2667 {
          tunnel: w2673 -> [w2681 w2690]
          tunnel: w2672 -> [w2680 w2685]
          tunnel: w2671 -> [w2679 w2689]
          tunnel: [w2678 w2683] -> w2670
          tunnel: [w2674 w2682] -> w2669
          tunnel: [w2676 w2684] -> w2668
          tunnel: w2664 -> [w2675 w2688]
          tunnel: w2666 -> [_ w2682]
          frame False {
            n587 = Get Variant Attribute(Variant=w2681, name=w2680, default value (empty Variant)=w2675, error in=w2679) -> (duplicate Variant=w2676:variant, value=w2677:i32, error out=w2678:errorcluster)  [unwired: 1 out]
            n588 = To Variant(anything=w2677) -> (Variant=w2674:variant)
          }
          frame True {
            n589 = Variant To Data(error in=w2689, type=w2688, Variant=w2682) -> (data=w2687:i32, error out=w2686:errorcluster)
            n590 = Set Variant Attribute(Variant=w2690, name=w2685, value=w2687, error in=w2686) -> (Variant out=w2684:variant, error out=w2683:errorcluster)  [unwired: 1 out]
          }
        }
        n591 = To Variant(anything=w2664) -> (Variant=w2665:variant)
      }
      frame "Actual # Gates" {
        w2691 = 0
        n592 = case shown="True" w2694 {
          tunnel: w2700 -> [w2708 w2717]
          tunnel: w2699 -> [w2707 w2712]
          tunnel: w2698 -> [w2706 w2716]
          tunnel: [w2705 w2710] -> w2697
          tunnel: [w2701 w2709] -> w2696
          tunnel: [w2703 w2711] -> w2695
          tunnel: w2691 -> [w2702 w2715]
          tunnel: w2693 -> [_ w2709]
          frame False {
            n593 = Get Variant Attribute(Variant=w2708, name=w2707, default value (empty Variant)=w2702, error in=w2706) -> (duplicate Variant=w2703:variant, value=w2704:i32, error out=w2705:errorcluster)  [unwired: 1 out]
            n594 = To Variant(anything=w2704) -> (Variant=w2701:variant)
          }
          frame True {
            n595 = Variant To Data(error in=w2716, type=w2715, Variant=w2709) -> (data=w2714:i32, error out=w2713:errorcluster)
            n596 = Set Variant Attribute(Variant=w2717, name=w2712, value=w2714, error in=w2713) -> (Variant out=w2711:variant, error out=w2710:errorcluster)  [unwired: 1 out]
          }
        }
        n597 = To Variant(anything=w2691) -> (Variant=w2692:variant)
      }
      frame "Dataset Number" {
        w2718 = 0
        n598 = case shown="True" w2721 {
          tunnel: w2727 -> [w2735 w2744]
          tunnel: w2726 -> [w2734 w2739]
          tunnel: w2725 -> [w2733 w2743]
          tunnel: [w2732 w2737] -> w2724
          tunnel: [w2728 w2736] -> w2723
          tunnel: [w2730 w2738] -> w2722
          tunnel: w2718 -> [w2729 w2742]
          tunnel: w2720 -> [_ w2736]
          frame False {
            n599 = Get Variant Attribute(Variant=w2735, name=w2734, default value (empty Variant)=w2729, error in=w2733) -> (duplicate Variant=w2730:variant, value=w2731:i32, error out=w2732:errorcluster)  [unwired: 1 out]
            n600 = To Variant(anything=w2731) -> (Variant=w2728:variant)
          }
          frame True {
            n601 = Variant To Data(error in=w2743, type=w2742, Variant=w2736) -> (data=w2741:i32, error out=w2740:errorcluster)
            n602 = Set Variant Attribute(Variant=w2744, name=w2739, value=w2741, error in=w2740) -> (Variant out=w2738:variant, error out=w2737:errorcluster)  [unwired: 1 out]
          }
        }
        n603 = To Variant(anything=w2718) -> (Variant=w2719:variant)
      }
      frame "Gates to..." {
        w2745 = TRUE
        n604 = case shown="True" w2748 {
          tunnel: w2754 -> [w2762 w2771]
          tunnel: w2753 -> [w2761 w2766]
          tunnel: w2752 -> [w2760 w2770]
          tunnel: [w2759 w2764] -> w2751
          tunnel: [w2755 w2763] -> w2750
          tunnel: [w2757 w2765] -> w2749
          tunnel: w2745 -> [w2756 w2769]
          tunnel: w2747 -> [_ w2763]
          frame False {
            n605 = Get Variant Attribute(Variant=w2762, name=w2761, default value (empty Variant)=w2756, error in=w2760) -> (duplicate Variant=w2757:variant, value=w2758:bool, error out=w2759:errorcluster)  [unwired: 1 out]
            n606 = To Variant(anything=w2758) -> (Variant=w2755:variant)
          }
          frame True {
            n607 = Variant To Data(error in=w2770, type=w2769, Variant=w2763) -> (data=w2768:bool, error out=w2767:errorcluster)
            n608 = Set Variant Attribute(Variant=w2771, name=w2766, value=w2768, error in=w2767) -> (Variant out=w2765:variant, error out=w2764:errorcluster)  [unwired: 1 out]
          }
        }
        n609 = To Variant(anything=w2745) -> (Variant=w2746:variant)
      }
      frame "Gates Skipped" {
        w2772 = T9 {"Start"=0, "End"=0} ("Gates to Skip")
        n610 = case shown="True" w2775 {
          tunnel: w2781 -> [w2789 w2798]
          tunnel: w2780 -> [w2788 w2793]
          tunnel: w2779 -> [w2787 w2797]
          tunnel: [w2786 w2791] -> w2778
          tunnel: [w2782 w2790] -> w2777
          tunnel: [w2784 w2792] -> w2776
          tunnel: w2772 -> [w2783 w2796]
          tunnel: w2774 -> [_ w2790]
          frame False {
            n611 = Get Variant Attribute(Variant=w2789, name=w2788, default value (empty Variant)=w2783, error in=w2787) -> (duplicate Variant=w2784:variant, value=w2785:T9, error out=w2786:errorcluster)  [unwired: 1 out]
            n612 = To Variant(anything=w2785) -> (Variant=w2782:variant)
          }
          frame True {
            n613 = Variant To Data(error in=w2797, type=w2796, Variant=w2790) -> (data=w2795:T9, error out=w2794:errorcluster)
            n614 = Set Variant Attribute(Variant=w2798, name=w2793, value=w2795, error in=w2794) -> (Variant out=w2792:variant, error out=w2791:errorcluster)  [unwired: 1 out]
          }
        }
        n615 = To Variant(anything=w2772) -> (Variant=w2773:variant)
      }
      frame "Gates to keep" {
        w2799 = T9 {"Start"=0, "End"=0} ("Gates to Skip")
        n616 = case shown="True" w2802 {
          tunnel: w2808 -> [w2816 w2825]
          tunnel: w2807 -> [w2815 w2820]
          tunnel: w2806 -> [w2814 w2824]
          tunnel: [w2813 w2818] -> w2805
          tunnel: [w2809 w2817] -> w2804
          tunnel: [w2811 w2819] -> w2803
          tunnel: w2799 -> [w2810 w2823]
          tunnel: w2801 -> [_ w2817]
          frame False {
            n617 = Get Variant Attribute(Variant=w2816, name=w2815, default value (empty Variant)=w2810, error in=w2814) -> (duplicate Variant=w2811:variant, value=w2812:T9, error out=w2813:errorcluster)  [unwired: 1 out]
            n618 = To Variant(anything=w2812) -> (Variant=w2809:variant)
          }
          frame True {
            n619 = Variant To Data(error in=w2824, type=w2823, Variant=w2817) -> (data=w2822:T9, error out=w2821:errorcluster)
            n620 = Set Variant Attribute(Variant=w2825, name=w2820, value=w2822, error in=w2821) -> (Variant out=w2819:variant, error out=w2818:errorcluster)  [unwired: 1 out]
          }
        }
        n621 = To Variant(anything=w2799) -> (Variant=w2800:variant)
      }
      frame "Gate Step" {
        w2826 = 0
        n622 = case shown="True" w2829 {
          tunnel: w2835 -> [w2843 w2852]
          tunnel: w2834 -> [w2842 w2847]
          tunnel: w2833 -> [w2841 w2851]
          tunnel: [w2840 w2845] -> w2832
          tunnel: [w2836 w2844] -> w2831
          tunnel: [w2838 w2846] -> w2830
          tunnel: w2826 -> [w2837 w2850]
          tunnel: w2828 -> [_ w2844]
          frame False {
            n623 = Get Variant Attribute(Variant=w2843, name=w2842, default value (empty Variant)=w2837, error in=w2841) -> (duplicate Variant=w2838:variant, value=w2839:i32, error out=w2840:errorcluster)  [unwired: 1 out]
            n624 = To Variant(anything=w2839) -> (Variant=w2836:variant)
          }
          frame True {
            n625 = Variant To Data(error in=w2851, type=w2850, Variant=w2844) -> (data=w2849:i32, error out=w2848:errorcluster)
            n626 = Set Variant Attribute(Variant=w2852, name=w2847, value=w2849, error in=w2848) -> (Variant out=w2846:variant, error out=w2845:errorcluster)  [unwired: 1 out]
          }
        }
        n627 = To Variant(anything=w2826) -> (Variant=w2827:variant)
      }
      frame "Gate Separation" {
        w2853 = 0.0  # s
        n628 = case shown="True" w2856 {
          tunnel: w2862 -> [w2870 w2879]
          tunnel: w2861 -> [w2869 w2874]
          tunnel: w2860 -> [w2868 w2878]
          tunnel: [w2867 w2872] -> w2859
          tunnel: [w2863 w2871] -> w2858
          tunnel: [w2865 w2873] -> w2857
          tunnel: w2853 -> [w2864 w2877]
          tunnel: w2855 -> [_ w2871]
          frame False {
            n629 = Get Variant Attribute(Variant=w2870, name=w2869, default value (empty Variant)=w2864, error in=w2868) -> (duplicate Variant=w2865:variant, value=w2866:dbl, error out=w2867:errorcluster)  [unwired: 1 out]
            n630 = To Variant(anything=w2866) -> (Variant=w2863:variant)
          }
          frame True {
            n631 = Variant To Data(error in=w2878, type=w2877, Variant=w2871) -> (data=w2876:dbl, error out=w2875:errorcluster)
            n632 = Set Variant Attribute(Variant=w2879, name=w2874, value=w2876, error in=w2875) -> (Variant out=w2873:variant, error out=w2872:errorcluster)  [unwired: 1 out]
          }
        }
        n633 = To Variant(anything=w2853) -> (Variant=w2854:variant)
      }
      frame "Reversed Gates" {
        w2880 = FALSE
        n634 = case shown="True" w2883 {
          tunnel: w2889 -> [w2897 w2906]
          tunnel: w2888 -> [w2896 w2901]
          tunnel: w2887 -> [w2895 w2905]
          tunnel: [w2894 w2899] -> w2886
          tunnel: [w2890 w2898] -> w2885
          tunnel: [w2892 w2900] -> w2884
          tunnel: w2880 -> [w2891 w2904]
          tunnel: w2882 -> [_ w2898]
          frame False {
            n635 = Get Variant Attribute(Variant=w2897, name=w2896, default value (empty Variant)=w2891, error in=w2895) -> (duplicate Variant=w2892:variant, value=w2893:bool, error out=w2894:errorcluster)  [unwired: 1 out]
            n636 = To Variant(anything=w2893) -> (Variant=w2890:variant)
          }
          frame True {
            n637 = Variant To Data(error in=w2905, type=w2904, Variant=w2898) -> (data=w2903:bool, error out=w2902:errorcluster)
            n638 = Set Variant Attribute(Variant=w2906, name=w2901, value=w2903, error in=w2902) -> (Variant out=w2900:variant, error out=w2899:errorcluster)  [unwired: 1 out]
          }
        }
        n639 = To Variant(anything=w2880) -> (Variant=w2881:variant)
      }
      frame "Pile-up Correction" {
        w2907 = FALSE
        n640 = case shown="True" w2910 {
          tunnel: w2916 -> [w2924 w2933]
          tunnel: w2915 -> [w2923 w2928]
          tunnel: w2914 -> [w2922 w2932]
          tunnel: [w2921 w2926] -> w2913
          tunnel: [w2917 w2925] -> w2912
          tunnel: [w2919 w2927] -> w2911
          tunnel: w2907 -> [w2918 w2931]
          tunnel: w2909 -> [_ w2925]
          frame False {
            n641 = Get Variant Attribute(Variant=w2924, name=w2923, default value (empty Variant)=w2918, error in=w2922) -> (duplicate Variant=w2919:variant, value=w2920:bool, error out=w2921:errorcluster)  [unwired: 1 out]
            n642 = To Variant(anything=w2920) -> (Variant=w2917:variant)
          }
          frame True {
            n643 = Variant To Data(error in=w2932, type=w2931, Variant=w2925) -> (data=w2930:bool, error out=w2929:errorcluster)
            n644 = Set Variant Attribute(Variant=w2933, name=w2928, value=w2930, error in=w2929) -> (Variant out=w2927:variant, error out=w2926:errorcluster)  [unwired: 1 out]
          }
        }
        n645 = To Variant(anything=w2907) -> (Variant=w2908:variant)
      }
      frame "Pixel Well Capacity" {
        w2934 = u32 0  # U32
        n646 = case shown="True" w2937 {
          tunnel: w2943 -> [w2951 w2960]
          tunnel: w2942 -> [w2950 w2955]
          tunnel: w2941 -> [w2949 w2959]
          tunnel: [w2948 w2953] -> w2940
          tunnel: [w2944 w2952] -> w2939
          tunnel: [w2946 w2954] -> w2938
          tunnel: w2934 -> [w2945 w2958]
          tunnel: w2936 -> [_ w2952]
          frame False {
            n647 = Get Variant Attribute(Variant=w2951, name=w2950, default value (empty Variant)=w2945, error in=w2949) -> (duplicate Variant=w2946:variant, value=w2947:u32, error out=w2948:errorcluster)  [unwired: 1 out]
            n648 = To Variant(anything=w2947) -> (Variant=w2944:variant)
          }
          frame True {
            n649 = Variant To Data(error in=w2959, type=w2958, Variant=w2952) -> (data=w2957:u32, error out=w2956:errorcluster)
            n650 = Set Variant Attribute(Variant=w2960, name=w2955, value=w2957, error in=w2956) -> (Variant out=w2954:variant, error out=w2953:errorcluster)  [unwired: 1 out]
          }
        }
        n651 = To Variant(anything=w2934) -> (Variant=w2935:variant)
      }
      frame "Background Subtracted" {
        w2961 = FALSE
        n652 = case shown="True" w2964 {
          tunnel: w2970 -> [w2978 w2987]
          tunnel: w2969 -> [w2977 w2982]
          tunnel: w2968 -> [w2976 w2986]
          tunnel: [w2975 w2980] -> w2967
          tunnel: [w2971 w2979] -> w2966
          tunnel: [w2973 w2981] -> w2965
          tunnel: w2961 -> [w2972 w2985]
          tunnel: w2963 -> [_ w2979]
          frame False {
            n653 = Get Variant Attribute(Variant=w2978, name=w2977, default value (empty Variant)=w2972, error in=w2976) -> (duplicate Variant=w2973:variant, value=w2974:bool, error out=w2975:errorcluster)  [unwired: 1 out]
            n654 = To Variant(anything=w2974) -> (Variant=w2971:variant)
          }
          frame True {
            n655 = Variant To Data(error in=w2986, type=w2985, Variant=w2979) -> (data=w2984:bool, error out=w2983:errorcluster)
            n656 = Set Variant Attribute(Variant=w2987, name=w2982, value=w2984, error in=w2983) -> (Variant out=w2981:variant, error out=w2980:errorcluster)  [unwired: 1 out]
          }
        }
        n657 = To Variant(anything=w2961) -> (Variant=w2962:variant)
      }
      frame "Background Subtraction Method" {
        w2988 = AlliGator_Baseline_Subtraction_Method."Constant" ("Baseline Subtraction Method")
        n658 = case shown="True" w2991 {
          tunnel: w2997 -> [w3005 w3014]
          tunnel: w2996 -> [w3004 w3009]
          tunnel: w2995 -> [w3003 w3013]
          tunnel: [w3002 w3007] -> w2994
          tunnel: [w2998 w3006] -> w2993
          tunnel: [w3000 w3008] -> w2992
          tunnel: w2988 -> [w2999 w3012]
          tunnel: w2990 -> [_ w3006]
          frame False {
            n659 = Get Variant Attribute(Variant=w3005, name=w3004, default value (empty Variant)=w2999, error in=w3003) -> (duplicate Variant=w3000:variant, value=w3001:T35, error out=w3002:errorcluster)  [unwired: 1 out]
            n660 = To Variant(anything=w3001) -> (Variant=w2998:variant)
          }
          frame True {
            n661 = Variant To Data(error in=w3013, type=w3012, Variant=w3006) -> (data=w3011:T35, error out=w3010:errorcluster)
            n662 = Set Variant Attribute(Variant=w3014, name=w3009, value=w3011, error in=w3010) -> (Variant out=w3008:variant, error out=w3007:errorcluster)  [unwired: 1 out]
          }
        }
        n663 = To Variant(anything=w2988) -> (Variant=w2989:variant)
      }
      frame "Background Definition Range" {
        w3015 = T52 {"Min Gate"=0.0, "Max Gate"=0.0} ("Background Definition Range")
        n664 = case shown="True" w3018 {
          tunnel: w3024 -> [w3032 w3041]
          tunnel: w3023 -> [w3031 w3036]
          tunnel: w3022 -> [w3030 w3040]
          tunnel: [w3029 w3034] -> w3021
          tunnel: [w3025 w3033] -> w3020
          tunnel: [w3027 w3035] -> w3019
          tunnel: w3015 -> [w3026 w3039]
          tunnel: w3017 -> [_ w3033]
          frame False {
            n665 = Get Variant Attribute(Variant=w3032, name=w3031, default value (empty Variant)=w3026, error in=w3030) -> (duplicate Variant=w3027:variant, value=w3028:T52, error out=w3029:errorcluster)  [unwired: 1 out]
            n666 = To Variant(anything=w3028) -> (Variant=w3025:variant)
          }
          frame True {
            n667 = Variant To Data(error in=w3040, type=w3039, Variant=w3033) -> (data=w3038:T52, error out=w3037:errorcluster)
            n668 = Set Variant Attribute(Variant=w3041, name=w3036, value=w3038, error in=w3037) -> (Variant out=w3035:variant, error out=w3034:errorcluster)  [unwired: 1 out]
          }
        }
        n669 = To Variant(anything=w3015) -> (Variant=w3016:variant)
      }
      frame "Background File (deprecated)" {
        w3042 = path "" ("Background Definition Range")
        n670 = case shown="True" w3045 {
          tunnel: w3051 -> [w3059 w3068]
          tunnel: w3050 -> [w3058 w3063]
          tunnel: w3049 -> [w3057 w3067]
          tunnel: [w3056 w3061] -> w3048
          tunnel: [w3052 w3060] -> w3047
          tunnel: [w3054 w3062] -> w3046
          tunnel: w3042 -> [w3053 w3066]
          tunnel: w3044 -> [_ w3060]
          frame False {
            n671 = Get Variant Attribute(Variant=w3059, name=w3058, default value (empty Variant)=w3053, error in=w3057) -> (duplicate Variant=w3054:variant, value=w3055:path, error out=w3056:errorcluster)  [unwired: 1 out]
            n672 = To Variant(anything=w3055) -> (Variant=w3052:variant)
          }
          frame True {
            n673 = Variant To Data(error in=w3067, type=w3066, Variant=w3060) -> (data=w3065:path, error out=w3064:errorcluster)
            n674 = Set Variant Attribute(Variant=w3068, name=w3063, value=w3065, error in=w3064) -> (Variant out=w3062:variant, error out=w3061:errorcluster)  [unwired: 1 out]
          }
        }
        n675 = To Variant(anything=w3042) -> (Variant=w3043:variant)
      }
      frame "Number of Dataset Accumulated" {
        w3069 = 0
        n676 = case shown="True" w3072 {
          tunnel: w3078 -> [w3086 w3095]
          tunnel: w3077 -> [w3085 w3090]
          tunnel: w3076 -> [w3084 w3094]
          tunnel: [w3083 w3088] -> w3075
          tunnel: [w3079 w3087] -> w3074
          tunnel: [w3081 w3089] -> w3073
          tunnel: w3069 -> [w3080 w3093]
          tunnel: w3071 -> [_ w3087]
          frame False {
            n677 = Get Variant Attribute(Variant=w3086, name=w3085, default value (empty Variant)=w3080, error in=w3084) -> (duplicate Variant=w3081:variant, value=w3082:i32, error out=w3083:errorcluster)  [unwired: 1 out]
            n678 = To Variant(anything=w3082) -> (Variant=w3079:variant)
          }
          frame True {
            n679 = Variant To Data(error in=w3094, type=w3093, Variant=w3087) -> (data=w3092:i32, error out=w3091:errorcluster)
            n680 = Set Variant Attribute(Variant=w3095, name=w3090, value=w3092, error in=w3091) -> (Variant out=w3089:variant, error out=w3088:errorcluster)  [unwired: 1 out]
          }
        }
        n681 = To Variant(anything=w3069) -> (Variant=w3070:variant)
      }
      frame "Array of Accumulated Dataset Paths" {
        w3096 = path[] [] ("Background Definition Range")
        n682 = case shown="True" w3099 {
          tunnel: w3105 -> [w3113 w3122]
          tunnel: w3104 -> [w3112 w3117]
          tunnel: w3103 -> [w3111 w3121]
          tunnel: [w3110 w3115] -> w3102
          tunnel: [w3106 w3114] -> w3101
          tunnel: [w3108 w3116] -> w3100
          tunnel: w3096 -> [w3107 w3120]
          tunnel: w3098 -> [_ w3114]
          frame False {
            n683 = Get Variant Attribute(Variant=w3113, name=w3112, default value (empty Variant)=w3107, error in=w3111) -> (duplicate Variant=w3108:variant, value=w3109:path[], error out=w3110:errorcluster)  [unwired: 1 out]
            n684 = To Variant(anything=w3109) -> (Variant=w3106:variant)
          }
          frame True {
            n685 = Variant To Data(error in=w3121, type=w3120, Variant=w3114) -> (data=w3119:path[], error out=w3118:errorcluster)
            n686 = Set Variant Attribute(Variant=w3122, name=w3117, value=w3119, error in=w3118) -> (Variant out=w3116:variant, error out=w3115:errorcluster)  [unwired: 1 out]
          }
        }
        n687 = To Variant(anything=w3096) -> (Variant=w3097:variant)
      }
      frame "Do Averaged Datasets" {
        w3123 = FALSE ("Get(F)/Set")
        n688 = case shown="True" w3126 {
          tunnel: w3132 -> [w3140 w3149]
          tunnel: w3131 -> [w3139 w3144]
          tunnel: w3130 -> [w3138 w3148]
          tunnel: [w3137 w3142] -> w3129
          tunnel: [w3133 w3141] -> w3128
          tunnel: [w3135 w3143] -> w3127
          tunnel: w3123 -> [w3134 w3147]
          tunnel: w3125 -> [_ w3141]
          frame False {
            n689 = Get Variant Attribute(Variant=w3140, name=w3139, default value (empty Variant)=w3134, error in=w3138) -> (duplicate Variant=w3135:variant, value=w3136:bool, error out=w3137:errorcluster)  [unwired: 1 out]
            n690 = To Variant(anything=w3136) -> (Variant=w3133:variant)
          }
          frame True {
            n691 = Variant To Data(error in=w3148, type=w3147, Variant=w3141) -> (data=w3146:bool, error out=w3145:errorcluster)
            n692 = Set Variant Attribute(Variant=w3149, name=w3144, value=w3146, error in=w3145) -> (Variant out=w3143:variant, error out=w3142:errorcluster)  [unwired: 1 out]
          }
        }
        n693 = To Variant(anything=w3123) -> (Variant=w3124:variant)
      }
      frame "Destination File Path" {
        w3150 = path " "
        n694 = case shown="True" w3153 {
          tunnel: w3159 -> [w3167 w3176]
          tunnel: w3158 -> [w3166 w3171]
          tunnel: w3157 -> [w3165 w3175]
          tunnel: [w3164 w3169] -> w3156
          tunnel: [w3160 w3168] -> w3155
          tunnel: [w3162 w3170] -> w3154
          tunnel: w3150 -> [w3161 w3174]
          tunnel: w3152 -> [_ w3168]
          frame False {
            n695 = Get Variant Attribute(Variant=w3167, name=w3166, default value (empty Variant)=w3161, error in=w3165) -> (duplicate Variant=w3162:variant, value=w3163:path, error out=w3164:errorcluster)  [unwired: 1 out]
            n696 = To Variant(anything=w3163) -> (Variant=w3160:variant)
          }
          frame True {
            n697 = Variant To Data(error in=w3175, type=w3174, Variant=w3168) -> (data=w3173:path, error out=w3172:errorcluster)
            n698 = Set Variant Attribute(Variant=w3176, name=w3171, value=w3173, error in=w3172) -> (Variant out=w3170:variant, error out=w3169:errorcluster)  [unwired: 1 out]
          }
        }
        n699 = To Variant(anything=w3150) -> (Variant=w3151:variant)
      }
      frame "Process Plot Target" {
        w3177 = AlliGator_Decay_Graph_Process_Plot_Target."Single Plot"
        n700 = case shown="True" w3180 {
          tunnel: w3186 -> [w3194 w3203]
          tunnel: w3185 -> [w3193 w3198]
          tunnel: w3184 -> [w3192 w3202]
          tunnel: [w3191 w3196] -> w3183
          tunnel: [w3187 w3195] -> w3182
          tunnel: [w3189 w3197] -> w3181
          tunnel: w3177 -> [w3188 w3201]
          tunnel: w3179 -> [_ w3195]
          frame False {
            n701 = Get Variant Attribute(Variant=w3194, name=w3193, default value (empty Variant)=w3188, error in=w3192) -> (duplicate Variant=w3189:variant, value=w3190:T53, error out=w3191:errorcluster)  [unwired: 1 out]
            n702 = To Variant(anything=w3190) -> (Variant=w3187:variant)
          }
          frame True {
            n703 = Variant To Data(error in=w3202, type=w3201, Variant=w3195) -> (data=w3200:T53, error out=w3199:errorcluster)
            n704 = Set Variant Attribute(Variant=w3203, name=w3198, value=w3200, error in=w3199) -> (Variant out=w3197:variant, error out=w3196:errorcluster)  [unwired: 1 out]
          }
        }
        n705 = To Variant(anything=w3177) -> (Variant=w3178:variant)
      }
      frame "Use 1/D as Phasor Frequency" {
        w3204 = FALSE
        n706 = case shown="True" w3207 {
          tunnel: w3213 -> [w3221 w3230]
          tunnel: w3212 -> [w3220 w3225]
          tunnel: w3211 -> [w3219 w3229]
          tunnel: [w3218 w3223] -> w3210
          tunnel: [w3214 w3222] -> w3209
          tunnel: [w3216 w3224] -> w3208
          tunnel: w3204 -> [w3215 w3228]
          tunnel: w3206 -> [_ w3222]
          frame False {
            n707 = Get Variant Attribute(Variant=w3221, name=w3220, default value (empty Variant)=w3215, error in=w3219) -> (duplicate Variant=w3216:variant, value=w3217:bool, error out=w3218:errorcluster)  [unwired: 1 out]
            n708 = To Variant(anything=w3217) -> (Variant=w3214:variant)
          }
          frame True {
            n709 = Variant To Data(error in=w3229, type=w3228, Variant=w3222) -> (data=w3227:bool, error out=w3226:errorcluster)
            n710 = Set Variant Attribute(Variant=w3230, name=w3225, value=w3227, error in=w3226) -> (Variant out=w3224:variant, error out=w3223:errorcluster)  [unwired: 1 out]
          }
        }
        n711 = To Variant(anything=w3204) -> (Variant=w3205:variant)
      }
      frame "---- Decay Fit Parameter Map -----" {
      }
      frame "Decay Fit Parameter Map:Palette Information" {
        w3234 = T21 {"Palette Name [# Colors,int?,inv?]"="", "Palette Type"=0, "Palette Colors"=[], "Interpolate?"=FALSE} ("Image Display Palette Information")
        n712 = case shown="True" w3237 {
          tunnel: w3243 -> [w3251 w3260]
          tunnel: w3242 -> [w3250 w3255]
          tunnel: w3241 -> [w3249 w3259]
          tunnel: [w3248 w3253] -> w3240
          tunnel: [w3244 w3252] -> w3239
          tunnel: [w3246 w3254] -> w3238
          tunnel: w3234 -> [w3245 w3258]
          tunnel: w3236 -> [_ w3252]
          frame False {
            n713 = Get Variant Attribute(Variant=w3251, name=w3250, default value (empty Variant)=w3245, error in=w3249) -> (duplicate Variant=w3246:variant, value=w3247:T21, error out=w3248:errorcluster)  [unwired: 1 out]
            n714 = To Variant(anything=w3247) -> (Variant=w3244:variant)
          }
          frame True {
            n715 = Variant To Data(error in=w3259, type=w3258, Variant=w3252) -> (data=w3257:T21, error out=w3256:errorcluster)
            n716 = Set Variant Attribute(Variant=w3260, name=w3255, value=w3257, error in=w3256) -> (Variant out=w3254:variant, error out=w3253:errorcluster)  [unwired: 1 out]
          }
        }
        n717 = To Variant(anything=w3234) -> (Variant=w3235:variant)
      }
      frame "Decay Fit Parameter Map:Palette List" {
        w3261 = string[] []  # Decay Fit Parameter Map Palette List
        n718 = case shown="True" w3264 {
          tunnel: w3270 -> [w3278 w3287]
          tunnel: w3269 -> [w3277 w3282]
          tunnel: w3268 -> [w3276 w3286]
          tunnel: [w3275 w3280] -> w3267
          tunnel: [w3271 w3279] -> w3266
          tunnel: [w3273 w3281] -> w3265
          tunnel: w3261 -> [w3272 w3285]
          tunnel: w3263 -> [_ w3279]
          frame False {
            n719 = Get Variant Attribute(Variant=w3278, name=w3277, default value (empty Variant)=w3272, error in=w3276) -> (duplicate Variant=w3273:variant, value=w3274:string[], error out=w3275:errorcluster)  [unwired: 1 out]
            n720 = To Variant(anything=w3274) -> (Variant=w3271:variant)
          }
          frame True {
            n721 = Variant To Data(error in=w3286, type=w3285, Variant=w3279) -> (data=w3284:string[], error out=w3283:errorcluster)
            n722 = Set Variant Attribute(Variant=w3287, name=w3282, value=w3284, error in=w3283) -> (Variant out=w3281:variant, error out=w3280:errorcluster)  [unwired: 1 out]
          }
        }
        n723 = To Variant(anything=w3261) -> (Variant=w3262:variant)
      }
      frame "---- Parameter Map ----" {
      }
      frame "Parameter Map:Palette Information" {
        w3291 = T21 {"Palette Name [# Colors,int?,inv?]"="", "Palette Type"=0, "Palette Colors"=[], "Interpolate?"=FALSE} ("Image Display Palette Information")
        n724 = case shown="True" w3294 {
          tunnel: w3300 -> [w3308 w3317]
          tunnel: w3299 -> [w3307 w3312]
          tunnel: w3298 -> [w3306 w3316]
          tunnel: [w3305 w3310] -> w3297
          tunnel: [w3301 w3309] -> w3296
          tunnel: [w3303 w3311] -> w3295
          tunnel: w3291 -> [w3302 w3315]
          tunnel: w3293 -> [_ w3309]
          frame False {
            n725 = Get Variant Attribute(Variant=w3308, name=w3307, default value (empty Variant)=w3302, error in=w3306) -> (duplicate Variant=w3303:variant, value=w3304:T21, error out=w3305:errorcluster)  [unwired: 1 out]
            n726 = To Variant(anything=w3304) -> (Variant=w3301:variant)
          }
          frame True {
            n727 = Variant To Data(error in=w3316, type=w3315, Variant=w3309) -> (data=w3314:T21, error out=w3313:errorcluster)
            n728 = Set Variant Attribute(Variant=w3317, name=w3312, value=w3314, error in=w3313) -> (Variant out=w3311:variant, error out=w3310:errorcluster)  [unwired: 1 out]
          }
        }
        n729 = To Variant(anything=w3291) -> (Variant=w3292:variant)
      }
      frame "Parameter Map:Palette List" {
        w3318 = string[] []  # Parameter Map Palette List
        n730 = case shown="True" w3321 {
          tunnel: w3327 -> [w3335 w3344]
          tunnel: w3326 -> [w3334 w3339]
          tunnel: w3325 -> [w3333 w3343]
          tunnel: [w3332 w3337] -> w3324
          tunnel: [w3328 w3336] -> w3323
          tunnel: [w3330 w3338] -> w3322
          tunnel: w3318 -> [w3329 w3342]
          tunnel: w3320 -> [_ w3336]
          frame False {
            n731 = Get Variant Attribute(Variant=w3335, name=w3334, default value (empty Variant)=w3329, error in=w3333) -> (duplicate Variant=w3330:variant, value=w3331:string[], error out=w3332:errorcluster)  [unwired: 1 out]
            n732 = To Variant(anything=w3331) -> (Variant=w3328:variant)
          }
          frame True {
            n733 = Variant To Data(error in=w3343, type=w3342, Variant=w3336) -> (data=w3341:string[], error out=w3340:errorcluster)
            n734 = Set Variant Attribute(Variant=w3344, name=w3339, value=w3341, error in=w3340) -> (Variant out=w3338:variant, error out=w3337:errorcluster)  [unwired: 1 out]
          }
        }
        n735 = To Variant(anything=w3318) -> (Variant=w3319:variant)
      }
      frame "------- Local Decay Window ---------" {
      }
      frame "Local Decay Graph Window:Event Refnum" {
        w3348 = refnum<user-event> refnum  # Local Decay Graph Window Event Refnum
        n736 = case shown="True" w3351 {
          tunnel: w3357 -> [w3365 w3374]
          tunnel: w3356 -> [w3364 w3369]
          tunnel: w3355 -> [w3363 w3373]
          tunnel: [w3362 w3367] -> w3354
          tunnel: [w3358 w3366] -> w3353
          tunnel: [w3360 w3368] -> w3352
          tunnel: w3348 -> [w3359 w3372]
          tunnel: w3350 -> [_ w3366]
          frame False {
            n737 = Get Variant Attribute(Variant=w3365, name=w3364, default value (empty Variant)=w3359, error in=w3363) -> (duplicate Variant=w3360:variant, value=w3361:refnum<user-event>, error out=w3362:errorcluster)  [unwired: 1 out]
            n738 = To Variant(anything=w3361) -> (Variant=w3358:variant)
          }
          frame True {
            n739 = Variant To Data(error in=w3373, type=w3372, Variant=w3366) -> (data=w3371:refnum<user-event>, error out=w3370:errorcluster)
            n740 = Set Variant Attribute(Variant=w3374, name=w3369, value=w3371, error in=w3370) -> (Variant out=w3368:variant, error out=w3367:errorcluster)  [unwired: 1 out]
          }
        }
        n741 = To Variant(anything=w3348) -> (Variant=w3349:variant)
      }
      frame "Local Decay Graph Window:Use normalized IRF for convolution" {
        w3375 = TRUE
        n742 = case shown="True" w3378 {
          tunnel: w3384 -> [w3392 w3401]
          tunnel: w3383 -> [w3391 w3396]
          tunnel: w3382 -> [w3390 w3400]
          tunnel: [w3389 w3394] -> w3381
          tunnel: [w3385 w3393] -> w3380
          tunnel: [w3387 w3395] -> w3379
          tunnel: w3375 -> [w3386 w3399]
          tunnel: w3377 -> [_ w3393]
          frame False {
            n743 = Get Variant Attribute(Variant=w3392, name=w3391, default value (empty Variant)=w3386, error in=w3390) -> (duplicate Variant=w3387:variant, value=w3388:bool, error out=w3389:errorcluster)  [unwired: 1 out]
            n744 = To Variant(anything=w3388) -> (Variant=w3385:variant)
          }
          frame True {
            n745 = Variant To Data(error in=w3400, type=w3399, Variant=w3393) -> (data=w3398:bool, error out=w3397:errorcluster)
            n746 = Set Variant Attribute(Variant=w3401, name=w3396, value=w3398, error in=w3397) -> (Variant out=w3395:variant, error out=w3394:errorcluster)  [unwired: 1 out]
          }
        }
        n747 = To Variant(anything=w3375) -> (Variant=w3376:variant)
      }
      frame "----- Miscellaneous ----" {
      }
      frame "Misc:Skippable Dialog Windows Status" {
        w3405 = T54[] []
        n748 = case shown="True" w3408 {
          tunnel: w3414 -> [w3422 w3431]
          tunnel: w3413 -> [w3421 w3426]
          tunnel: w3412 -> [w3420 w3430]
          tunnel: [w3419 w3424] -> w3411
          tunnel: [w3415 w3423] -> w3410
          tunnel: [w3417 w3425] -> w3409
          tunnel: w3405 -> [w3416 w3429]
          tunnel: w3407 -> [_ w3423]
          frame False {
            n749 = Get Variant Attribute(Variant=w3422, name=w3421, default value (empty Variant)=w3416, error in=w3420) -> (duplicate Variant=w3417:variant, value=w3418:T54[], error out=w3419:errorcluster)  [unwired: 1 out]
            n750 = To Variant(anything=w3418) -> (Variant=w3415:variant)
          }
          frame True {
            n751 = Variant To Data(error in=w3430, type=w3429, Variant=w3423) -> (data=w3428:T54[], error out=w3427:errorcluster)
            n752 = Set Variant Attribute(Variant=w3431, name=w3426, value=w3428, error in=w3427) -> (Variant out=w3425:variant, error out=w3424:errorcluster)  [unwired: 1 out]
          }
        }
        n753 = To Variant(anything=w3405) -> (Variant=w3406:variant)
      }
    }
  }
  "Data out" <- w3
  "Error Out" <- w4
  "Default Data out" <- w1
